vi "TLB Native Dynamic Events ver 0.19a.vi"() -> ()   [LabVIEW 2018]
uses:
  Labview Training Phase 2/Enum Controls/States for Action Engine.ctl
  TLB Type Definitions/State Type Definitions, for 0.26g versions and later 2.ctl
  TLB Type Definitions/Intruction Type Definitions.ctl
  TLB Type Definitions/Encoder cluster.ctl
  TLB Type Definitions/PING CLUSTER.ctl
  <vilib>/Studica/Studica Toolkit/NavX/NavX.lvlib
  <vilib>/Studica/Studica Toolkit/Background/DIO Channel.ctl
  Underlying VI's/NavX VI/navX type def.ctl
  <vilib>/Studica/Studica Toolkit/Background/I2C Channel.ctl
  TLB Type Definitions/Vision cluster.ctl
  <vilib>/NI_Real-Time Target Support.lvlib
  TLB Type Definitions/Stepper cluster.ctl
  Experimental VI's/Archived VI's/MOTOR CONTROL NO PID Type Def.ctl
  Underlying VI's/I2C Master VI/I2C MASTER Type Def.ctl
  Underlying VI's/I2C Master VI/I2C_MASTER_WRITE_NEW Type Def.ctl
  <vilib>/userdefined/High Color/IMAQdx.ctl
  Underlying VI's/I2C Master VI/Arduino_Interfacing.ctl
  TLB Type Definitions/Yaw Cluster.ctl
  TLB Type Definitions/Time cluster.ctl
  TLB Type Definitions/Y Stepper cluster.ctl
  Underlying VI's/Modified webcam FGV/Webcam AE.ctl
  Underlying VI's/Elasped Timer/Elapsed timer control.ctl
  Underlying VI's/Motor Control VI with PID/MOTOR CONTROL WITH PID AE DATA MODE TYPE DEF.ctl
  Underlying VI's/Motor Control VI with PID/MOTOR CONTROL WITH PID AE DIRECTION TYPE DEF.ctl
  TLB Type Definitions/IR Sensor Type Def.ctl
  <vilib>/myRIO/Common/Instrument Driver Framework/myRIO v1.0/AI/typedefs/AI Channels Enum.ctl
  <vilib>/myRIO/Common/Instrument Driver Framework/myRIO v1.0/AI/typedefs/AI Channels List.ctl
  TLB Type Definitions/Motor Speed Cluster.ctl
  Underlying VI's/IMAQ Create Reference AE/IMAQ Reference AE.ctl
  TLB Type Definitions/Line Sensor Cluster.ctl
  Underlying VI's/Line Sensor AE/Line Sensor AE Type Def.ctl
  <vilib>/Utility/RT CPU Load.ctl
  <vilib>/Studica/Studica Toolkit/NavX/TypeDefs/Flags/Z900_navX_Flags_CalibrationStatusTypeDef.ctl
  <vilib>/Studica/Studica Toolkit/NavX/TypeDefs/Flags/Z900_navX_Flags_OpStatusTypeDef.ctl
panel:
  out "Distance reached?":bool
  out "Correcte stepper":u8
  out "Image Processing Error":errorcluster
  out "Object Detection":T1
  out "Status":T4 {"OP Status" items=["INITIALIZING", "SELFTEST_IN_PROGRESS", "ERROR", "IMU_AUTOCAL_IN_PROGRESS", "NORMAL"]; "Calibration Status" items=["IMU_CAL_STATE_MASK"=3, "IMU_CAL_STATE_INPROGRESS"=0, "IMU_CAL_STATE_ACCUMULATE"=1, "IMU_CAL_STATE_COMPLETE"=2]}
  out "General Errors":errorcluster
  in  "Red LED":bool
  out "Arm IR Sensor":dbl
  out "Table obstruct":bool
  out "x-y":dbl
  out "Left IR Sensor":dbl
  out "Obstacle detected":bool
  out "Speed & distance":T5
  out "Time up flag":bool
  out "Task selection":u8
  in  "Object recognition mode":enum16{"Ball", "Soap", "Gel", "Pipe", "None"}(ring)
  out "NavX Readings":T6
  out "Arduino Data":T7
  out "CPU loads":T8[](array[typedef]) {"ISR (%)" format="%#.2f"; "Idle (%)" format="%#.2f"; "Background (%)" format="%#.2f"; "Normal (%)" format="%#.2f"; "Above Normal (%)" format="%#.2f"; "High (%)" format="%#.2g"; "Timed Structures (%)" format="%#.2g"; "Time Critical (%)" format="%#.2g"; "Total (%)" format="%#.2g"}
  out "TASK ENABLE":bool
  out "Rising Edge":bool
  in  "Green LED":bool
  out "State Logic":T9=enum."Startup"
  out "elements":T10[](array[typedef])
  in  "STOP TASK":bool
  in  "OK Button":bool
  in  "STOP":bool
  out "Queue Errors":errorcluster
  out "Action Queue Items":i32
  out "State Logic Queue Items":i32
  out "Action Queues items":string[](array[string])=["Hardware reset", "Software reset", ""]
  out "Action State":string
  # "System Health Status Update"
  # "VISION"
  # "TLB FRAMEWORK STATUS"
  # "Test Programme written by Calvin Loke    Dated: 28 Aug 2019\nTest Programme revised by Dr Alex See   Dated 30 Aug 2019\n\nRevision date: 20/03/2020\nProgramme version:   TLB Native Dynamic Events ver 0.19a"
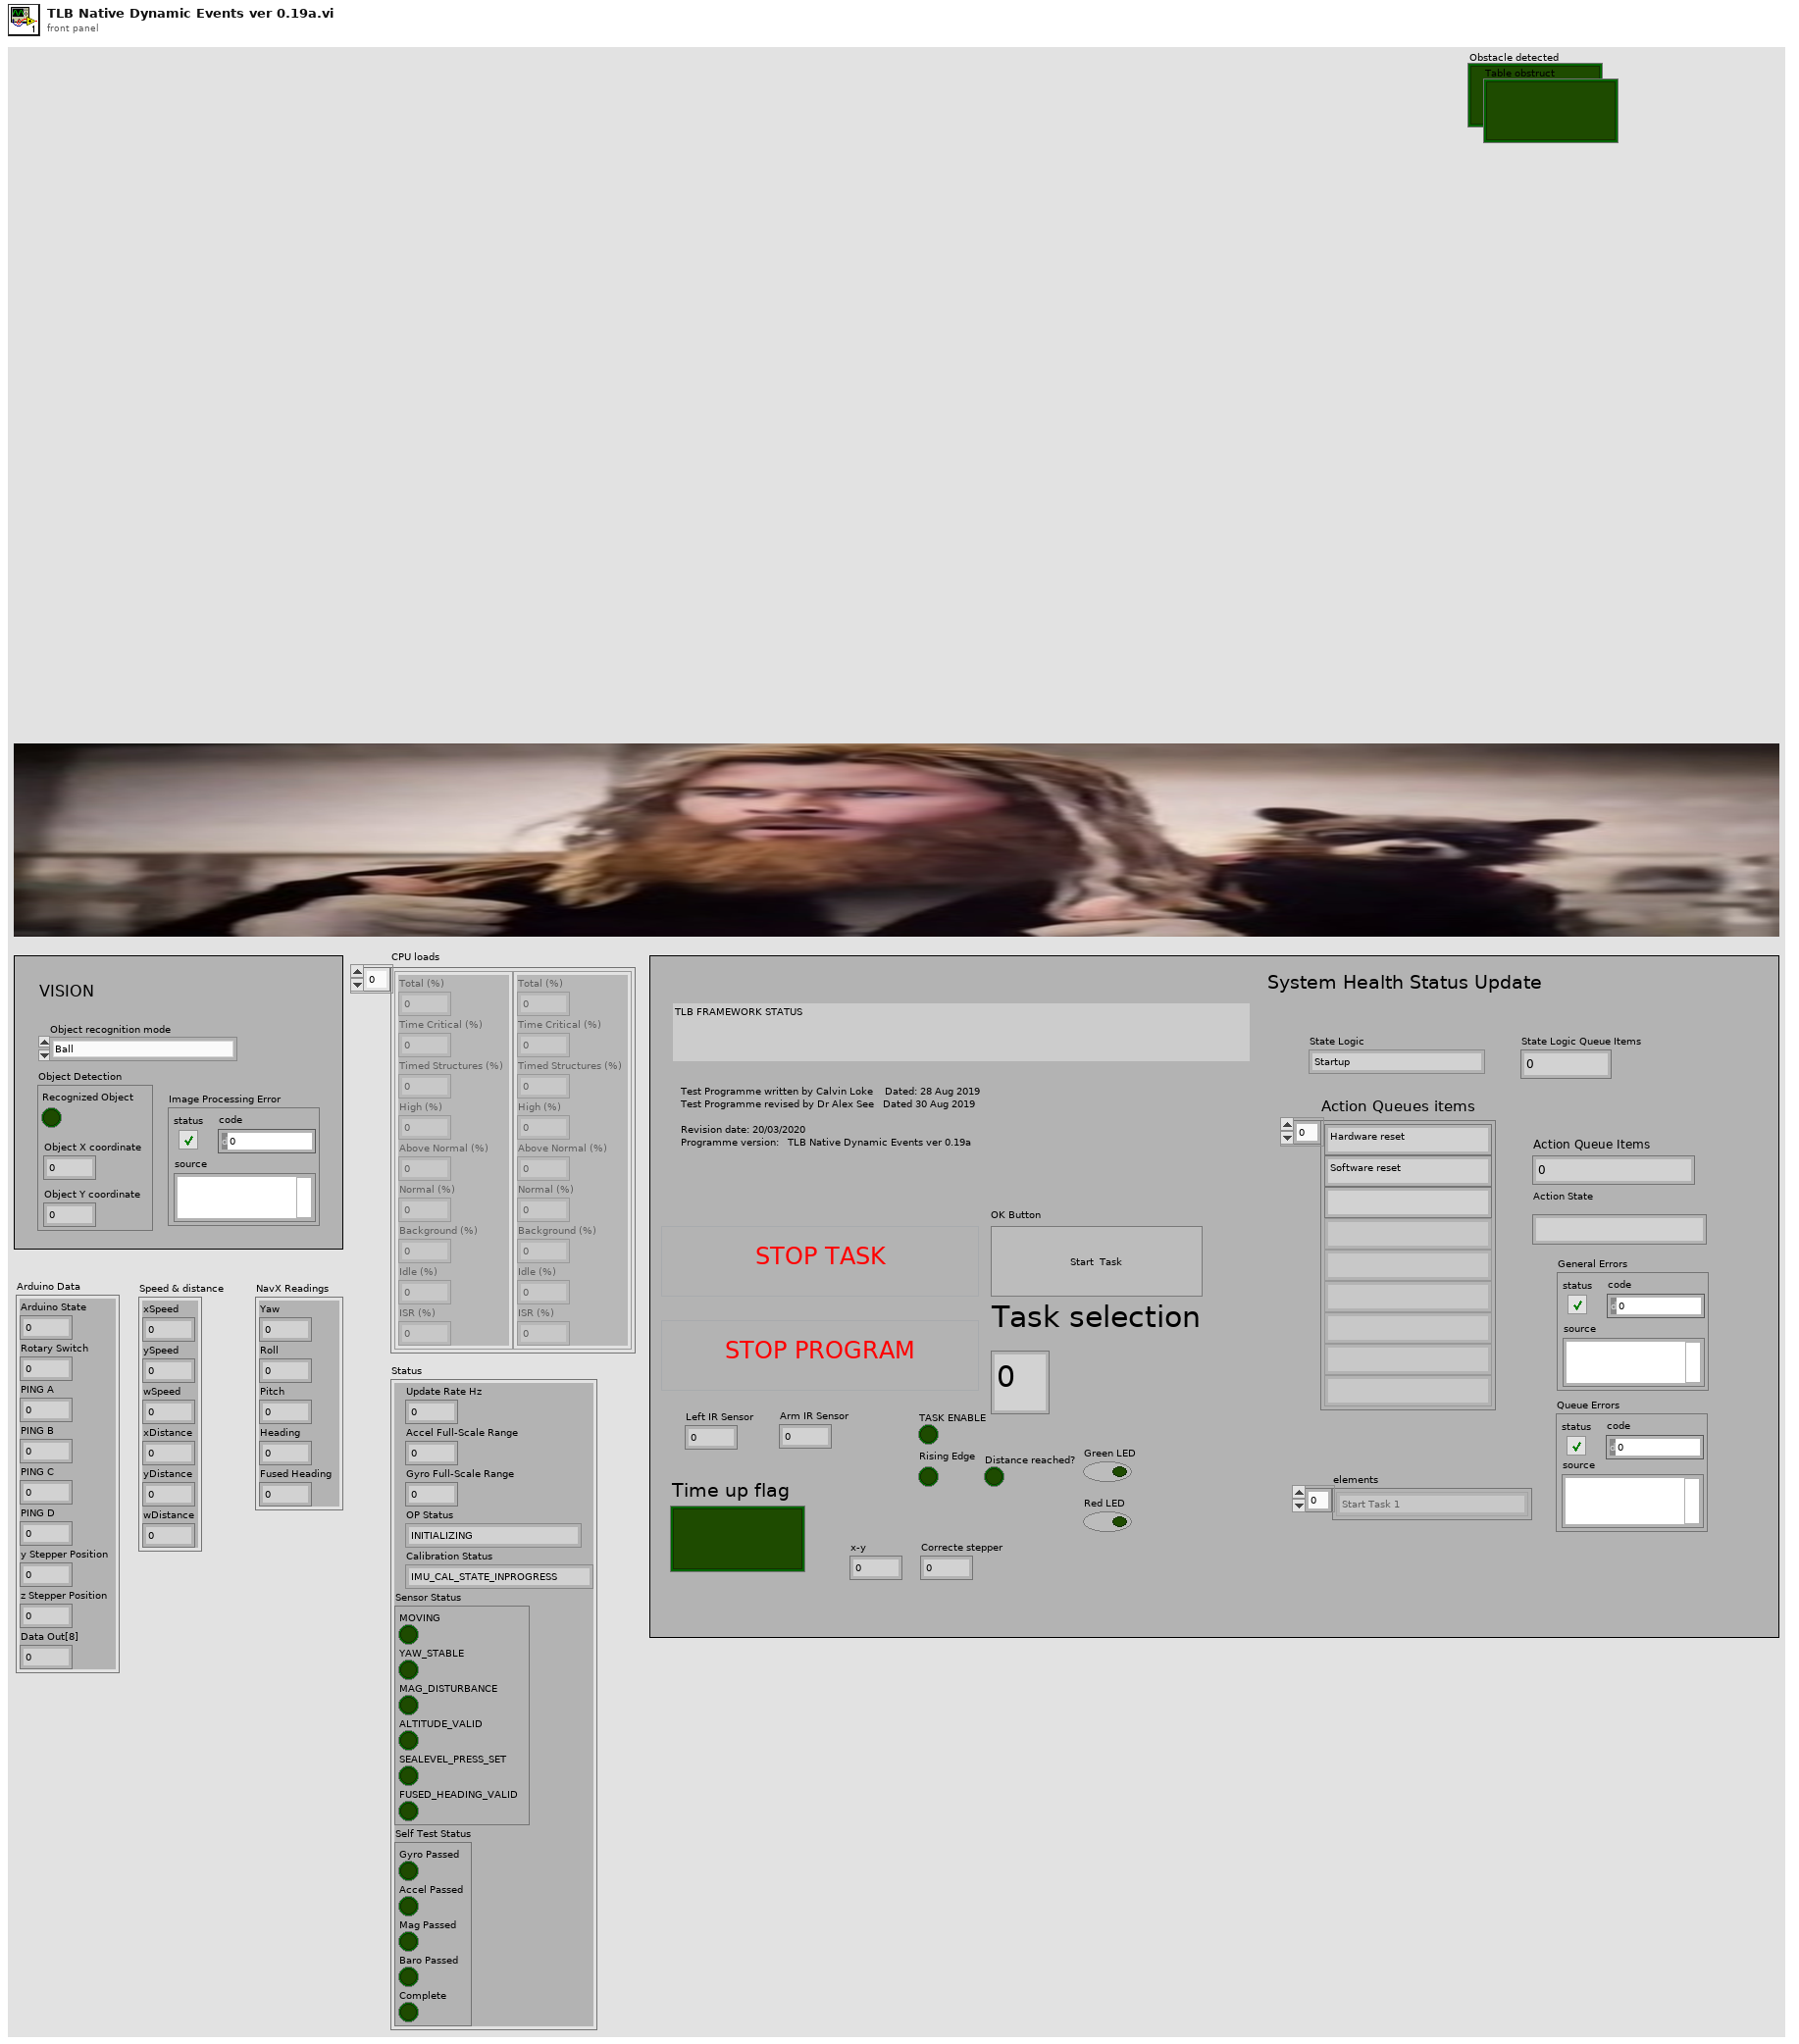
[diagram p1: front panel]
types:
  T1 = typedef "Vision cluster.ctl" = cluster{"Recognized Object":bool, "Object X coordinate":dbl, "Object Y coordinate":dbl}
  T2 = typedef "NavX.lvlib/Z900_navX_Flags_OpStatusTypeDef.ctl" = u8
  T3 = typedef "NavX.lvlib/Z900_navX_Flags_CalibrationStatusTypeDef.ctl" = u8
  T4 = cluster{"Update Rate Hz":u8, "Accel Full-Scale Range":u8, "Gyro Full-Scale Range":u16, "OP Status":T2, "Calibration Status":T3, "Sensor Status":cluster{"MOVING":bool, "YAW_STABLE":bool, "MAG_DISTURBANCE":bool, "ALTITUDE_VALID":bool, "SEALEVEL_PRESS_SET":bool, "FUSED_HEADING_VALID":bool}, "Self Test Status":cluster{"Gyro Passed":bool, "Accel Passed":bool, "Mag Passed":bool, "Baro Passed":bool, "Complete":bool}}
  T5 = cluster{"xSpeed":dbl, "ySpeed":dbl, "wSpeed":dbl, "xDistance":dbl, "yDistance":dbl, "wDistance":dbl}
  T6 = cluster{"Yaw":dbl, "Roll":dbl, "Pitch":dbl, "Heading":dbl, "Fused Heading":dbl}
  T7 = cluster{"Arduino State":u8, "Rotary Switch":u8, "PING A":u8, "PING B":u8, "PING C":u8, "PING D":u8, "y Stepper Position":u8, "z Stepper Position":u8, "Data Out[8]":u8}
  T8 = typedef "NI_Real-Time Target Support.lvlib/RT CPU Load.ctl" = cluster{"Total (%)":dbl, "Time Critical (%)":dbl, "Timed Structures (%)":dbl, "High (%)":dbl, "Above Normal (%)":dbl, "Normal (%)":dbl, "Background (%)":dbl, "Idle (%)":dbl, "ISR (%)":dbl}
  T9 = typedef "State Type Definitions, for 0.26g versions and later 2.ctl" = enum16{"None", "Startup", "Move to Angle", "True Stop", "Idle", "Shutdown", "Task 1A", "Task 1B", "Task 2:Raise Arm", "Task 2:Sensor Mode", "Task 2:Reverse Mode", "Task 3", "Task 4_A", "Task 4_B", "Task 4_C", "Task 4_D", "Task 5A", "Task 5B", "Task 5C", "Task 5D", "Task 5E: POSITION ARM", "Task 5F: ARM GRAB HEIGHT", "Task 5G: CLOSE CLAW", "Task 5H: RAISE ARM", "Task 6_A", "Task 6_B", "Task 7", "Task 8A: RAISE ARM", "Task 8B: MOVE TO BOX", "Task 8C: CAM BURST", "Task 8D: PROCESS IMAGE", "Task 8E: ROBOT ADJUST", "Task 8F: CAM BURST 2", "Task 8G: PROCESS IMAGE 2", "Task 8H: ARM ADJUST", "Task 8I: ARM GRAB HEIGHT", "Task 8J: CLOSE CLAW", "Task 8K: RAISE MY SWORD", "Task 9A: Raise Arm", "Task 9B: Rotate to Angle", "Task 9C: Detect Box", "Task 9D: MOVE FORWARD", "Task 9E: MOVE LEFT", "Task 9F: SCAN BOX", "Task 9G: MOVE RIGHT", "Task 9H: SCAN BOX 2", "Task 9I: ROTATE 90 CW", "Task 9J: FORWARD", "Task 9K: MOVE RIGHT", "Task 9L: SCAN BOX 3", "Task 9M: MOVE RIGHT", "Task 9N: SCAN BOX 4", "PENIS", "PENIS 2", "PENIS 3", "Task 9R: PROCESS COLOUR", "Task A1: Task 9 Open cam", "Task A2: Task 9 Move Arm", "Task A3: Task 9 Set Timer", "Task A4: Tasl 9 Capture images", "Task A5: Task 9 Close camera", "Task A6: Process Colour", "Task A7: Dispose Camera Buffer"}
  T10 = typedef "Intruction Type Definitions.ctl" = enum16{"None", "Start Task 1", "Start Task 2", "Start Task 3", "Start Task 4", "Start Task 5", "Start Task 6", "Start Task 7", "Start Task 8 - BALL", "Start Task 8 - Gel", "Start Task 8 - Pipe", "Start Task 8 - Soap", "Start Task 9", "Start Task A", "Start Task B", "Exit"}
  T11 = typedef "Line Sensor Cluster.ctl" = cluster{"Line Detected?":bool, "S1":dbl, "S2":dbl, "S3":dbl, "S4":dbl}
  T12 = typedef "Motor Speed Cluster.ctl" = cluster{"ySpeed":dbl, "xSpeed":dbl, "wSpeed":dbl}
  T13 = typedef "IR Sensor Type Def.ctl" = cluster{"Left IR Sensor":dbl, "Arm IR Sensor":dbl, "Bottom IR Sensor":dbl}
  T14 = typedef "Y Stepper cluster.ctl" = cluster{"yStepper desired":u8}
  T15 = typedef "Time cluster.ctl" = cluster{"Time up flag":bool, "SET TIME TO CHECK":dbl}
  T16 = typedef "Yaw Cluster.ctl" = cluster{"Yaw":dbl, "Compass":dbl}
  T17 = typedef "Stepper cluster.ctl" = cluster{"y Stepper Position":u8, "z Stepper Position":u8}
  T18 = typedef "DIO Channel.ctl" = enum16{"Not Connected", "A/DIO1", "A/DIO2", "A/DIO3", "A/DIO4", "A/DIO5", "A/DIO6", "A/DIO7", "A/DIO13", "B/DIO1", "B/DIO2", "B/DIO3", "B/DIO4", "B/DIO5", "B/DIO6", "B/DIO7", "B/DIO13", "C/DIO0", "C/DIO1", "C/DIO2", "C/DIO3", "C/DIO4", "C/DIO5", "C/DIO6", "C/DIO7"}
  T19 = typedef "PING CLUSTER.ctl" = cluster{"PING_A":u8, "PING_B":u8, "PING_C":u8, "PING_D":u8}
  T20 = typedef "Encoder cluster.ctl" = cluster{"xDistance":dbl, "yDistance":dbl, "wDistance":dbl}
  T21 = cluster{"DIO Channel":T18, "FPGA VI Reference Out":refnum<k20>}
  T22 = typedef "navX type def.ctl" = enum16{"Get i2C reference", "Read Values", "Zero Yaw"}
  T23 = typedef "Arduino_Interfacing.ctl" = enum16{"Initialize", "Write to Arduino", "Read From Arduino"}
  T24 = typedef "I2C Channel.ctl" = enum16{"Not Connected", "A", "B"}
  T25 = typedef "States for Action Engine.ctl" = enum16{"Initialize", "Write", "Read"}
  T26 = cluster{"I2C Ref Out":cluster{"I2C Channel":T24, "FPGA VI Reference Out":refnum<k20>}, "Connected":bool, "Slave Address (7-bit)":u8, "Registry":u8[]}
  T27 = typedef "State Type Definitions.ctl" = enum16{"None", "Startup", "Move to Angle", "True Stop", "Idle", "Shutdown", "Task 1", "Task 2:Raise Arm", "Task 2:Sensor Mode", "Task 2:Reverse Mode", "Task 3", "Task 4_A", "Task 4_B", "Task 4_C", "Task 4_D", "Task 5A: ARM CAM HEIGHT", "Task 5B: MOVE TO BOX", "Task 5C: CAM BURST", "Task 5D: PROCESS IMAGE", "Task 5E: POSITION ARM", "Task 5F: ARM GRAB HEIGHT", "Task 5G: CLOSE CLAW", "Task 5H: RAISE ARM", "Task 6_A", "Task 6_B", "Task 7", "Task 8A: RAISE ARM", "Task 8B: MOVE TO BOX", "Task 8C: CAM BURST", "Task 8D: PROCESS IMAGE", "Task 8E: ROBOT ADJUST", "Task 8F: CAM BURST 2", "Task 8G: PROCESS IMAGE 2", "Task 8H: ARM ADJUST", "Task 8I: ARM GRAB HEIGHT", "Task 8J: CLOSE CLAW", "Task 8K: RAISE MY SWORD", "Task 9A: Raise Arm", "Task 9B: Rotate to Angle", "Task 9C: Rotation alignmnet", "Task 9D: Move Forward", "Task 9E: MOVE LEFT", "Task A: RAISE ARM TO HEIGHT", "Task A: MOVE FORWARD"}
  T28 = typedef "MOTOR CONTROL WITH PID AE DIRECTION TYPE DEF.ctl" = enum16{"y-axis movement", "x-axis movement", "rotation", "stop", "reset encoders"}
  T29 = typedef "MOTOR CONTROL WITH PID AE DATA MODE TYPE DEF.ctl" = enum16{"Init AE", "Write to AE", "Read from AE"}
  T30 = typedef "Line Sensor AE Type Def.ctl" = enum16{"INIT AE", "READ FROM LINE SENSORS"}
  T31 = typedef "IMAQ Reference AE.ctl" = enum16{"Initialize AE", "Get IMAQ Reference", "Dispose Processing Buffer"}
  T32 = typedef "Elapsed timer control.ctl" = enum16{"Start", "Pause", "Initialize"}
  T33 = typedef "I2C_MASTER_WRITE_NEW Type Def.ctl" = enum16{"Ultrasonic sensors", "Stepper origin", "zStepper 13.3k", "zStepper 13k", "zStepper 12k", "zStepper 11k", "zStepper 10k", "zStepper 9k", "zStepper 8k", "zStepper 7k", "zStepper 6k", "zStepper 5k", "zStepper 4k", "zStepper 3k", "zStepper 2k", "zStepper 1k", "zStepper 900", "zStepper 800", "zStepper 700", "zStepper 600", "zStepper 500", "zStepper 400", "zStepper 300", "zStepper 200", "zStepper 100", "zStepper 0", "yStepper control", "Open Claw", "Close Claw", "Soft Reset"}
  T34 = typedef "Webcam AE.ctl" = enum16{"Initialize Camera", "Open Camera", "Continuous Acquisition", "Close Camera", "Retrieve Image", "Dispose Camera Image Buffer"}
  T35 = typedef "IMAQdx.ctl" = refnum<k21>
  T36 = typedef "MOTOR CONTROL NO PID Type Def.ctl" = enum16{"Init", "Front Back", "Left Right", "Rotate", "Stop", "Latch"}
  T37 = typedef "AI Channels List.ctl" = T38[]
  T38 = typedef "AI Channels Enum.ctl" = enum16{"Not Connected", "AudioIn/Left", "AudioIn/Right", "C/AI0", "C/AI1", "A/AI0", "A/AI1", "A/AI2", "A/AI3", "A/AI4", "A/AI5", "A/AI6", "A/AI7", "B/AI0", "B/AI1", "B/AI2", "B/AI3", "B/AI4", "B/AI5", "B/AI6", "B/AI7", "AI/AI0", "AI/AI1", "AI/AI2", "AI/AI3", "A/AI0 (DIFF)", "A/AI1 (DIFF)", "A/AI2 (DIFF)", "A/AI3 (DIFF)", "B/AI0 (DIFF)", "B/AI1 (DIFF)", "B/AI2 (DIFF)", "B/AI3 (DIFF)"}
  T39 = cluster{"S1":dbl, "S2":dbl, "S3":dbl, "S4":dbl, "Array[4]":dbl, "Array[5]":dbl, "Array[6]":dbl, "Array[7]":dbl, "Array[8]":dbl}
  T40 = typedef "I2C MASTER Type Def.ctl" = enum16{"Last State", "Mode 0", "Mode 1", "Mode 2", "Mode 3", "Mode 4", "Mode 5", "Mode 6", "Mode 7", "Mode 8", "Mode 9", "Mode 10"}
  T41 = typedef "IMAQ Image.ctl" = refnum<image>
  T42 = cluster{"Number of Matches":i32, "Object detected?":bool}
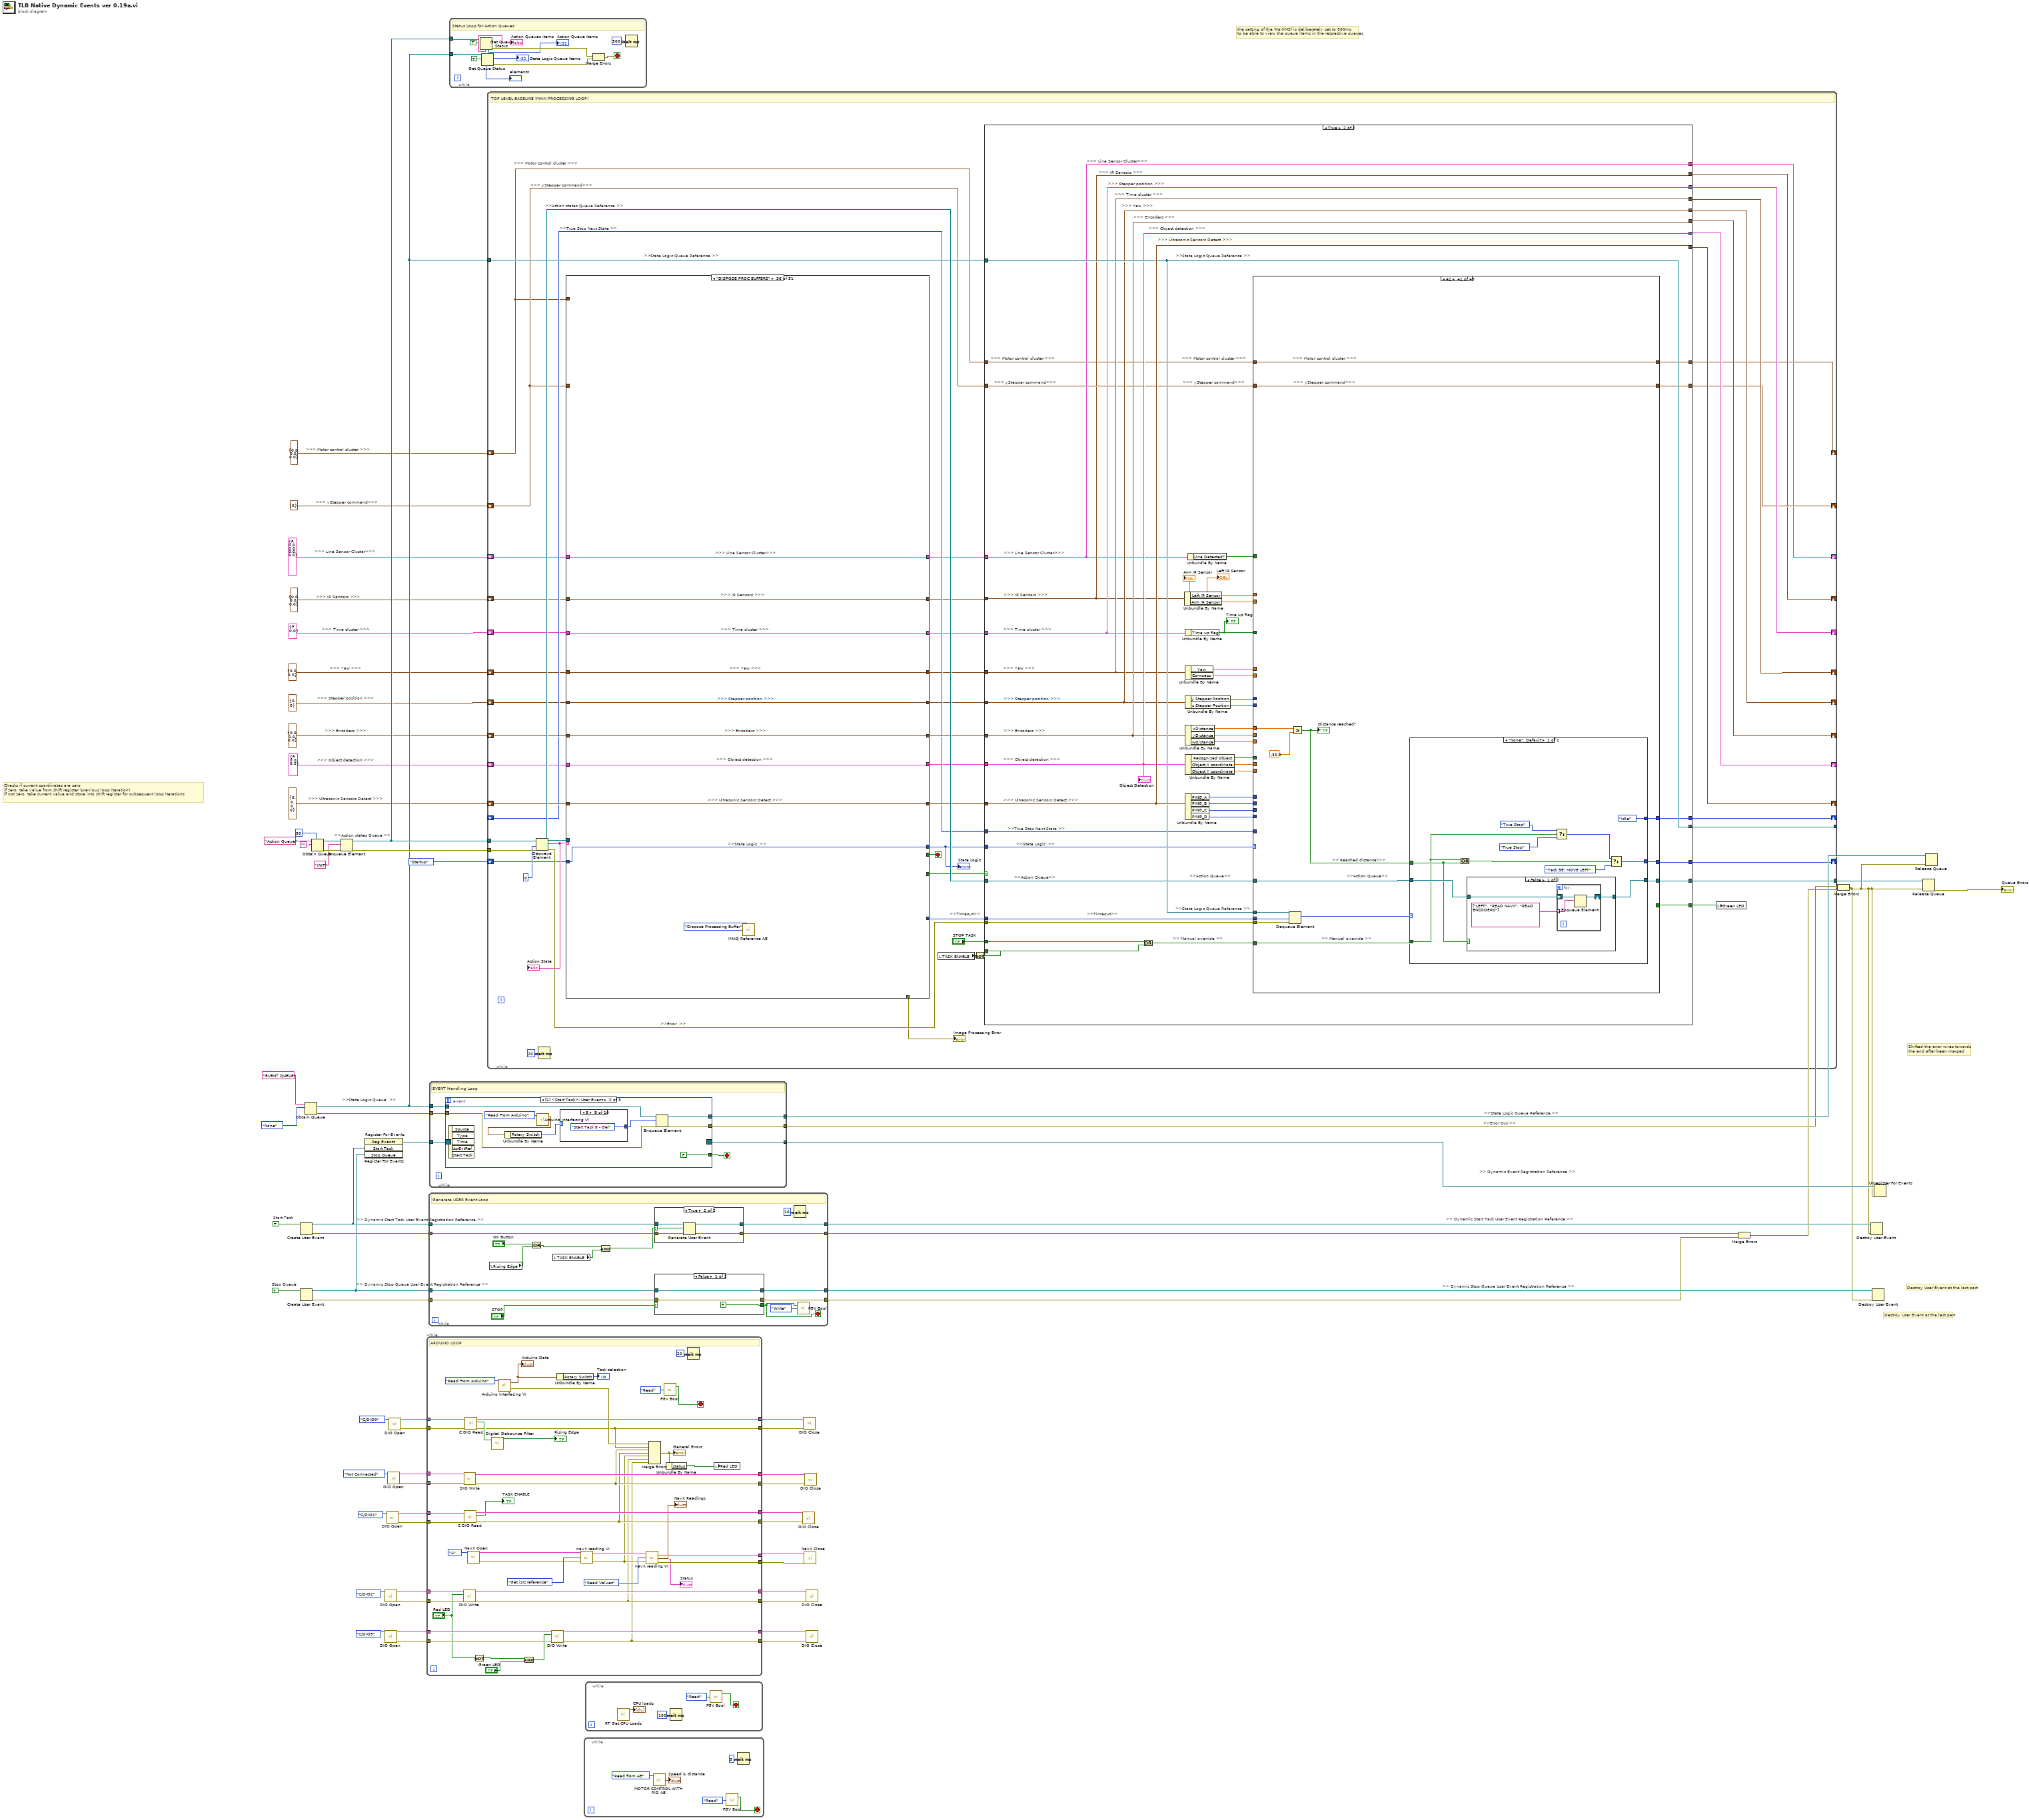
[diagram p0: block diagram]
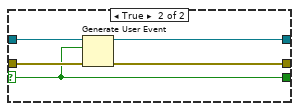
[diagram p2: hidden frame]
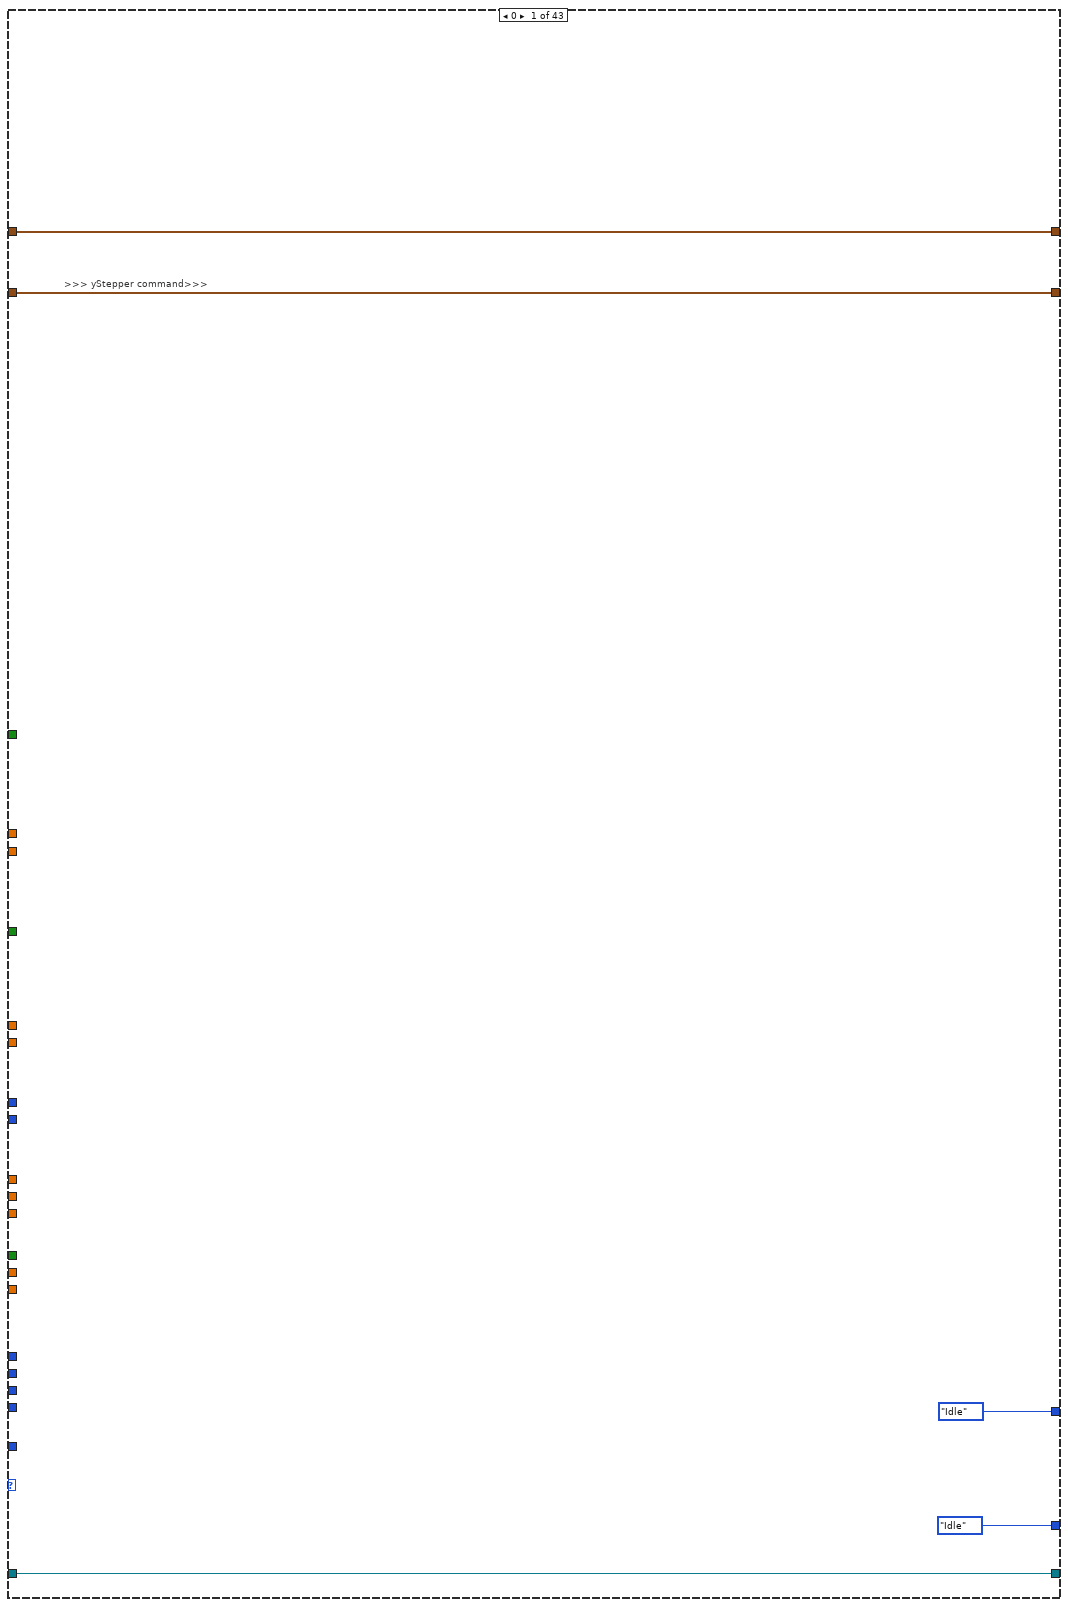
[diagram p5: hidden frame]
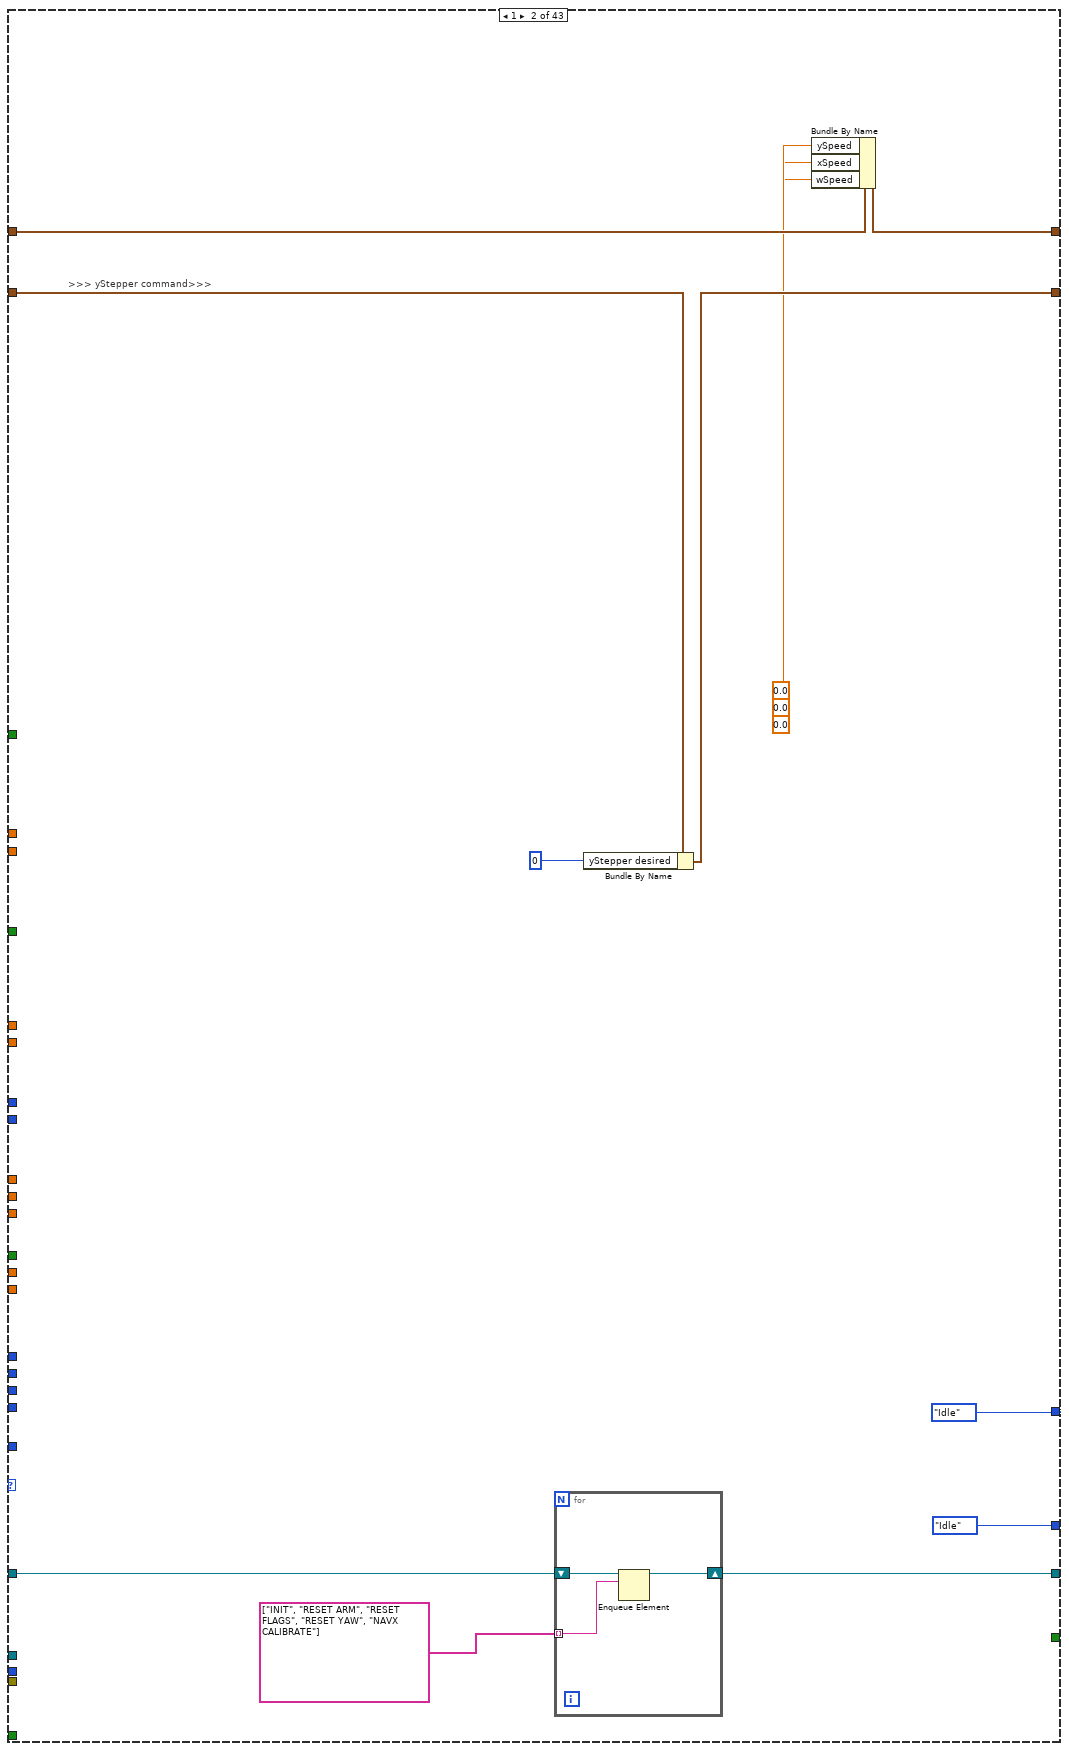
[diagram p6: hidden frame]
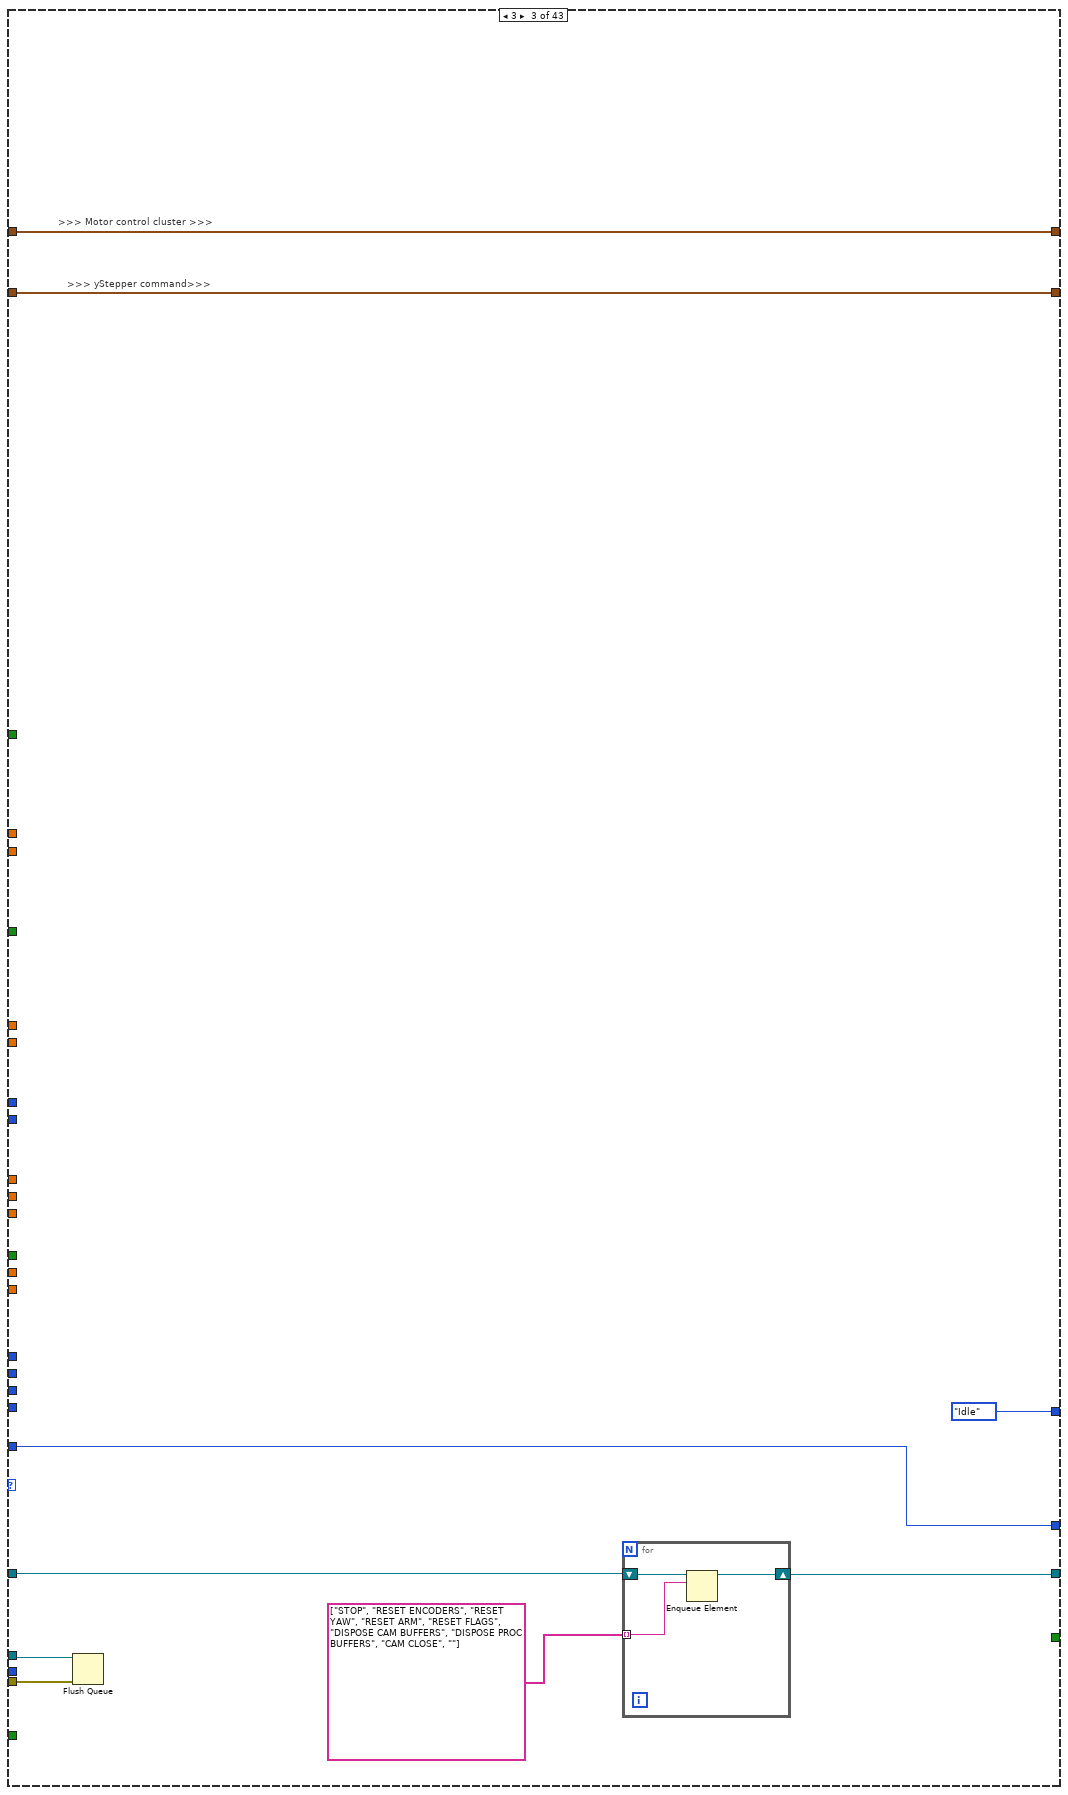
[diagram p7: hidden frame]
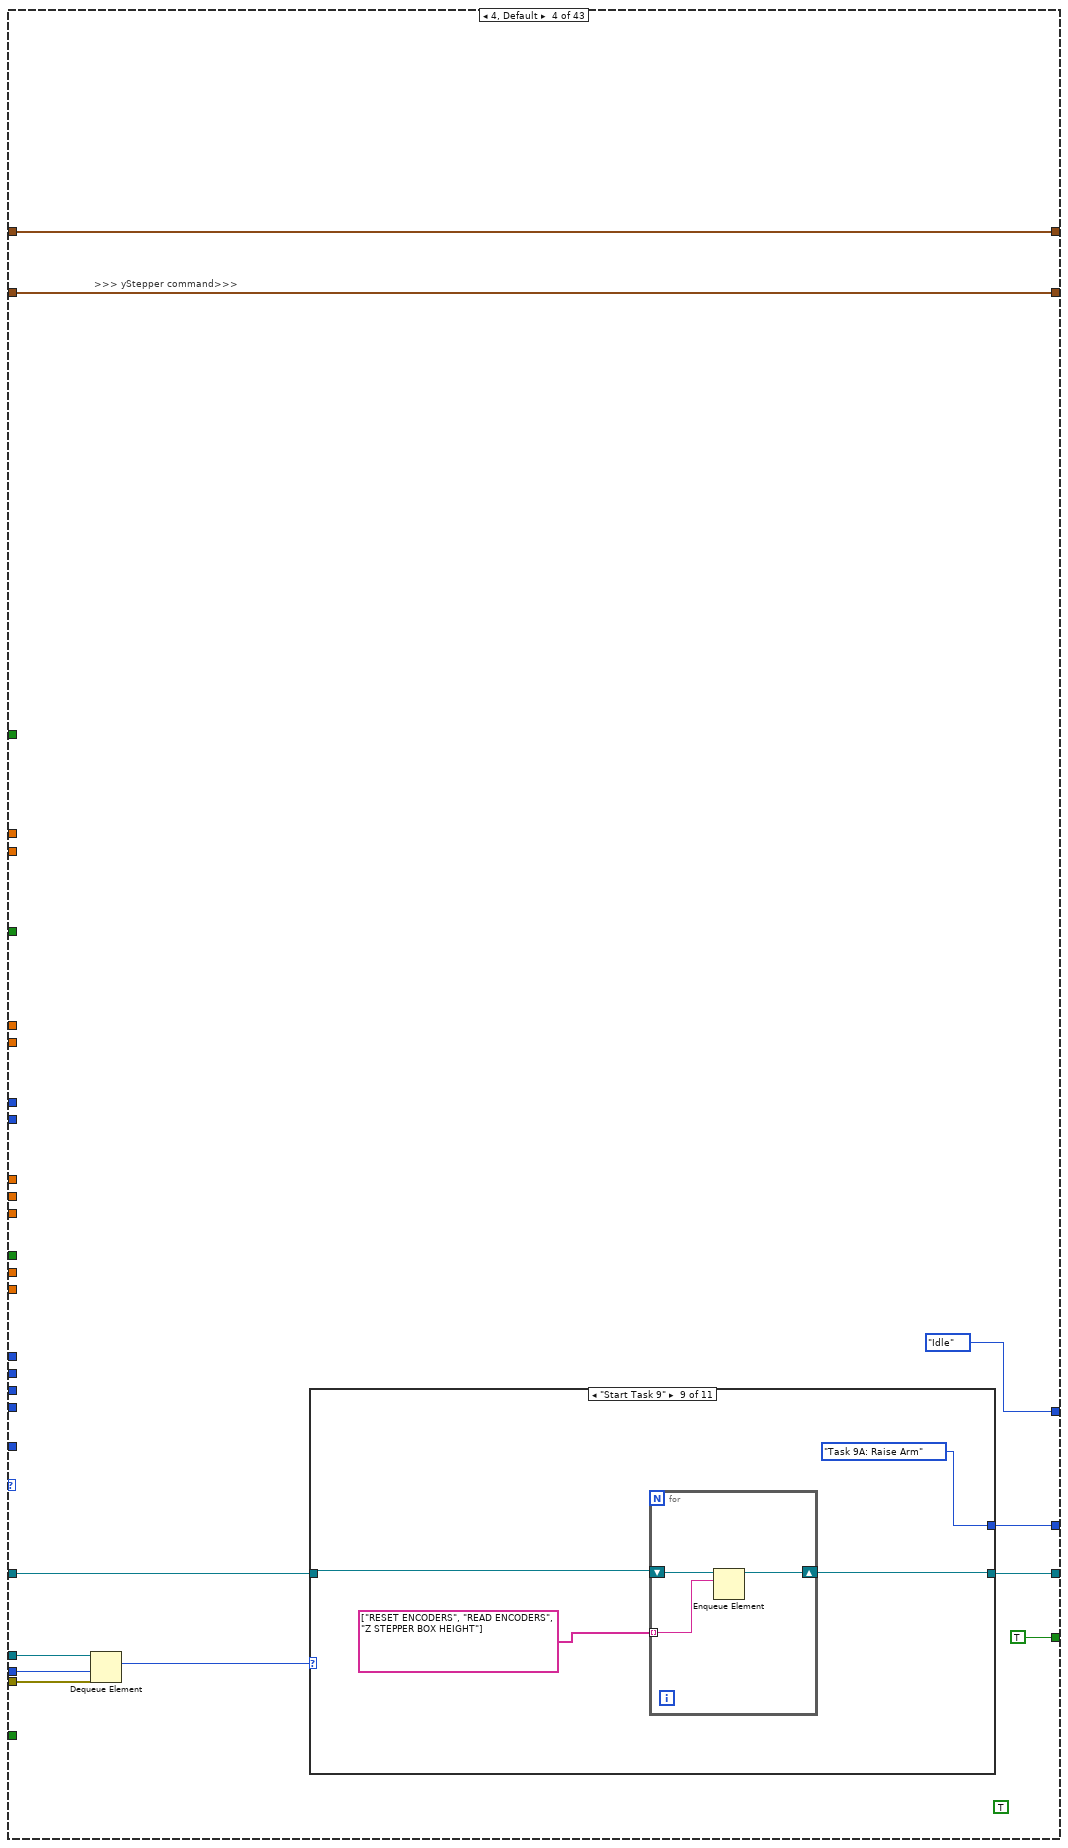
[diagram p8: hidden frame]
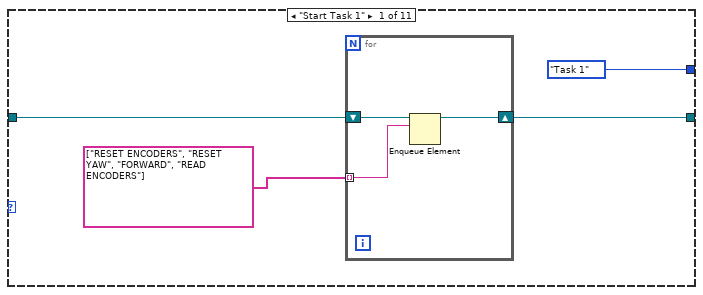
[diagram p9: hidden frame]
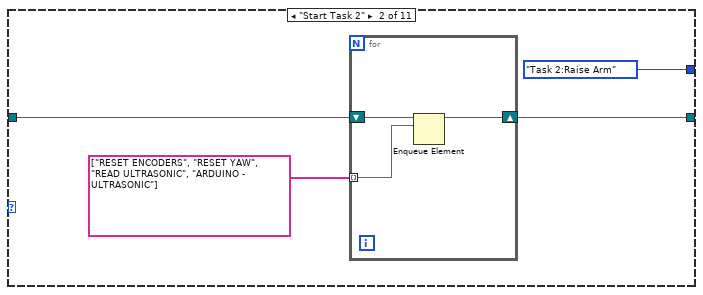
[diagram p10: hidden frame]
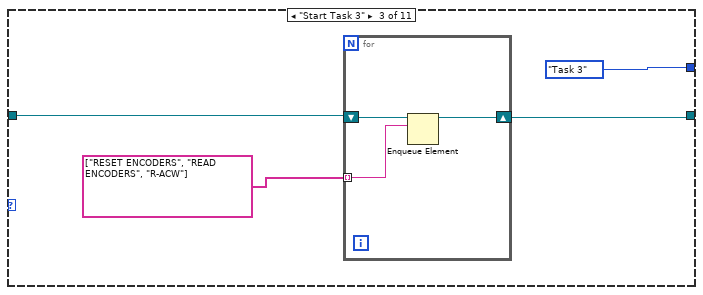
[diagram p11: hidden frame]
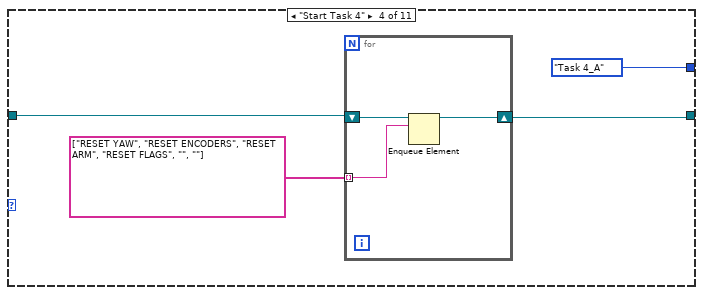
[diagram p12: hidden frame]
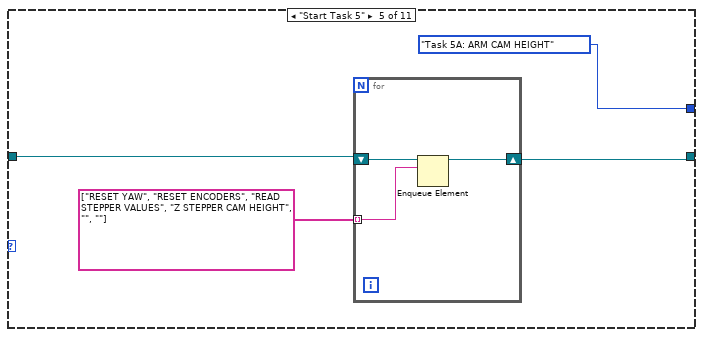
[diagram p13: hidden frame]
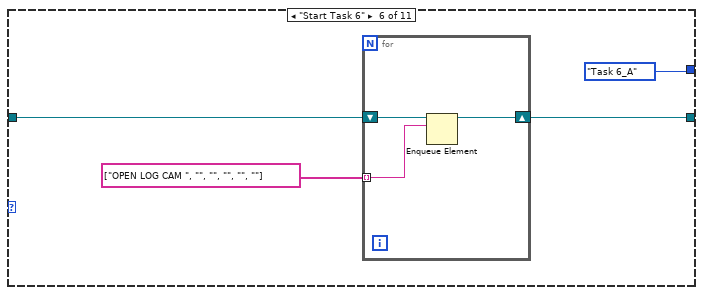
[diagram p14: hidden frame]
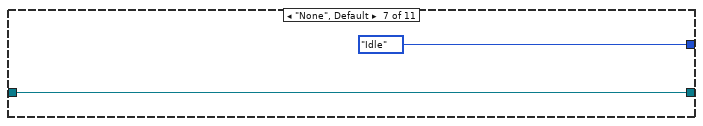
[diagram p15: hidden frame]
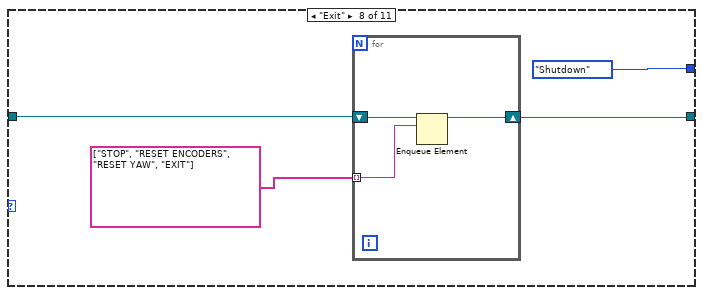
[diagram p16: hidden frame]
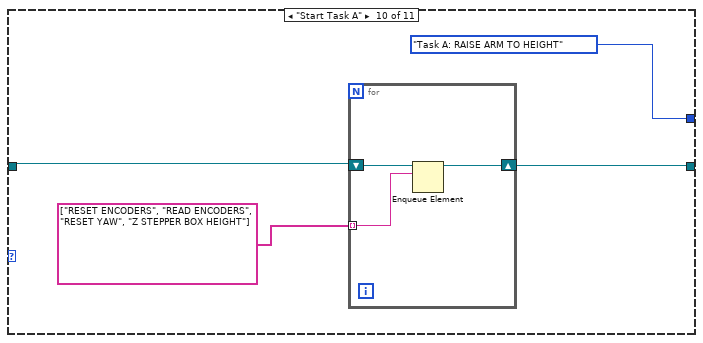
[diagram p17: hidden frame]
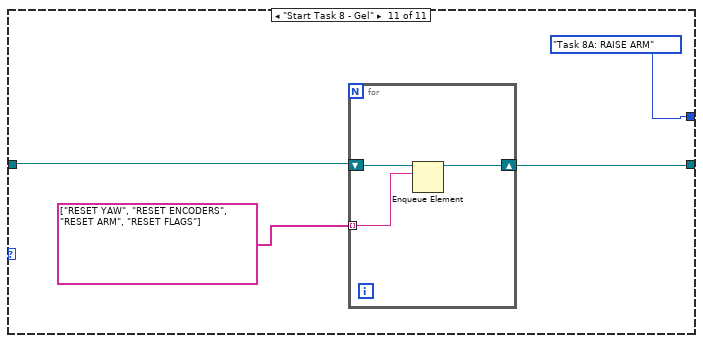
[diagram p18: hidden frame]
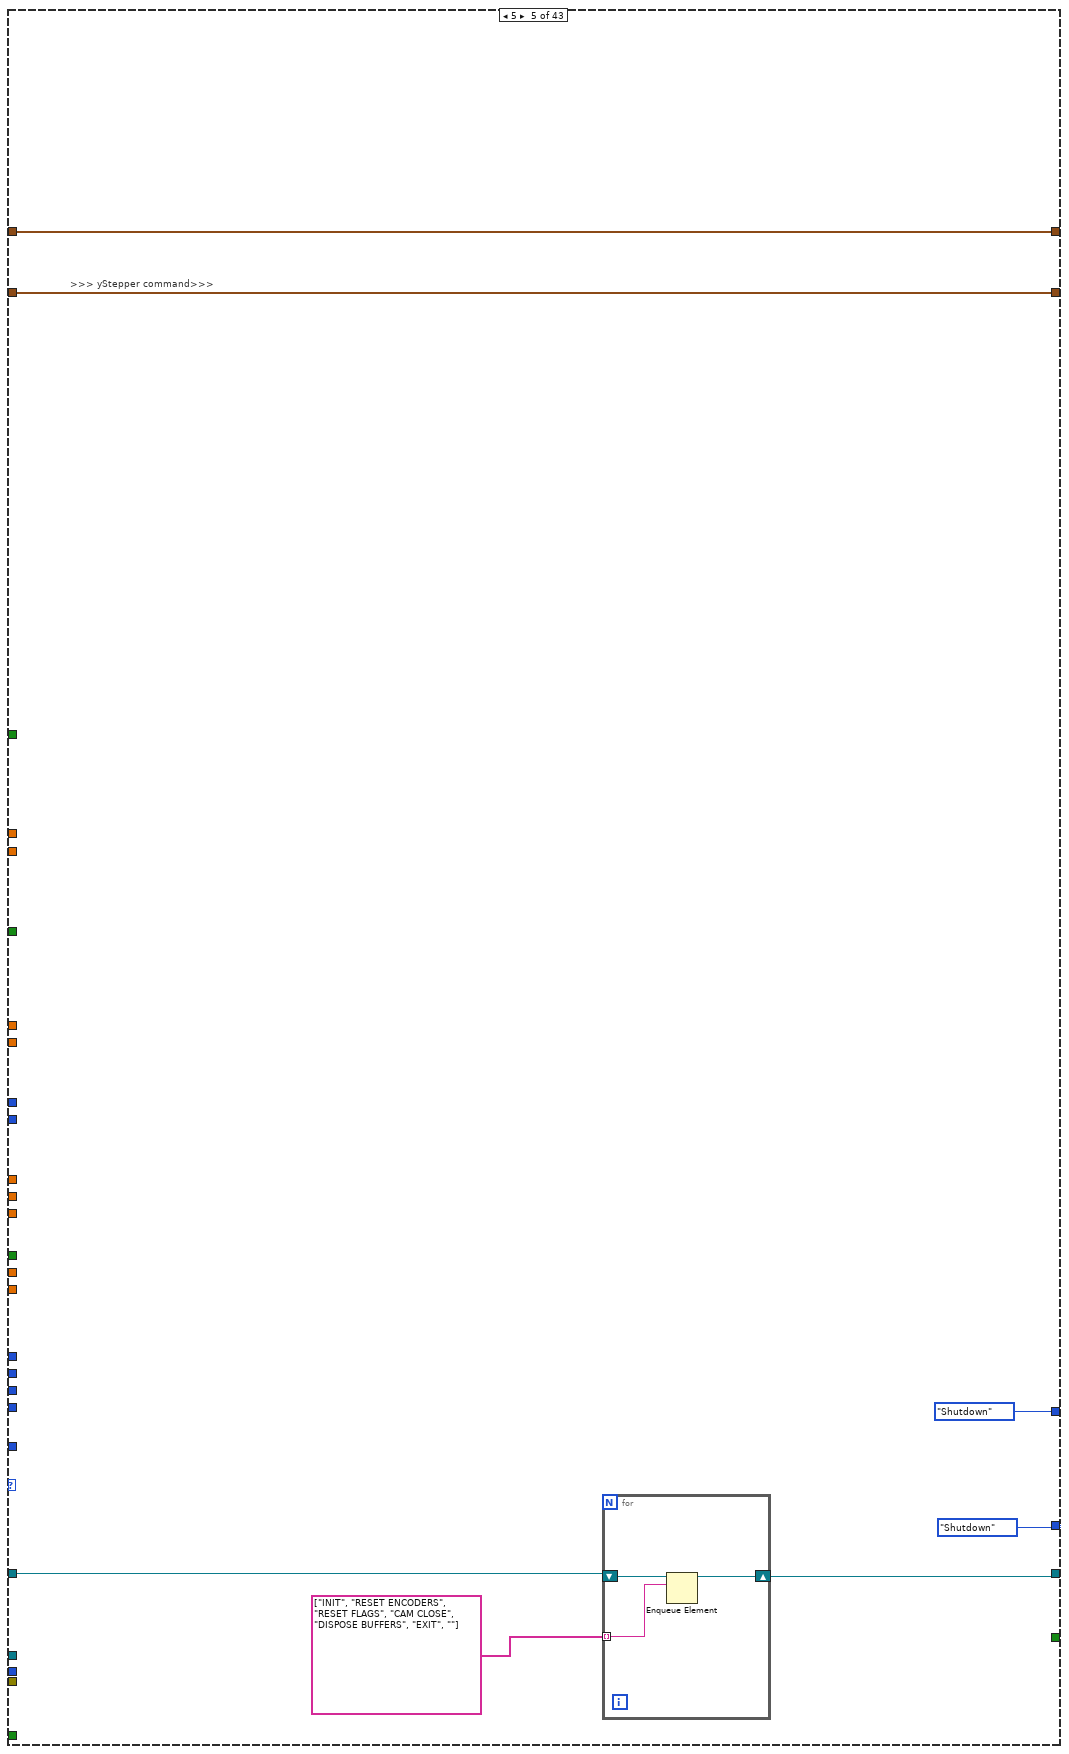
[diagram p19: hidden frame]
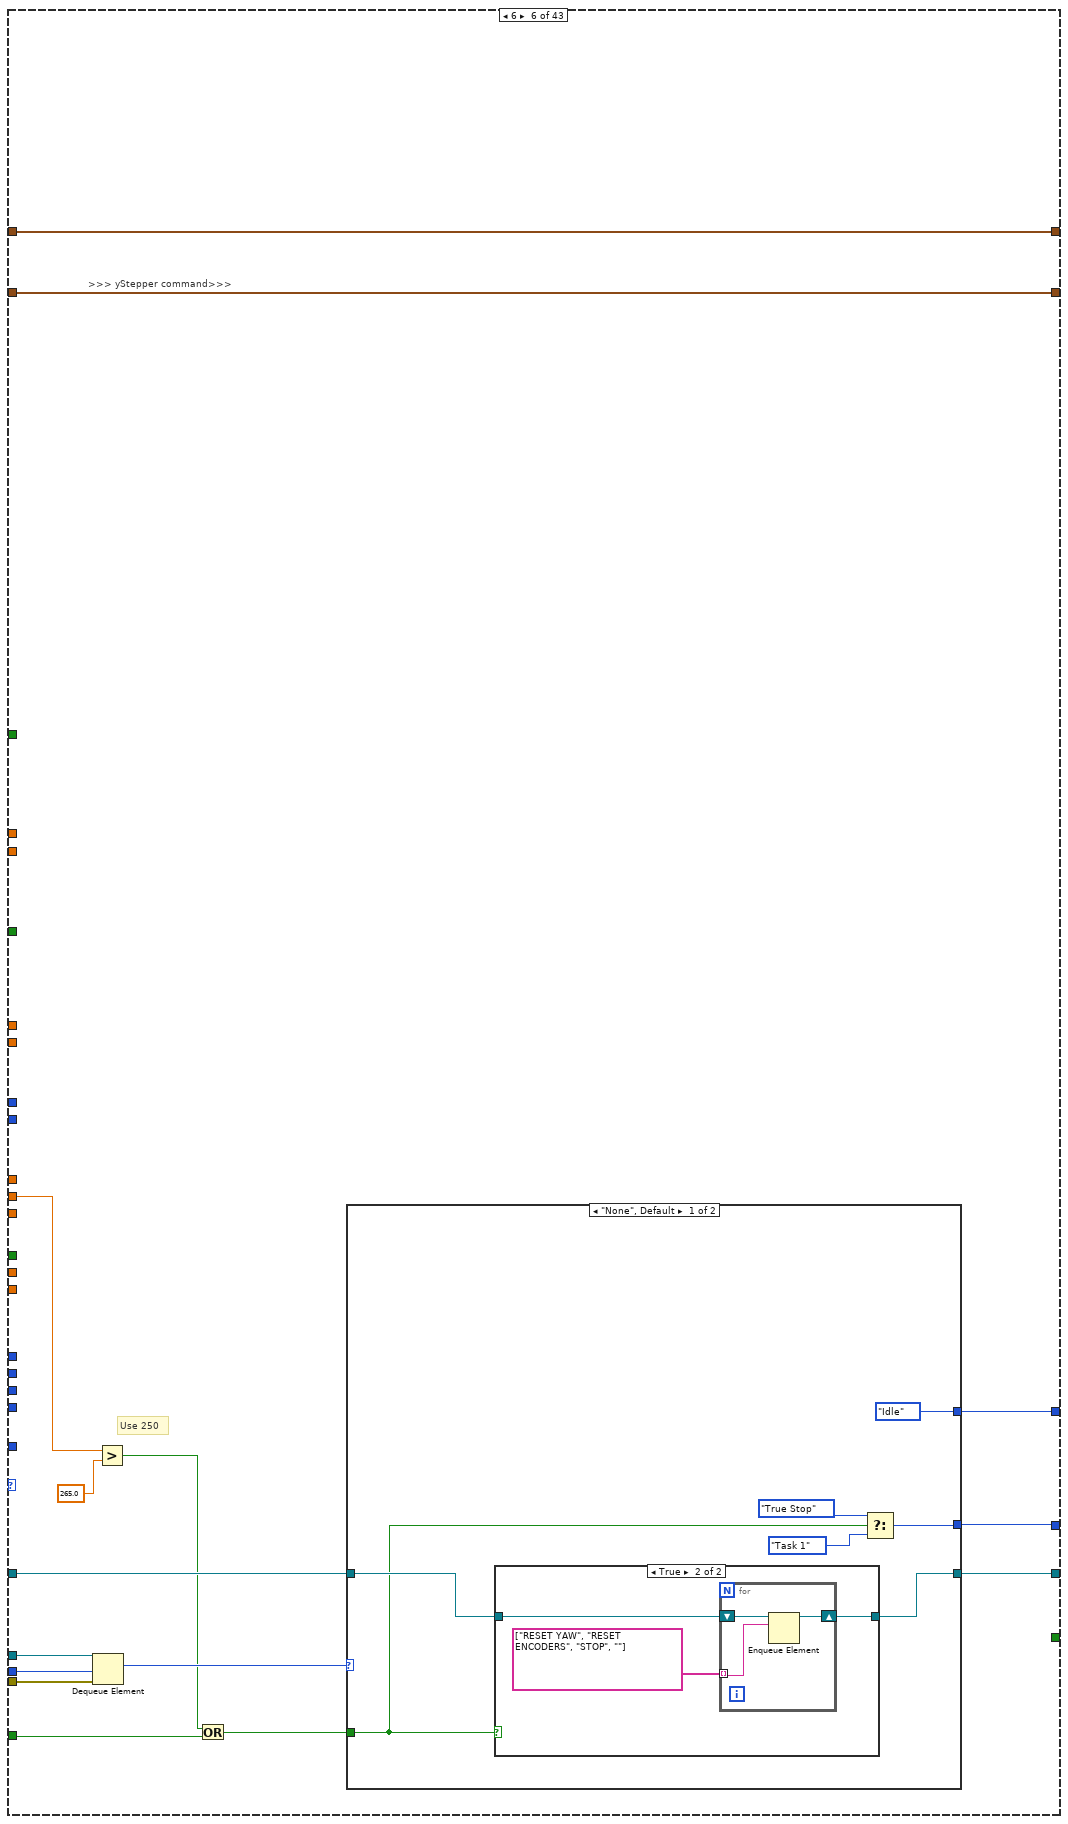
[diagram p20: hidden frame]
diagram:
  w68 = TRUE  # Stop Queue
  w67 = TRUE  # Start Task
  # ">>> Line Sensor Cluster>>>"
  # ">>> Motor control cluster >>>"
  # ">>> IR Sensors >>>"
  # "Checks if current coordinates are zero\nif zero, take value from shift register (previous loop iteration)\nif not zero, take current value and store into shift register for subsequent loop iterations"
  # ">>> yStepper command>>>"
  # ">>> Time cluster >>>"
  # ">>> Yaw >>>"
  # ">>> Stepper position >>>"
  # ">>> Encoders >>>"
  # ">>> Object detection >>>"
  # ">>> Ultrasonic Sensors Detect >>>"
  # "the setting of the Wait(MS) is deliberately set to 500ms\nto be able to view the queue items in the respective queues"
  # ">>Error Out >>"
  # ">> Dynamic Stop Queue User Event Registration Reference >>"
  # ">> Dynamic Start Task User Event Registration Reference >>"
  # ">> Dynamic Stop Queue User Event Registration Reference >>"
  # ">> Dynamic Start Task User Event Registration Reference >>"
  # ">> Dynamic Event Registration Reference >>"
  # ">>Action states Queue >>"
  # ">>State Logic Queue  >>"
  # ">>State Logic Queue Reference >>"
  # "Destroy User Event at the last part"
  # "Destroy User Event at the last part"
  # "Shifted the error wires towards\nthe end after been merged"
  n1 = Create User Event(user event datatype=w67) -> (user event=w59:refnum<user-event>, error out=w64:errorcluster)  [unwired: 1 in]
  n2 = Create User Event(user event datatype=w68) -> (user event=w60:refnum<user-event>, error out=w63:errorcluster)  [unwired: 1 in]
  n3 = Obtain Queue(name (unnamed)="EVENT QUEUE", element data type=Intruction_Type_Definitions."None" ("Enum")) -> (queue out=w45:refnum<queue>, error out=w51:errorcluster)  [unwired: 3 in, 1 out]
  n4 = Obtain Queue(max queue size (-1, unlimited)=50, name (unnamed)="Action Queue", element data type="") -> (queue out=w54:refnum<queue>, error out=w50:errorcluster)  [unwired: 2 in, 1 out]
  n5 = Enqueue Element(queue=w54, element="INIT", error in (no error)=w50) -> (queue out=w46:refnum<queue>, error out=w49:errorcluster)  [unwired: 1 in, 1 out]
  n6 = register-events "Register For Events"(w59, w60) -> (reference out=w58:refnum<event-registration>)  [unwired: 2 in, 1 out]
  n7 = call <vilib>:"DIO Open.vi"("DIO Channel"=DIO_Channel."C/DIO2") -> ("error out"=w18:errorcluster, "DIO Info Out"=w19:T21)  [unwired: 9 in]
  n8 = call <vilib>:"DIO Open.vi"("DIO Channel"=DIO_Channel."C/DIO3") -> ("error out"=w13:errorcluster, "DIO Info Out"=w14:T21)  [unwired: 9 in]
  n9 = call <vilib>:"DIO Open.vi"("DIO Channel"=DIO_Channel."C/DIO1") -> ("error out"=w23:errorcluster, "DIO Info Out"=w24:T21)  [unwired: 9 in]
  n10 = call <vilib>:"DIO Open.vi"("DIO Channel"=DIO_Channel."Not Connected") -> ("error out"=w28:errorcluster, "DIO Info Out"=w30:T21)  [unwired: 9 in]
  n11 = call <vilib>:"DIO Open.vi"("DIO Channel"=DIO_Channel."C/DIO0") -> ("error out"=w33:errorcluster, "DIO Info Out"=w36:T21)  [unwired: 9 in]
  n12 = while {
    tunnel: w36 -> [w112]
    tunnel: [w111] -> w34
    tunnel: w33 -> [w110]
    tunnel: [w81] -> w32
    tunnel: w30 -> [w107]
    tunnel: [w106] -> w29
    tunnel: w28 -> [w105]
    tunnel: [w80] -> w27
    tunnel: [w104] -> w25
    tunnel: w24 -> [w103]
    tunnel: w23 -> [w102]
    tunnel: [w79] -> w22
    tunnel: w19 -> [w96]
    tunnel: w18 -> [w95]
    tunnel: [w94] -> w17
    tunnel: [w77] -> w16
    tunnel: w14 -> [w93]
    tunnel: w13 -> [w92]
    tunnel: [w91] -> w12
    tunnel: [w76] -> w11
    tunnel: [w88] -> w8
    tunnel: [w87] -> w9
    stop <- w114 stop-if-true
    # "ARDUINO LOOP"
    n13 = call <vilib>:"DIO Write.vi"("error in (no error)"=w95, "Input"="Red LED", "DIO Info In"=w96) -> ("error out"=w77:errorcluster, "DIO Info Out"=w94:T21)  [unwired: 7 in]
    n14 = call <vilib>:"DIO Write.vi"("error in (no error)"=w105, "DIO Info In"=w107) -> ("error out"=w80:errorcluster, "DIO Info Out"=w106:T21)  [unwired: 8 in]
    n15 = call <vilib>:"C DIO Read.vi"("error in (no error)"=w102, "DIO Info In in"=w103) -> ("error out"=w79:errorcluster, "IN"=→"TASK ENABLE":bool, "DIO Info In out"=w104:T21)  [unwired: 7 in]
    n16 = call <vilib>:"C DIO Read.vi"("error in (no error)"=w110, "DIO Info In in"=w112) -> ("error out"=w81:errorcluster, "IN"=w109:bool, "DIO Info In out"=w111:T21)  [unwired: 7 in]
    n17 = call <vilib>:"NavX Open.vi"("I2C Channel"=I2C_Channel."A") -> ("error out"=w98:errorcluster, "NavX Info"=w100:T26)  [unwired: 9 in]
    n18 = Not(x="Red LED") -> (.not. x?=w70:bool)
    n19 = call "Digital Debounce Filter.vi"("Boolean input"=w109) -> ("Rising Edge"=→"Rising Edge":bool)  [unwired: 1 in, 2 out]
    n20 = call "Arduino Interfacing VI.vi"("AE Mode"=Arduino_Interfacing."Read From Arduino") -> ("error out"=w82:errorcluster, "Arduino Data"=w84:T7)  [unwired: 3 in]
    "Arduino Data" <- w84
    n21 = And(x=w70, y="Green LED") -> (x .and. y?=w73:bool)
    n22 = call <vilib>:"DIO Write.vi"("error in (no error)"=w92, "Input"=w73, "DIO Info In"=w93) -> ("error out"=w76:errorcluster, "DIO Info Out"=w91:T21)  [unwired: 7 in]
    n23 = Unbundle By Name(w84) -> ("Rotary Switch"=→"Task selection":u8)
    n24 = call "navX reading VI.vi"("NavX Info In"=w100, "Mode"=navX_type_def."Get i2C reference", "error in (no error)"=w98) -> ("NavX Info Out"=w89:T26, "Error Out"=w78:errorcluster)  [unwired: 2 out]
    n25 = call "navX reading VI.vi"("NavX Info In"=w89, "Mode"=navX_type_def."Read Values", "error in (no error)"=w78) -> ("NavX Info Out"=w88:T26, "NavX Readings"=→"NavX Readings":T6, "Status"=→"Status":T4, "Error Out"=w87:errorcluster)
    n26 = Merge Errors(w82, w81, w80, w79, w78, w77, w76) -> (w74:errorcluster)
    "General Errors" <- w74
    n27 = call "FGV Bool.vi"("Init/Read/Write State"=States_for_Action_Engine."Read") -> ("Output node"=w114:bool)  [unwired: 2 in, 1 out]
    n28 = Unbundle By Name(w74) -> ("status"=w71:bool)
    n29 = Wait (ms)(milliseconds to wait=u32 20) -> ()  [unwired: 1 out]
    n30 = local write "Red LED"(w71) -> ()
  }
  n31 = while {
    tunnel: w59 -> [w132]
    tunnel: w60 -> [w131]
    tunnel: [w130] -> w66
    tunnel: [w129] -> w65
    tunnel: w64 -> [w128]
    tunnel: [w127] -> w62
    tunnel: w63 -> [w126]
    tunnel: [w125] -> w61
    stop <- w123 stop-if-true
    # "Generate USER Event Loop"
    n32 = local read "Rising Edge"() -> (w120:bool)
    n33 = Or(x="OK Button", y=w120) -> (x .or. y?=w119:bool)
    n34 = local read "TASK ENABLE"() -> (w118:bool)
    n35 = And(x=w119, y=w118) -> (x .and. y?=w117:bool)
    n36 = case shown="True" w117 {
      selector: w117 -> [_ w143]
      tunnel: w132 -> [w142 w147]
      tunnel: [w142 w146] -> w129
      tunnel: w128 -> [w141 w145]
      tunnel: [w141 w144] -> w127
      frame False {
      }
      frame True {
        n37 = Generate User Event(user event=w147, event data cluster=w143, error in=w145) -> (user event out=w146:refnum<user-event>, error out=w144:errorcluster)  [unwired: 1 in]
      }
    }
    n38 = case shown="False" "STOP" {
      selector: "STOP" -> [_ w136]
      tunnel: w131 -> [w135 w140]
      tunnel: [w135 w139] -> w130
      tunnel: w126 -> [w134 w138]
      tunnel: [w134 w137] -> w125
      tunnel: [FALSE w136] -> w123
      frame False {
      }
      frame True {
        n39 = Generate User Event(user event=w140, event data cluster=w136, error in=w138) -> (user event out=w139:refnum<user-event>, error out=w137:errorcluster)  [unwired: 1 in]
      }
    }
    n40 = Wait (ms)(milliseconds to wait=u32 10) -> ()  [unwired: 1 out]
    n41 = call "FGV Bool.vi"("Init/Read/Write State"=States_for_Action_Engine."Write", "Input Node"=w123) -> ()  [unwired: 1 in, 2 out]
  }
  n42 = while {
    tunnel: w58 -> [w154]
    tunnel: [w153] -> w57
    tunnel: w45 -> [w151]
    tunnel: [w150] -> w56
    tunnel: w51 -> [w149]
    tunnel: [w148] -> w48
    stop <- w152 stop-if-true
    # "EVENT Handling Loop"
    n43 = event shown="[1] <Start Task>: User Event" {
      selector: w154 -> [_ _ _]
      dyn-events: [_ _ _] -> w153
      timeout: _ -> [_ _ _]
      tunnel: [FALSE FALSE w185] -> w152
      tunnel: w151 -> [w159 w168 w183]
      tunnel: [w158 w167 w184] -> w150
      tunnel: w149 -> [w157 w166 w182]
      tunnel: [w156 w165 w181] -> w148
      event Timeout {
        n44 = event-data() -> ()  [unwired: 1 in, 3 out]
        n45 = Enqueue Element(queue=w159, element=Intruction_Type_Definitions."None" ("Enum"), error in (no error)=w157) -> (queue out=w158:refnum<queue>, error out=w156:errorcluster)  [unwired: 1 in, 1 out]
      }
      event User Event {
        n46 = event-data() -> ()  [unwired: 1 in, 5 out]
        n47 = call "Arduino Interfacing VI.vi"("AE Mode"=Arduino_Interfacing."Read From Arduino") -> ("Arduino Data"=w162:T7)  [unwired: 3 in, 1 out]
        n48 = Unbundle By Name(w162) -> ("Rotary Switch"=w161:u8)
        n49 = case shown="8" w161 {
          tunnel: [Intruction_Type_Definitions."None" ("Enum") Intruction_Type_Definitions."Start Task 1" ("Enum") Intruction_Type_Definitions."Start Task 2" ("Enum") Intruction_Type_Definitions."Start Task 3" ("Enum") Intruction_Type_Definitions."Start Task 4" ("Enum") Intruction_Type_Definitions."Start Task 5" ("Enum") Intruction_Type_Definitions."Start Task 6" ("Enum") Intruction_Type_Definitions."Start Task 8 - Gel" ("Enum") Intruction_Type_Definitions."Start Task 9" ("Enum") Intruction_Type_Definitions."Start Task A" ("Enum")] -> w164
          frame 0, Default {
          }
          frame 1 {
          }
          frame 2 {
          }
          frame 3 {
          }
          frame 4 {
          }
          frame 5 {
          }
          frame 6 {
          }
          frame 8 {
          }
          frame 9 {
          }
          frame 10 {
          }
        }
        n50 = Enqueue Element(queue=w168, element=w164, error in (no error)=w166) -> (queue out=w167:refnum<queue>, error out=w165:errorcluster)  [unwired: 1 in, 1 out]
      }
      event User Event {
        n51 = event-data() -> ("Stop Queue"=w185:bool)  [unwired: 1 in, 4 out]
        n52 = Enqueue Element At Opposite End(queue=w183, element=Intruction_Type_Definitions."Exit" ("Enum"), error in (no error)=w182) -> (queue out=w184:refnum<queue>, error out=w181:errorcluster)  [unwired: 1 in, 1 out]
      }
    }
  }
  n53 = while {
    tunnel: w46 -> [w195]
    tunnel: w45 -> [w192]
    stop <- w189 stop-if-true
    # "Status Loop for Action Queues"
    n54 = Get Queue Status(queue=w195, return elements? (F)=TRUE) -> (error out=w191:errorcluster, # elements in queue=→"Action Queue Items":i32, elements=→"Action Queues items":string[])  [unwired: 1 in, 5 out]
    n55 = Get Queue Status(queue=w192, return elements? (F)=TRUE) -> (# pending remove=→"State Logic Queue Items":i32, error out=w190:errorcluster, elements=→"elements":T10[])  [unwired: 1 in, 5 out]
    n56 = Merge Errors(w191, w190) -> (w189:errorcluster)
    n57 = Wait (ms)(milliseconds to wait=u32 500) -> ()  [unwired: 1 out]
  }
  n58 = while {
    tunnel: w45 -> [w236]
    tunnel: w46 -> [w248]
    tunnel: w49 -> [w246]
    tunnel: [w245] -> _
    tunnel: [w244] -> w39
    shift-right: [w237] -> _
    shift-left: T19 {"PING_A"=0, "PING_B"=0, "PING_C"=0, "PING_D"=0} -> [w239]
    shift-right: [w230] -> _
    shift-left: State_Type_Definitions,_for_0.26g_versions_and_later_2."Startup" ("Enum") -> [w233]
    shift-right: [w226] -> _
    shift-left: T20 {"xDistance"=0.0, "yDistance"=0.0, "wDistance"=0.0} -> [w228]
    shift-right: [w223] -> _
    shift-left: _ -> [w222]
    shift-right: [w219] -> _
    shift-left: T1 {"Recognized Object"=FALSE, "Object X coordinate"=0.0, "Object Y coordinate"=0.0} -> [w221]
    shift-right: [w216] -> _
    shift-left: T17 {"y Stepper Position"=0, "z Stepper Position"=0} -> [w218]
    shift-right: [w213] -> _
    shift-left: T16 {"Yaw"=0.0, "Compass"=0.0} -> [w215]
    shift-right: [w210] -> _
    shift-left: T15 {"Time up flag"=FALSE, "SET TIME TO CHECK"=0.0} -> [w212]
    shift-right: [w208] -> _
    shift-left: T14 {"yStepper desired"=0} -> [w209]
    shift-right: [w204] -> _
    shift-left: T13 {"Left IR Sensor"=0.0, "Arm IR Sensor"=0.0, "Bottom IR Sensor"=0.0} -> [w206]
    shift-right: [w202] -> _
    shift-left: T12 {"ySpeed"=0.0, "xSpeed"=0.0, "wSpeed"=0.0} -> [w203]
    shift-right: [w199] -> _
    shift-left: T11 {"Line Detected?"=FALSE, "S1"=0.0, "S2"=0.0, "S3"=0.0, "S4"=0.0} -> [w201]
    stop <- w235 stop-if-true
    # ">>> Motor control cluster >>>"
    # ">>> yStepper command>>>"
    # ">>True Stop Next State >>"
    # ">>Error  >>"
    # ">>Timeout>>"
    # ">>Action states Queue Reference >>"
    # ">>State Logic Queue Reference >>"
    # "TOP LEVEL BASELINE (MAIN PROCESSING LOOP)"
    n59 = Dequeue Element(queue=w248, timeout in ms (-1)=0, error in (no error)=w246) -> (queue out=w240:refnum<queue>, element=w247:string, error out=w241:errorcluster)  [unwired: 1 out]
    "Action State" <- w247
    n60 = Wait (ms)(milliseconds to wait=u32 20) -> ()  [unwired: 1 out]
    n61 = case shown="\"DISPOSE PROC BUFFERS\"" w247 {
      tunnel: [_ _ _ _ _ _ _ _ _ _ _ _ _ _ _ _ _ _ _ _ 0 w2400 _ _ _ _ _ _ _ _ _ _ _ _ _ _ _ _ _ _ _ _ _ _ _ _ _ _ _ _ _] -> w243
      tunnel: w240 -> [_ _ _ _ _ _ _ _ _ _ _ _ _ _ _ _ _ _ _ _ _ _ _ _ _ _ _ _ _ _ _ _ _ _ _ _ _ _ _ _ _ _ _ _ _ _ _ _ _ _ _]
      tunnel: w239 -> [w2117 w2127 w2140 w2152 w2170 w2182 w2194 w2207 w2221 w2234 w2246 w2254 w2270 w2285 w2298 w2309 w2331 w2339 w2367 w2378 w2390 w2401 w2411 w2422 w2453 w2465 w2474 w2484 w2495 w2508 w2522 w2532 w2542 w2561 w2570 w2584 w2592 w2603 w2614 w2625 w2633 w2649 w2657 w2674 w2681 w2694 w2707 w2720 w2733 w2746 w2758]
      tunnel: [w2117 w2127 w2140 w2152 w2170 w2182 w2194 w2207 w2221 w2234 w2246 w2254 w2270 w2286 w2298 w2309 w2331 w2339 w2368 w2378 w2390 w2401 w2411 w2422 w2452 w2465 w2474 w2484 w2495 w2508 w2522 w2532 w2542 w2561 w2570 w2584 w2592 w2603 w2614 w2625 w2633 w2649 w2657 w2674 w2681 w2694 w2707 w2720 w2733 w2746 w2758] -> w238
      tunnel: [TRUE TRUE _ _ _ _ _ _ _ _ _ _ _ _ _ _ _ _ _ _ _ _ _ _ _ _ _ _ _ _ _ _ _ _ _ _ _ _ _ _ _ _ _ _ _ _ _ _ _ _ _] -> w235
      tunnel: w233 -> [w2115 w2125 w2139 w2151 w2169 w2181 w2193 w2206 w2220 w2233 w2245 w2253 w2269 w2284 w2297 w2307 w2324 w2338 w2366 w2377 w2387 w2398 w2410 w2421 w2451 w2464 w2473 w2483 w2487 w2507 w2521 w2531 w2541 w2560 w2569 w2578 w2591 w2602 w2613 w2624 w2632 w2640 w2656 w2673 w2680 w2693 w2706 w2719 w2732 w2745 w2757]
      tunnel: [_ _ _ _ _ _ _ _ _ _ _ _ _ _ _ _ _ _ _ _ _ TRUE _ _ _ _ _ _ _ _ _ _ _ _ _ _ _ _ _ _ _ _ _ _ _ _ _ _ _ _ _] -> w232
      tunnel: [w2115 w2125 w2139 w2151 w2169 w2181 w2193 w2206 w2220 w2233 w2245 w2253 w2269 w2284 w2297 w2307 w2324 w2338 w2366 w2377 w2387 w2398 w2410 w2421 w2451 w2464 w2473 w2483 w2487 w2507 w2521 w2531 w2541 w2560 w2569 w2578 w2591 w2602 w2613 w2624 w2632 w2640 w2656 w2673 w2680 w2693 w2706 w2719 w2732 w2745 w2757] -> w231
      tunnel: w228 -> [w2114 w2124 w2138 w2154 w2168 w2180 w2192 w2205 w2219 w2232 w2244 w2255 w2268 w2283 w2299 w2311 w2326 w2340 w2365 w2379 w2386 w2397 w2412 w2423 w2441 w2463 w2476 w2485 w2492 w2509 w2523 w2533 w2543 w2562 w2572 w2582 w2594 w2605 w2616 w2627 w2635 w2644 w2659 w2676 w2683 w2696 w2709 w2722 w2735 w2748 w2760]
      tunnel: [w2114 w2124 w2138 w2154 w2168 w2180 w2192 w2205 w2219 w2232 w2244 w2255 w2267 w2283 w2299 w2311 w2326 w2340 w2364 w2379 w2386 w2397 w2412 w2423 w2440 w2463 w2476 w2485 w2492 w2509 w2523 w2533 w2543 w2562 w2572 w2582 w2594 w2605 w2616 w2627 w2635 w2644 w2659 w2676 w2683 w2696 w2709 w2722 w2735 w2748 w2760] -> w227
      tunnel: w221 -> [w2113 w2123 w2137 w2153 w2167 w2179 w2191 w2204 w2218 w2231 w2242 w2252 w2266 w2282 w2292 w2310 w2325 w2337 w2356 w2376 w2385 w2396 w2409 w2420 w2446 w2461 w2475 w2482 w2493 w2506 w2520 w2527 w2540 w2555 w2571 w2583 w2593 w2604 w2615 w2626 w2634 w2643 w2658 w2675 w2682 w2695 w2708 w2721 w2734 w2747 w2759]
      tunnel: [w2113 w2123 w2137 w2153 w2167 w2179 w2191 w2204 w2218 w2231 w2242 w2252 w2266 w2282 w2292 w2310 w2325 w2337 w2355 w2376 w2385 w2396 w2409 w2420 w2445 w2461 w2475 w2482 w2493 w2506 w2520 w2527 w2540 w2554 w2571 w2583 w2593 w2604 w2615 w2626 w2634 w2643 w2658 w2675 w2682 w2695 w2708 w2721 w2734 w2747 w2759] -> w220
      tunnel: w218 -> [w2112 w2122 w2136 w2155 w2166 w2178 w2190 w2203 w2217 w2230 w2241 w2251 w2265 w2281 w2300 w2312 w2327 w2336 w2361 w2375 w2384 w2395 w2408 w2419 w2436 w2460 w2472 w2481 w2491 w2505 w2519 w2530 w2539 w2563 w2573 w2581 w2590 w2601 w2612 w2623 w2636 w2645 w2660 w2672 w2684 w2697 w2710 w2723 w2736 w2749 w2761]
      tunnel: [w2112 w2122 w2136 w2155 w2166 w2178 w2190 w2203 w2217 w2230 w2241 w2251 w2265 w2281 w2300 w2312 w2327 w2336 w2360 w2375 w2384 w2395 w2408 w2419 w2435 w2460 w2472 w2481 w2491 w2505 w2519 w2530 w2539 w2563 w2573 w2581 w2590 w2601 w2612 w2623 w2636 w2645 w2660 w2671 w2684 w2697 w2710 w2723 w2736 w2749 w2761] -> w217
      tunnel: w215 -> [w2111 w2121 w2134 w2156 w2164 w2176 w2189 w2201 w2215 w2228 w2240 w2250 w2264 w2274 w2295 w2313 w2328 w2335 w2351 w2374 w2383 w2394 w2407 w2418 w2432 w2459 w2469 w2480 w2490 w2504 w2518 w2529 w2538 w2564 w2574 w2580 w2589 w2598 w2609 w2620 w2637 w2646 w2661 w2666 w2685 w2698 w2711 w2724 w2737 w2750 w2762]
      tunnel: [w2111 w2121 w2134 w2156 w2164 w2176 w2189 w2201 w2215 w2228 w2240 w2250 w2264 w2274 w2294 w2313 w2328 w2335 w2350 w2374 w2383 w2394 w2407 w2418 w2431 w2459 w2469 w2480 w2490 w2504 w2518 w2529 w2538 w2564 w2574 w2580 w2589 w2598 w2609 w2620 w2637 w2646 w2661 w2666 w2685 w2698 w2711 w2724 w2737 w2750 w2762] -> w214
      tunnel: w212 -> [w2109 w2120 w2135 w2157 w2165 w2177 w2188 w2202 w2216 w2229 w2239 w2249 w2263 w2273 w2291 w2314 w2329 w2334 w2347 w2371 w2382 w2393 w2406 w2417 w2429 w2457 w2468 w2479 w2489 w2503 w2517 w2528 w2537 w2565 w2575 w2579 w2588 w2597 w2608 w2619 w2638 w2647 w2662 w2665 w2679 w2692 w2705 w2718 w2731 w2744 w2756]
      tunnel: [w2109 w2120 w2135 w2157 w2165 w2177 w2188 w2202 w2216 w2229 w2239 w2249 w2263 w2273 w2291 w2314 w2329 w2334 w2347 w2371 w2382 w2393 w2406 w2417 w2428 w2457 w2468 w2479 w2489 w2503 w2517 w2528 w2537 w2565 w2575 w2579 w2588 w2597 w2608 w2619 w2638 w2647 w2662 w2665 w2679 w2690 w2703 w2716 w2729 w2742 w2755] -> w211
      tunnel: w209 -> [_ _ _ _ _ _ _ _ _ _ _ _ _ _ _ _ _ _ _ _ _ _ _ _ _ _ _ _ _ _ _ _ _ _ _ _ _ _ _ _ _ _ w2653 _ _ _ _ _ _ _ _]
      tunnel: [w2108 w2119 w2129 w2147 w2159 w2172 w2184 w2196 w2211 w2223 w2236 w2248 w2257 w2272 w2288 w2305 w2330 w2333 w2344 w2370 w2381 w2392 w2405 w2414 w2425 w2456 w2467 w2478 w2494 w2497 w2511 w2525 w2535 w2548 w2567 w2585 w2587 w2596 w2607 w2618 w2629 w2648 w2651 w2664 w2678 w2687 w2700 w2713 w2726 w2739 w2752] -> w205
      tunnel: w206 -> [w2108 w2119 w2129 w2147 w2159 w2172 w2184 w2196 w2211 w2223 w2236 w2248 w2257 w2272 w2288 w2306 w2330 w2333 w2344 w2370 w2381 w2392 w2405 w2414 w2425 w2456 w2467 w2478 w2494 w2497 w2511 w2525 w2535 w2548 w2567 w2585 w2587 w2596 w2607 w2618 w2629 w2648 w2651 w2664 w2678 w2687 w2700 w2713 w2726 w2739 w2752]
      tunnel: w203 -> [_ _ _ _ _ _ _ _ w2210 _ _ _ _ _ _ _ _ _ _ _ _ _ _ _ _ _ _ _ _ _ _ _ _ _ _ _ _ _ _ _ _ _ _ _ _ _ _ _ _ _ _]
      tunnel: w201 -> [w2107 w2118 w2128 w2141 w2158 w2171 w2183 w2195 w2208 w2222 w2235 w2247 w2256 w2271 w2287 w2301 w2323 w2332 w2342 w2369 w2380 w2391 w2404 w2413 w2424 w2455 w2466 w2477 w2486 w2496 w2510 w2524 w2534 w2545 w2566 w2576 w2586 w2595 w2606 w2617 w2628 w2639 w2650 w2663 w2677 w2686 w2699 w2712 w2725 w2738 w2751]
      tunnel: [w2107 w2118 w2128 w2141 w2158 w2171 w2183 w2195 w2208 w2222 w2235 w2247 w2256 w2271 w2287 w2301 w2322 w2332 w2342 w2369 w2380 w2391 w2404 w2413 w2424 w2455 w2466 w2477 w2486 w2496 w2510 w2524 w2534 w2545 w2566 w2576 w2586 w2595 w2606 w2617 w2628 w2639 w2650 w2663 w2677 w2686 w2699 w2712 w2725 w2738 w2751] -> w200
      tunnel: [_ _ _ _ _ _ _ _ _ _ _ _ _ _ _ _ _ _ _ _ _ _ _ _ _ _ _ _ _ _ _ _ _ w2544 _ _ _ _ _ _ _ _ _ _ _ _ _ _ _ _ _] -> w198
      frame "Exit" {
        # ">>State Logic  >>"
        # ">>> Time cluster >>>"
        # ">>> Yaw >>>"
        # ">>> Stepper position >>>"
        # ">>> Encoders >>>"
        # ">>> Object detection >>>"
        # ">>> Ultrasonic Sensors Detect >>>"
        n62 = call "Imaq Dispose"("All Images? (No)"=TRUE) -> ()  [unwired: 5 in, 1 out]
      }
      frame "----Movement States----" {
        # ">>State Logic  >>"
        # ">>> Time cluster >>>"
        # ">>> Yaw >>>"
        # ">>> Stepper position >>>"
        # ">>> Encoders >>>"
        # ">>> Object detection >>>"
        # ">>> Ultrasonic Sensors Detect >>>"
      }
      frame "FORWARD" {
        # ">>State Logic  >>"
        # ">>> Time cluster >>>"
        # ">>> Yaw >>>"
        # ">>> Stepper position >>>"
        # ">>> Encoders >>>"
        # ">>> Object detection >>>"
        # ">>> Ultrasonic Sensors Detect >>>"
        n63 = Unbundle By Name(w2134) -> ("Yaw"=w2130:dbl)
        n64 = call "MOTOR CONTROL WITH PID AE.vi"("Yaw"=w2130, "Speed"=50.0, "Direction"=MOTOR_CONTROL_WITH_PID_AE_DIRECTION_TYPE_DEF."y-axis movement", "AE Mode"=MOTOR_CONTROL_WITH_PID_AE_DATA_MODE_TYPE_DEF."Write to AE") -> ()  [unwired: 1 out]
      }
      frame "FORWARD - IR ASSIST" {
        # ">>State Logic  >>"
        # ">>> Time cluster >>>"
        # ">>> Yaw >>>"
        # ">>> Stepper position >>>"
        # ">>> Encoders >>>"
        # ">>> Object detection >>>"
        # ">>> Ultrasonic Sensors Detect >>>"
        n65 = Unbundle By Name(w2147) -> ("Left IR Sensor"=w2146:dbl)
        n66 = Subtract(x=w2146, y=20.0) -> (x-y=w2144:dbl)
        n67 = Multiply(x=w2144, y=0.25) -> (x*y=w2142:dbl)
        n68 = call "MOTOR CONTROL WITH PID AE.vi"("Yaw"=w2142, "Speed"=30.0, "Direction"=MOTOR_CONTROL_WITH_PID_AE_DIRECTION_TYPE_DEF."y-axis movement", "AE Mode"=MOTOR_CONTROL_WITH_PID_AE_DATA_MODE_TYPE_DEF."Write to AE") -> ()  [unwired: 1 out]
      }
      frame "LEFT" {
        # ">>State Logic  >>"
        # ">>> Time cluster >>>"
        # ">>> Yaw >>>"
        # ">>> Stepper position >>>"
        # ">>> Encoders >>>"
        # ">>> Object detection >>>"
        # ">>> Ultrasonic Sensors Detect >>>"
        n69 = Unbundle By Name(w2164) -> ("Yaw"=w2161:dbl)
        n70 = call "MOTOR CONTROL WITH PID AE.vi"("Yaw"=w2161, "Speed"=-25.0, "Direction"=MOTOR_CONTROL_WITH_PID_AE_DIRECTION_TYPE_DEF."x-axis movement", "AE Mode"=MOTOR_CONTROL_WITH_PID_AE_DATA_MODE_TYPE_DEF."Write to AE") -> ()  [unwired: 1 out]
      }
      frame "R-ACW" {
        # ">>> IR Sensors >>>"
        # ">>> Time cluster >>>"
        # ">>> Yaw >>>"
        # ">>> Stepper position >>>"
        # ">>> Encoders >>>"
        # ">>> Object detection >>>"
        # ">>> Ultrasonic Sensors Detect >>>"
        n71 = call "MOTOR CONTROL WITH PID AE.vi"("Speed"=-10.0, "Direction"=MOTOR_CONTROL_WITH_PID_AE_DIRECTION_TYPE_DEF."rotation", "AE Mode"=MOTOR_CONTROL_WITH_PID_AE_DATA_MODE_TYPE_DEF."Write to AE") -> ()  [unwired: 1 in, 1 out]
      }
      frame "R-CW" {
        (unwired) -0.2 ("Speed")
        # ">>> Time cluster >>>"
        # ">>> Yaw >>>"
        # ">>> Stepper position >>>"
        # ">>> Encoders >>>"
        # ">>> Object detection >>>"
        # ">>> Ultrasonic Sensors Detect >>>"
        n72 = call "MOTOR CONTROL WITH PID AE.vi"("Speed"=10.0, "Direction"=MOTOR_CONTROL_WITH_PID_AE_DIRECTION_TYPE_DEF."rotation", "AE Mode"=MOTOR_CONTROL_WITH_PID_AE_DATA_MODE_TYPE_DEF."Write to AE") -> ()  [unwired: 1 in, 1 out]
      }
      frame "RIGHT" {
        # ">>> Time cluster >>>"
        # ">>> Yaw >>>"
        # ">>> Stepper position >>>"
        # ">>> Encoders >>>"
        # ">>> Object detection >>>"
        # ">>> Ultrasonic Sensors Detect >>>"
        n73 = Unbundle By Name(w2201) -> ("Yaw"=w2197:dbl)
        n74 = call "MOTOR CONTROL WITH PID AE.vi"("Yaw"=w2197, "Speed"=50.0, "Direction"=MOTOR_CONTROL_WITH_PID_AE_DIRECTION_TYPE_DEF."x-axis movement", "AE Mode"=MOTOR_CONTROL_WITH_PID_AE_DATA_MODE_TYPE_DEF."Write to AE") -> ()  [unwired: 1 out]
      }
      frame "X AXIS - SLOW" {
        # ">>> IR Sensors >>>"
        # ">>> Time cluster >>>"
        # ">>> Yaw >>>"
        # ">>> Stepper position >>>"
        # ">>> Encoders >>>"
        # ">>> Object detection >>>"
        # ">>> Ultrasonic Sensors Detect >>>"
        n75 = Unbundle By Name(w2210) -> ("xSpeed"=w2209:dbl)
        n76 = Unbundle By Name(w2215) -> ("Yaw"=w2212:dbl)
        n77 = call "MOTOR CONTROL WITH PID AE.vi"("Yaw"=w2212, "Speed"=w2209, "Direction"=MOTOR_CONTROL_WITH_PID_AE_DIRECTION_TYPE_DEF."x-axis movement", "AE Mode"=MOTOR_CONTROL_WITH_PID_AE_DATA_MODE_TYPE_DEF."Write to AE") -> ()  [unwired: 1 out]
      }
      frame "REVERSE" {
        # ">>> Time cluster >>>"
        # ">>> Yaw >>>"
        # ">>> Stepper position >>>"
        # ">>> Encoders >>>"
        # ">>> Object detection >>>"
        # ">>> Ultrasonic Sensors Detect >>>"
        n78 = Unbundle By Name(w2228) -> ("Yaw"=w2224:dbl)
        n79 = call "MOTOR CONTROL WITH PID AE.vi"("Yaw"=w2224, "Speed"=-50.0, "Direction"=MOTOR_CONTROL_WITH_PID_AE_DIRECTION_TYPE_DEF."y-axis movement", "AE Mode"=MOTOR_CONTROL_WITH_PID_AE_DATA_MODE_TYPE_DEF."Write to AE") -> ()  [unwired: 1 out]
      }
      frame "STOP" {
        n80 = Wait (ms)(milliseconds to wait=u32 100) -> ()  [unwired: 1 out]
        n81 = call "MOTOR CONTROL WITH PID AE.vi"("Direction"=MOTOR_CONTROL_WITH_PID_AE_DIRECTION_TYPE_DEF."stop", "AE Mode"=MOTOR_CONTROL_WITH_PID_AE_DATA_MODE_TYPE_DEF."Write to AE") -> ()  [unwired: 2 in, 1 out]
      }
      frame "----SENSOR READING---- " {
      }
      frame "READ ENCODERS" {
        # ">>> Time cluster >>>"
        # ">>> Yaw >>>"
        # ">>> Stepper position >>>"
        # ">>> Object detection >>>"
        # ">>> Current encoder distance >>>"
        # ">>> Ultrasonic Sensors Detect >>>"
        n82 = call "MOTOR CONTROL WITH PID AE.vi"("AE Mode"=MOTOR_CONTROL_WITH_PID_AE_DATA_MODE_TYPE_DEF."Read from AE") -> ("Speed & distance"=w2261:T5)  [unwired: 3 in]
        n83 = Unbundle By Name(w2261) -> ("xDistance"=w2260:dbl, "yDistance"=w2259:dbl, "wDistance"=w2258:dbl)
        n84 = Bundle By Name(cluster=w2268, "xDistance"=w2260, "yDistance"=w2259, "wDistance"=w2258) -> (w2267:T20)
      }
      frame "READ ULTRASONIC" {
        (unwired) navX_type_def."Read Values" ("Mode")
        (unwired) MOTOR_CONTROL_NO_PID_Type_Def."Latch" ("Direction")
        # ">>State Logic  >>"
        # ">>> Time cluster >>>"
        # ">>> Ultrasonic Sensors Detect >>>"
        # ">>> Object detection >>>"
        # ">>> Encoders >>>"
        # ">>> Stepper position >>>"
        # ">>> Yaw >>>"
        n85 = call "Arduino Interfacing VI.vi"("AE Mode"=Arduino_Interfacing."Read From Arduino") -> ("Arduino Data"=w2279:T7)  [unwired: 3 in, 1 out]
        n86 = Unbundle By Name(w2279) -> ("PING A"=w2278:u8, "PING B"=w2277:u8, "PING C"=w2276:u8, "PING D"=w2275:u8)
        n87 = Bundle By Name(cluster=w2285, "PING_A"=w2278, "PING_B"=w2277, "PING_C"=w2276, "PING_D"=w2275) -> (w2286:T19)
      }
      frame "READ NAVX" {
        # ">>> Time cluster >>>"
        # ">>> Yaw >>>"
        # ">>> Ultrasonic Sensors Detect >>>"
        # ">>> Object detection >>>"
        # ">>> Encoders >>>"
        # ">>> Stepper position >>>"
        n88 = call "navX reading VI.vi"("Mode"=navX_type_def."Read Values") -> ("NavX Readings"=w2290:T6)  [unwired: 2 in, 3 out]
        n89 = Unbundle By Name(w2290) -> ("Heading"=w2289:dbl)
        n90 = Unbundle By Name(w2290) -> ("Yaw"=w2293:dbl)
        n91 = Bundle By Name(cluster=w2295, "Yaw"=w2293, "Compass"=w2289) -> (w2294:T16)
      }
      frame "READ IR" {
        w2303 = T37 [enum."B/AI1"] items=["Not Connected", "AudioIn/Left", "AudioIn/Right", "C/AI0", "C/AI1", "A/AI0", "A/AI1", "A/AI2", "A/AI3", "A/AI4", "A/AI5", "A/AI6", "A/AI7", "B/AI0", "B/AI1", "B/AI2", "B/AI3", "B/AI4", "B/AI5", "B/AI6", "B/AI7", "AI/AI0", "AI/AI1", "AI/AI2", "AI/AI3", "A/AI0 (DIFF)", "A/AI1 (DIFF)", "A/AI2 (DIFF)", "A/AI3 (DIFF)", "B/AI0 (DIFF)", "B/AI1 (DIFF)", "B/AI2 (DIFF)", "B/AI3 (DIFF)"] ("AI Channel")
        w2308 = T37 [enum."B/AI0"] items=["Not Connected", "AudioIn/Left", "AudioIn/Right", "C/AI0", "C/AI1", "A/AI0", "A/AI1", "A/AI2", "A/AI3", "A/AI4", "A/AI5", "A/AI6", "A/AI7", "B/AI0", "B/AI1", "B/AI2", "B/AI3", "B/AI4", "B/AI5", "B/AI6", "B/AI7", "AI/AI0", "AI/AI1", "AI/AI2", "AI/AI3", "A/AI0 (DIFF)", "A/AI1 (DIFF)", "A/AI2 (DIFF)", "A/AI3 (DIFF)", "B/AI0 (DIFF)", "B/AI1 (DIFF)", "B/AI2 (DIFF)", "B/AI3 (DIFF)"] ("AI Channel")
        # ">>State Logic  >>"
        # ">>> Time cluster >>>"
        # ">>> Ultrasonic Sensors Detect >>>"
        # ">>> Object detection >>>"
        # ">>> Encoders >>>"
        # ">>> Stepper position >>>"
        # ">>> Yaw >>>"
        n92 = call <vilib>:"Sharp IR.vi"("AI Channel"=w2308) -> ("Sharp IR Distance"=w2304:dbl)  [unwired: 8 in, 2 out]
        n93 = call <vilib>:"Sharp IR.vi"("AI Channel"=w2303) -> ("Sharp IR Distance"=w2302:dbl)  [unwired: 8 in, 2 out]
        n94 = Bundle By Name(cluster=w2306, "Left IR Sensor"=w2304, "Arm IR Sensor"=w2302) -> (w2305:T13)
      }
      frame "READ LINE SENSOR" {
        # ">>> IR Sensors >>>"
        # ">>> Line Sensor Cluster>>>"
        # ">>State Logic  >>"
        # ">>> Time cluster >>>"
        # ">>> Object detection >>>"
        # ">>> Yaw >>>"
        # ">>> Ultrasonic Sensors Detect >>>"
        # ">>> Encoders >>>"
        # ">>> Stepper position >>>"
        n95 = call "Line Sensor AE.vi"("AE State"=Line_Sensor_AE_Type_Def."READ FROM LINE SENSORS") -> ("Line Detected?"=w2320:bool, "Line Sensor Raw Values"=w2319:T39)
        n96 = Unbundle By Name(w2319) -> ("S1"=w2318:dbl, "S2"=w2317:dbl, "S3"=w2316:dbl, "S4"=w2315:dbl)
        n97 = Bundle By Name(cluster=w2323, "Line Detected?"=w2320, "S1"=w2318, "S2"=w2317, "S3"=w2316, "S4"=w2315) -> (w2322:T11)
      }
      frame "----SYSTEM MODES----" {
        (unwired) I2C_MASTER_Type_Def."Last State" ("Arduino Mode")
        # ">>> Object detection >>>"
        # ">>> Yaw >>>"
        # ">>> Ultrasonic Sensors Detect >>>"
        # ">>> Encoders >>>"
        # ">>> Stepper position >>>"
      }
      frame "INIT" {
        w2362 = u8 0
        w2363 = 0.0
        # ">>> IR Sensors >>>"
        # ">>> IR Sensors >>>"
        # ">>> Line Sensor Cluster>>>"
        # ">>> Time cluster >>>"
        # ">>> Object detection >>>"
        # ">>> Yaw >>>"
        # ">>> Ultrasonic Sensors Detect >>>"
        # ">>> Encoders >>>"
        # ">>> Stepper position >>>"
        # ">>State Logic  >>"
        n98 = call "Arduino Interfacing VI.vi"("AE Mode"=Arduino_Interfacing."Initialize") -> ()  [unwired: 3 in, 2 out]
        n99 = call "FGV Bool.vi"("Init/Read/Write State"=States_for_Action_Engine."Initialize") -> ()  [unwired: 2 in, 2 out]
        n100 = call "Elasped Timer.vi"("Action"=Elapsed_timer_control."Initialize") -> ()  [unwired: 7 in, 4 out]
        n101 = call "MOTOR CONTROL WITH PID AE.vi"("AE Mode"=MOTOR_CONTROL_WITH_PID_AE_DATA_MODE_TYPE_DEF."Init AE") -> ()  [unwired: 3 in, 1 out]
        n102 = call "IMAQ Reference AE.vi"("IMAQ AE States"=IMAQ_Reference_AE."Initialize AE") -> ()  [unwired: 1 in, 2 out]
        n103 = call "Line Sensor AE.vi"("AE State"=Line_Sensor_AE_Type_Def."INIT AE") -> ()  [unwired: 2 out]
        n104 = Bundle By Name(cluster=w2356, "Recognized Object"=FALSE, "Object X coordinate"=0.0, "Object Y coordinate"=0.0) -> (w2355:T1)
        n105 = Bundle By Name(cluster=w2361, "y Stepper Position"=u8 0, "z Stepper Position"=u8 0) -> (w2360:T17)
        n106 = Bundle By Name(cluster=w2365, "xDistance"=w2363, "yDistance"=w2363, "wDistance"=w2363) -> (w2364:T20)
        n107 = Bundle By Name(cluster=w2367, "PING_A"=w2362, "PING_B"=w2362, "PING_C"=w2362, "PING_D"=w2362) -> (w2368:T19)
        n108 = Bundle By Name(cluster=w2351, "Yaw"=0.0) -> (w2350:T16)
      }
      frame "ARDUINO - ULTRASONIC" {
        # ">>> Time cluster >>>"
        # ">>> Line Sensor Cluster>>>"
        # ">>> Object detection >>>"
        # ">>> Yaw >>>"
        # ">>> Ultrasonic Sensors Detect >>>"
        # ">>> Encoders >>>"
        # ">>> Stepper position >>>"
        # ">>State Logic  >>"
        n109 = call "Arduino Interfacing VI.vi"("Data to Write"=I2C_MASTER_WRITE_NEW_Type_Def."Ultrasonic sensors", "AE Mode"=Arduino_Interfacing."Write to Arduino") -> ()  [unwired: 2 in, 2 out]
      }
      frame "NAVX CALIBRATE" {
        # ">>> Object detection >>>"
        # ">>> Yaw >>>"
        # ">>> Ultrasonic Sensors Detect >>>"
        # ">>> Encoders >>>"
        # ">>> Stepper position >>>"
        # ">>State Logic  >>"
        # "Adds a 15 second delay to the startup process \nfor the NavX to calibrate"
        n110 = Wait (ms)(milliseconds to wait=u32 1000) -> ()  [unwired: 1 out]
      }
      frame "NO ACTION", Default {
        (unwired) u8 0 ("y Stepper value")
        (unwired) TRUE ("Latch")
        (unwired) navX_type_def."Read Values" ("Mode")
        (unwired) MOTOR_CONTROL_NO_PID_Type_Def."Latch" ("Direction")
        # ">>> Object detection >>>"
        # ">>> Yaw >>>"
        # ">>> Ultrasonic Sensors Detect >>>"
        # ">>> Encoders >>>"
        # ">>> Stepper position >>>"
        # ">>State Logic  >>"
        n111 = case shown="4" w2398 {
          tunnel: [0 100] -> w2400
          frame 1, Default {
          }
          frame 4 {
          }
        }
      }
      frame "----RESET CASES----" {
        (unwired) I2C_MASTER_Type_Def."Last State" ("Arduino Mode")
        # ">>> Object detection >>>"
        # ">>> Yaw >>>"
        # ">>> Ultrasonic Sensors Detect >>>"
        # ">>> Encoders >>>"
        # ">>> Stepper position >>>"
        # ">>State Logic  >>"
      }
      frame "RESET ENCODERS" {
        # ">>> Object detection >>>"
        # ">>> Yaw >>>"
        # ">>> Ultrasonic Sensors Detect >>>"
        # ">>> Encoders >>>"
        # ">>> Stepper position >>>"
        # ">>State Logic  >>"
        n112 = call "MOTOR CONTROL WITH PID AE.vi"("Direction"=MOTOR_CONTROL_WITH_PID_AE_DIRECTION_TYPE_DEF."reset encoders", "AE Mode"=MOTOR_CONTROL_WITH_PID_AE_DATA_MODE_TYPE_DEF."Write to AE") -> ()  [unwired: 2 in, 1 out]
      }
      frame "RESET FLAGS" {
        (unwired) I2C_MASTER_Type_Def."Last State" ("Arduino Mode")
        # "Resets any software variables\nand/or non-critical states"
        n113 = Wait (ms)(milliseconds to wait=u32 20) -> ()  [unwired: 1 out]
        n114 = Bundle By Name(cluster=w2429, "Time up flag"=FALSE, "SET TIME TO CHECK"=0.0) -> (w2428:T15)
        n115 = Bundle By Name(cluster=w2446, "Recognized Object"=FALSE, "Object X coordinate"=0.0, "Object Y coordinate"=0.0) -> (w2445:T1)
        n116 = Bundle By Name(cluster=w2436, "y Stepper Position"=u8 0, "z Stepper Position"=u8 0) -> (w2435:T17)
        n117 = Bundle By Name(cluster=w2441, "xDistance"=0.0, "yDistance"=0.0, "wDistance"=0.0) -> (w2440:T20)
        n118 = Bundle By Name(cluster=w2453, "PING_A"=u8 0, "PING_B"=u8 0, "PING_C"=u8 0, "PING_D"=u8 0) -> (w2452:T19)
        n119 = Bundle By Name(cluster=w2432, "Yaw"=0.0) -> (w2431:T16)
      }
      frame "RESET YAW" {
        n120 = Wait (ms)(milliseconds to wait=u32 100) -> ()  [unwired: 1 out]
        n121 = call "navX reading VI.vi"("Mode"=navX_type_def."Zero Yaw") -> ()  [unwired: 2 in, 4 out]
      }
      frame "RESET ARM" {
        n122 = call "Arduino Interfacing VI.vi"("Data to Write"=I2C_MASTER_WRITE_NEW_Type_Def."Soft Reset", "AE Mode"=Arduino_Interfacing."Write to Arduino") -> ()  [unwired: 2 in, 2 out]
      }
      frame "--------CAM STATES-------" {
      }
      frame "OPEN IMAQ REF" {
        # ">>> Line Sensor Cluster>>>"
        # ">>State Logic  >>"
        # ">>> Time cluster >>>"
        # ">>> Object detection >>>"
        # ">>> Yaw >>>"
        # ">>> Ultrasonic Sensors Detect >>>"
        # ">>> Encoders >>>"
        # ">>> Stepper position >>>"
        # ">>> IR Sensors >>>"
        n123 = call "IMAQ Reference AE.vi"("IMAQ AE States"=IMAQ_Reference_AE."Initialize AE") -> ()  [unwired: 1 in, 2 out]
      }
      frame "OPEN LOG CAM" {
        n124 = call "Webcam AE.vi"("Session In"=T35 "cam0", "Camera states"=Webcam_AE."Initialize Camera") -> ("error out"=w2500:errorcluster, "Session Out"=w2499:T35)  [unwired: 1 in, 1 out]
        n125 = call "Webcam AE.vi"("error in (no error)"=w2500, "Session In"=w2499, "Camera states"=Webcam_AE."Open Camera") -> ()  [unwired: 3 out]
      }
      frame "OPEN LIFE CAM" {
        n126 = call "Webcam AE.vi"("Session In"=T35 "cam1", "Camera states"=Webcam_AE."Initialize Camera") -> ("error out"=w2514:errorcluster, "Session Out"=w2513:T35)  [unwired: 1 in, 1 out]
        n127 = call "Webcam AE.vi"("error in (no error)"=w2514, "Session In"=w2513, "Camera states"=Webcam_AE."Open Camera") -> ()  [unwired: 3 out]
      }
      frame "CAM ACQ" {
        # ">>State Logic  >>"
        # ">>> Time cluster >>>"
        # ">>> Yaw >>>"
        # ">>> Stepper position >>>"
        # ">>> Encoders >>>"
        # ">>> Object detection >>>"
        # ">>> Ultrasonic Sensors Detect >>>"
        n128 = call "Webcam AE.vi"("Camera states"=Webcam_AE."Continuous Acquisition") -> ()  [unwired: 2 in, 3 out]
      }
      frame "CAM CLOSE" {
        # ">>State Logic  >>"
        # ">>> Time cluster >>>"
        # ">>> Yaw >>>"
        # ">>> Stepper position >>>"
        # ">>> Encoders >>>"
        # ">>> Object detection >>>"
        # ">>> Ultrasonic Sensors Detect >>>"
        n129 = call "Webcam AE.vi"("Camera states"=Webcam_AE."Close Camera") -> ()  [unwired: 2 in, 3 out]
      }
      frame "PROCESS IMAGE" {
        # ">>State Logic  >>"
        # ">>> Time cluster >>>"
        # ">>> Yaw >>>"
        # ">>> Stepper position >>>"
        # ">>> Encoders >>>"
        # ">>> Object detection >>>"
        # ">>> Ultrasonic Sensors Detect >>>"
        n130 = call "Webcam AE.vi"("Camera states"=Webcam_AE."Retrieve Image") -> ("error out"=w2556:errorcluster, "Image Out"=w2558:T41)  [unwired: 2 in, 1 out]
        n131 = call "IMAQ Reference AE.vi"("IMAQ AE States"=IMAQ_Reference_AE."Get IMAQ Reference") -> ("Image Out"=w2546:T41)  [unwired: 1 in, 1 out]
        n132 = call "Object Detection SubVI.vi"("Error In"=w2556, "Mode"="Object recognition mode", "Image Dest"=w2546, "Image in"=w2558) -> ("Error out"=w2544:errorcluster, "Object Center Coordinates"=w2553:cluster{"x":sgl, "y":sgl}, "Object detection cluster"=w2549:T42)  [unwired: 1 out]
        n133 = Unbundle By Name(w2549) -> ("Object detected?"=w2550:bool)
        n134 = Unbundle By Name(w2553) -> ("x"=w2552:sgl, "y"=w2551:sgl)
        n135 = Bundle By Name(cluster=w2555, "Recognized Object"=w2550, "Object X coordinate"=w2552, "Object Y coordinate"=w2551) -> (w2554:T1)
      }
      frame "DISPOSE CAM BUFFERS" {
        # ">>> Line Sensor Cluster>>>"
        # ">>> IR Sensors >>>"
        # ">>State Logic  >>"
        # ">>> Time cluster >>>"
        # ">>> Yaw >>>"
        # ">>> Stepper position >>>"
        # ">>> Encoders >>>"
        # ">>> Object detection >>>"
        # ">>> Ultrasonic Sensors Detect >>>"
        n136 = call "Webcam AE.vi"("Camera states"=Webcam_AE."Dispose Camera Image Buffer") -> ()  [unwired: 2 in, 3 out]
      }
      frame "DISPOSE PROC BUFFERS" {
        # ">>> Line Sensor Cluster>>>"
        # ">>State Logic  >>"
        # ">>> IR Sensors >>>"
        # ">>> Time cluster >>>"
        # ">>> Object detection >>>"
        # ">>> Yaw >>>"
        # ">>> Ultrasonic Sensors Detect >>>"
        # ">>> Encoders >>>"
        # ">>> Stepper position >>>"
        n137 = call "IMAQ Reference AE.vi"("IMAQ AE States"=IMAQ_Reference_AE."Dispose Processing Buffer") -> ()  [unwired: 1 in, 2 out]
      }
      frame "-----ARM ACTIONS-----" {
      }
      frame "CLOSE CLAW" {
        n138 = call "Arduino Interfacing VI.vi"("Data to Write"=I2C_MASTER_WRITE_NEW_Type_Def."Close Claw", "AE Mode"=Arduino_Interfacing."Write to Arduino") -> ()  [unwired: 2 in, 2 out]
      }
      frame "OPEN CLAW" {
        n139 = call "Arduino Interfacing VI.vi"("Data to Write"=I2C_MASTER_WRITE_NEW_Type_Def."Open Claw", "AE Mode"=Arduino_Interfacing."Write to Arduino") -> ()  [unwired: 2 in, 2 out]
      }
      frame "Z STEPPER CAM HEIGHT" {
        n140 = call "Arduino Interfacing VI.vi"("Data to Write"=I2C_MASTER_WRITE_NEW_Type_Def."zStepper 6k", "AE Mode"=Arduino_Interfacing."Write to Arduino") -> ()  [unwired: 2 in, 2 out]
      }
      frame "Z STEPPER GRAB HEIGHT" {
        # ">>State Logic  >>"
        # ">>> Time cluster >>>"
        # ">>> Yaw >>>"
        # ">>> Stepper position >>>"
        # ">>> Encoders >>>"
        # ">>> Object detection >>>"
        # ">>> Ultrasonic Sensors Detect >>>"
        n141 = call "Arduino Interfacing VI.vi"("Data to Write"=I2C_MASTER_WRITE_NEW_Type_Def."zStepper 100", "AE Mode"=Arduino_Interfacing."Write to Arduino") -> ()  [unwired: 2 in, 2 out]
      }
      frame "Z STEPPER BOX HEIGHT" {
        # ">>> IR Sensors >>>"
        # ">>> Time cluster >>>"
        # ">>> Yaw >>>"
        # ">>> Stepper position >>>"
        # ">>> Encoders >>>"
        # ">>> Object detection >>>"
        # ">>> Ultrasonic Sensors Detect >>>"
        n142 = call "Arduino Interfacing VI.vi"("Data to Write"=I2C_MASTER_WRITE_NEW_Type_Def."zStepper 4k", "AE Mode"=Arduino_Interfacing."Write to Arduino") -> ()  [unwired: 2 in, 2 out]
      }
      frame "Y STEPPER CONTROL" {
        # ">>State Logic  >>"
        # ">>> yStepper command>>>"
        # ">>> Time cluster >>>"
        # ">>> Yaw >>>"
        # ">>> Stepper position >>>"
        # ">>> Encoders >>>"
        # ">>> Object detection >>>"
        # ">>> Ultrasonic Sensors Detect >>>"
        n143 = Unbundle By Name(w2653) -> ("yStepper desired"=w2652:u8)
        n144 = call "Arduino Interfacing VI.vi"("y Stepper value"=w2652, "Data to Write"=I2C_MASTER_WRITE_NEW_Type_Def."yStepper control", "AE Mode"=Arduino_Interfacing."Write to Arduino") -> ()  [unwired: 1 in, 2 out]
      }
      frame "READ STEPPER VALUES" {
        # ">>State Logic  >>"
        # ">>> Time cluster >>>"
        # ">>> Yaw >>>"
        # ">>> Stepper position >>>"
        # ">>> Encoders >>>"
        # ">>> Object detection >>>"
        # ">>> Ultrasonic Sensors Detect >>>"
        n145 = call "Arduino Interfacing VI.vi"("AE Mode"=Arduino_Interfacing."Read From Arduino") -> ("Arduino Data"=w2669:T7)  [unwired: 3 in, 1 out]
        n146 = Unbundle By Name(w2669) -> ("y Stepper Position"=w2668:u8, "z Stepper Position"=w2667:u8)
        n147 = Bundle By Name(cluster=w2672, "y Stepper Position"=w2668, "z Stepper Position"=w2667) -> (w2671:T17)
      }
      frame " -----TIMING-----" {
        # ">>State Logic  >>"
        # ">>> Time cluster >>>"
        # ">>> Yaw >>>"
        # ">>> Stepper position >>>"
        # ">>> Encoders >>>"
        # ">>> Object detection >>>"
        # ">>> Ultrasonic Sensors Detect >>>"
      }
      frame "SET TIMER 1" {
        # ">>State Logic  >>"
        # ">>> Time cluster >>>"
        # ">>> Yaw >>>"
        # ">>> Stepper position >>>"
        # ">>> Encoders >>>"
        # ">>> Object detection >>>"
        # ">>> Ultrasonic Sensors Detect >>>"
        n148 = call "Elasped Timer.vi"("Time Setting"=1.0, "Action"=Elapsed_timer_control."Initialize") -> ()  [unwired: 6 in, 4 out]
        n149 = Bundle By Name(cluster=w2692, "Time up flag"=FALSE) -> (w2690:T15)
      }
      frame "SET TIMER 2" {
        # ">>State Logic  >>"
        # ">>> Time cluster >>>"
        # ">>> Yaw >>>"
        # ">>> Stepper position >>>"
        # ">>> Encoders >>>"
        # ">>> Object detection >>>"
        # ">>> Ultrasonic Sensors Detect >>>"
        n150 = call "Elasped Timer.vi"("Time Setting"=2.0, "Action"=Elapsed_timer_control."Initialize") -> ()  [unwired: 6 in, 4 out]
        n151 = Bundle By Name(cluster=w2705, "Time up flag"=FALSE) -> (w2703:T15)
      }
      frame "SET TIMER 3" {
        # ">>State Logic  >>"
        # ">>> Time cluster >>>"
        # ">>> Yaw >>>"
        # ">>> Stepper position >>>"
        # ">>> Encoders >>>"
        # ">>> Object detection >>>"
        # ">>> Ultrasonic Sensors Detect >>>"
        n152 = call "Elasped Timer.vi"("Time Setting"=3.0, "Action"=Elapsed_timer_control."Initialize") -> ()  [unwired: 6 in, 4 out]
        n153 = Bundle By Name(cluster=w2718, "Time up flag"=FALSE) -> (w2716:T15)
      }
      frame "SET TIMER 4" {
        # ">>State Logic  >>"
        # ">>> Time cluster >>>"
        # ">>> Yaw >>>"
        # ">>> Stepper position >>>"
        # ">>> Encoders >>>"
        # ">>> Object detection >>>"
        # ">>> Ultrasonic Sensors Detect >>>"
        n154 = call "Elasped Timer.vi"("Time Setting"=4.0, "Action"=Elapsed_timer_control."Initialize") -> ()  [unwired: 6 in, 4 out]
        n155 = Bundle By Name(cluster=w2731, "Time up flag"=FALSE) -> (w2729:T15)
      }
      frame "SET TIMER 5" {
        # ">>State Logic  >>"
        # ">>> Time cluster >>>"
        # ">>> Yaw >>>"
        # ">>> Stepper position >>>"
        # ">>> Encoders >>>"
        # ">>> Object detection >>>"
        # ">>> Ultrasonic Sensors Detect >>>"
        n156 = call "Elasped Timer.vi"("Time Setting"=5.0, "Action"=Elapsed_timer_control."Initialize") -> ()  [unwired: 6 in, 4 out]
        n157 = Bundle By Name(cluster=w2744, "Time up flag"=FALSE) -> (w2742:T15)
      }
      frame "START TIMER" {
        # ">>State Logic  >>"
        # ">>> Time cluster >>>"
        # ">>> Yaw >>>"
        # ">>> Stepper position >>>"
        # ">>> Encoders >>>"
        # ">>> Object detection >>>"
        # ">>> Ultrasonic Sensors Detect >>>"
        n158 = call "Elasped Timer.vi"("Action"=Elapsed_timer_control."Start") -> ("Time Out?!"=w2753:bool)  [unwired: 7 in, 3 out]
        n159 = Bundle By Name(cluster=w2756, "Time up flag"=w2753) -> (w2755:T15)
      }
    }
    "State Logic" <- w231
    "Image Processing Error" <- w198
    n160 = local read "TASK ENABLE"() -> (w225:bool)
    n161 = Not(x=w225) -> (.not. x?=w224:bool)
    n162 = case shown="True" w232 {
      tunnel: w236 -> [w262 w300]
      tunnel: w240 -> [w258 w302]
      tunnel: [w262 w300] -> w245
      tunnel: [w258 w303] -> w244
      tunnel: w241 -> [_ w298]
      tunnel: w243 -> [_ w299]
      tunnel: w238 -> [w261 w305]
      tunnel: [w261 w305] -> w237
      tunnel: "STOP TASK" -> [_ w288]
      tunnel: w231 -> [w260 w304]
      tunnel: [w260 w301] -> w230
      tunnel: w227 -> [w259 w294]
      tunnel: [w259 w294] -> w226
      tunnel: w224 -> [_ w289]
      tunnel: [w257 w286] -> w223
      tunnel: w222 -> [w257 w285]
      tunnel: w220 -> [w256 w282]
      tunnel: [w256 w282] -> w219
      tunnel: w217 -> [w255 w278]
      tunnel: [w255 w278] -> w216
      tunnel: w214 -> [w254 w276]
      tunnel: [w254 w276] -> w213
      tunnel: w211 -> [w253 w274]
      tunnel: [w253 w274] -> w210
      tunnel: w209 -> [w252 w273]
      tunnel: [w252 w272] -> w208
      tunnel: [_ w270] -> w207
      tunnel: w205 -> [w251 w268]
      tunnel: [w251 w268] -> w204
      tunnel: w203 -> [w250 w267]
      tunnel: [w250 w266] -> w202
      tunnel: w200 -> [w249 w263]
      tunnel: [w249 w263] -> w199
      frame False {
        # ">>> Line Sensor Cluster>>>"
        # ">>> Line Sensor Cluster>>>"
        # ">>> Motor control cluster >>>"
        # ">>> yStepper command>>>"
        # ">>> Motor control cluster >>>"
        # ">>> yStepper command>>>"
        # ">>> Motor control cluster >>>"
        # ">>> IR Sensors >>>"
        # ">>> IR Sensors >>>"
        # ">>> yStepper command>>>"
        # ">>> Time cluster >>>"
        # ">>> Yaw >>>"
        # ">>> Stepper position >>>"
        # ">>> Encoders >>>"
        # ">>> Object detection >>>"
        # ">>> Ultrasonic Sensors Detect >>>"
        # ">>> Time cluster >>>"
        # ">>> Yaw >>>"
        # ">>> Stepper position >>>"
        # ">>> Encoders >>>"
        # ">>> Object detection >>>"
        # ">>> Ultrasonic Sensors Detect >>>"
      }
      frame True {
        # ">>> IR Sensors >>>"
        # ">>> Line Sensor Cluster>>>"
        # ">>> Line Sensor Cluster>>>"
        # ">>> Motor control cluster >>>"
        # ">>> yStepper command>>>"
        # ">>> IR Sensors >>>"
        # ">>> Motor control cluster >>>"
        # ">>State Logic Queue Reference >>"
        # ">>Timeout>>"
        # ">>> yStepper command>>>"
        # ">>> Time cluster >>>"
        # ">>> Object detection >>>"
        # ">>> Yaw >>>"
        # ">>> Ultrasonic Sensors Detect >>>"
        # ">>> Encoders >>>"
        # ">>> Stepper position >>>"
        # ">>State Logic  >>"
        # ">>True Stop Next State >>"
        # ">>Action Queue>>"
        # ">> Manual override >>"
        # ">>> Time cluster >>>"
        # ">>> Yaw >>>"
        # ">>> Stepper position >>>"
        # ">>> Encoders >>>"
        # ">>> Object detection >>>"
        # ">>> Ultrasonic Sensors Detect >>>"
        # ">>Action Queue>>"
        # ">>State Logic Queue Reference >>"
        n163 = Or(x=w288, y=w289) -> (x .or. y?=w287:bool)
        n164 = Unbundle By Name(w268) -> ("Left IR Sensor"=w269:dbl, "Arm IR Sensor"=w265:dbl)
        "Left IR Sensor" <- w269
        "Arm IR Sensor" <- w265
        n165 = Unbundle By Name(w274) -> ("Time up flag"=w275:bool)
        "Time up flag" <- w275
        n166 = Unbundle By Name(w276) -> ("Yaw"=w277:dbl, "Compass"=w271:dbl)
        n167 = Unbundle By Name(w278) -> ("y Stepper Position"=w280:u8, "z Stepper Position"=w279:u8)
        n168 = Unbundle By Name(w294) -> ("xDistance"=w291:dbl, "yDistance"=w292:dbl, "wDistance"=w293:dbl)
        n169 = Unbundle By Name(w282) -> ("Recognized Object"=w281:bool, "Object X coordinate"=w284:dbl, "Object Y coordinate"=w283:dbl)
        n170 = Unbundle By Name(w305) -> ("PING_A"=w297:u8, "PING_B"=w296:u8, "PING_C"=w295:u8, "PING_D"=w290:u8)
        n171 = Unbundle By Name(w263) -> ("Line Detected?"=w264:bool)
        n172 = case shown="42" w304 {
          tunnel: [w309 w320 w333 w343 w425 w439 w475 w528 w570 w617 w660 w714 w761 w801 w861 w906 w946 w994 w1036 w1088 w1125 w1176 w1219 w1262 w1291 w1308 w1353 w1393 w1441 w1493 w1531 w1579 w1621 w1673 w1710 w1761 w1796 w1844 w1886 w1931 w1976 w2019 w2073] -> w303
          tunnel: w302 -> [w309 w323 w334 w346 w427 w440 w484 w526 w574 w618 w666 w707 w764 w808 w851 w909 w952 w993 w1039 w1078 w1131 w1166 w1214 w1253 w1291 w1298 w1356 w1399 w1440 w1492 w1537 w1578 w1624 w1663 w1716 w1751 w1800 w1851 w1891 w1936 w1981 w2023 w2071]
          tunnel: [State_Type_Definitions,_for_0.26g_versions_and_later_2."Idle" ("Enum") State_Type_Definitions,_for_0.26g_versions_and_later_2."Idle" ("Enum") w329 w345 State_Type_Definitions,_for_0.26g_versions_and_later_2."Shutdown" ("Enum") w441 w482 w529 w571 w616 w661 w713 w762 w803 w860 w907 w953 w995 w1038 w1087 w1132 w1175 w1220 w1254 State_Type_Definitions,_for_0.26g_versions_and_later_2."Idle" ("Enum") w1307 w1354 w1400 w1442 w1494 w1538 w1580 w1623 w1672 w1717 w1760 w1797 w1845 w1887 w1932 w1977 w2020 w2074] -> w301
          tunnel: w300 -> [_ _ w332 w349 _ w446 w478 w525 w575 w625 w665 w711 w765 w807 w858 w904 w951 w991 w1040 w1085 w1130 w1173 w1217 w1261 _ w1305 w1351 w1398 w1438 w1490 w1536 w1576 w1625 w1670 w1715 w1758 w1804 w1850 w1894 w1939 w1984 w2027 w2070]
          tunnel: w299 -> [_ _ _ w348 _ w445 w477 w524 w576 w624 w664 w710 w758 w806 w857 w903 w950 w990 w1041 w1084 w1129 w1172 w1216 w1259 _ w1304 w1350 w1397 w1437 w1489 w1535 w1575 w1626 w1669 w1714 w1757 w1799 w1849 w1893 w1938 w1983 w2022 w2069]
          tunnel: w298 -> [_ _ w331 w344 _ w444 w476 w523 w577 w623 w663 w709 w757 w805 w859 w905 w949 w989 w1042 w1086 w1128 w1174 w1215 w1260 _ w1306 w1352 w1396 w1436 w1488 w1534 w1574 w1627 w1671 w1713 w1759 w1803 w1848 w1892 w1937 w1982 w2026 w2068]
          tunnel: w287 -> [_ _ _ _ _ w438 w483 w522 w578 w620 w659 w712 w763 w809 w852 w910 w947 w992 w1043 w1079 w1126 w1167 w1218 w1257 _ w1299 w1357 w1394 w1439 w1491 w1532 w1577 w1628 w1664 w1711 w1752 w1802 w1843 w1890 w1935 w1980 w2025 w2067]
          tunnel: w297 -> [_ _ _ _ _ _ _ _ _ _ _ _ _ _ _ _ _ _ _ _ _ _ _ _ _ _ _ _ _ _ _ _ _ _ _ _ _ _ _ _ _ _ _]
          tunnel: w296 -> [_ _ _ _ _ _ _ w521 _ _ _ w703 w746 w799 _ w896 _ _ _ _ _ _ _ _ _ _ w1343 _ _ _ _ _ _ _ _ _ _ _ _ _ _ _ _]
          tunnel: w295 -> [_ _ _ _ _ _ _ w520 _ _ _ w704 w747 w800 _ w897 _ _ _ _ _ _ _ _ _ _ w1344 _ _ _ _ _ _ _ _ _ _ _ _ _ _ _ _]
          tunnel: w293 -> [_ _ _ _ _ _ _ _ _ w622 _ _ _ _ _ _ _ _ _ _ _ _ _ _ _ _ _ _ _ _ _ _ _ _ _ _ _ _ _ _ _ _ _]
          tunnel: w292 -> [_ _ _ _ _ w437 _ _ w569 _ _ _ _ w804 _ _ _ _ _ _ _ _ _ _ _ _ _ _ _ _ _ _ _ _ _ _ _ _ _ _ _ _ _]
          tunnel: w291 -> [_ _ _ _ _ _ _ _ _ _ _ _ w752 _ _ _ _ _ _ _ _ _ _ _ _ _ _ _ _ w1479 _ _ _ _ _ _ _ _ _ _ w1974 _ _]
          tunnel: w290 -> [_ _ _ _ _ _ _ _ _ _ _ _ _ _ _ _ _ _ _ _ _ _ _ _ _ _ _ _ _ _ _ _ _ _ _ _ _ _ _ _ _ _ _]
          tunnel: [State_Type_Definitions,_for_0.26g_versions_and_later_2."Idle" ("Enum") State_Type_Definitions,_for_0.26g_versions_and_later_2."Idle" ("Enum") State_Type_Definitions,_for_0.26g_versions_and_later_2."Idle" ("Enum") State_Type_Definitions,_for_0.26g_versions_and_later_2."Idle" ("Enum") State_Type_Definitions,_for_0.26g_versions_and_later_2."Shutdown" ("Enum") w434 w481 w527 w572 w613 w658 w706 w760 w802 w862 w908 w945 w996 w1037 w1089 w1124 w1177 w1221 w1255 w1293 w1309 w1355 w1392 w1443 w1495 w1530 w1581 w1622 w1674 w1709 w1762 w1798 w1846 w1889 w1934 w1979 w2021 w2072] -> w286
          tunnel: w285 -> [_ _ w329 _ _ _ _ _ _ _ _ _ _ _ _ _ _ _ _ _ _ _ _ _ w1293 _ _ _ _ _ _ _ _ _ _ _ _ _ _ _ _ _ _]
          tunnel: w281 -> [_ _ _ _ _ _ _ _ _ _ _ _ _ _ _ _ _ _ _ _ _ _ _ w1256 _ _ _ _ _ _ _ _ _ _ _ _ _ _ _ _ _ _ _]
          tunnel: w284 -> [_ _ _ _ _ _ _ _ _ _ _ _ _ _ _ _ _ _ _ _ _ _ _ _ _ _ _ _ _ w1485 _ _ _ _ _ _ _ _ _ _ _ _ _]
          tunnel: w283 -> [_ _ _ _ _ _ _ _ _ _ _ _ _ _ _ _ _ _ w1032 _ _ _ _ _ _ _ _ _ _ _ _ _ w1617 _ _ _ _ _ _ _ _ _ _]
          tunnel: w280 -> [_ _ _ _ _ _ _ _ _ _ _ _ _ _ _ _ _ _ w1031 _ _ _ _ _ _ _ _ _ _ _ _ _ w1616 _ _ _ _ _ _ _ _ _ _]
          tunnel: w279 -> [_ _ _ _ _ _ w480 _ _ _ w656 _ _ _ w855 _ _ _ _ w1082 _ w1170 w1213 _ _ w1302 _ _ _ _ _ _ _ w1667 _ w1755 w1801 _ _ _ _ w2024 _]
          tunnel: w277 -> [_ _ _ _ _ _ _ _ _ _ _ _ _ _ _ _ _ _ _ _ _ _ _ _ _ _ _ _ _ _ _ _ _ _ _ _ _ _ _ _ _ _ _]
          tunnel: w275 -> [_ _ _ _ _ _ _ _ _ _ _ _ _ _ _ _ w943 w986 _ _ w1122 _ _ _ _ _ _ w1390 w1433 _ w1528 w1571 _ _ w1707 _ _ _ _ _ _ _ _]
          tunnel: w273 -> [w307 w318 w328 w341 w423 w433 w479 w519 w573 w612 w657 w705 w756 w798 w850 w901 w944 w987 w1034 w1077 w1123 w1165 w1210 w1252 w1294 w1297 w1348 w1391 w1434 w1486 w1529 w1572 w1619 w1662 w1708 w1750 w1795 w1847 w1888 w1933 w1978 w2018 w2066]
          tunnel: [w307 w317 w328 w341 w423 w433 w479 w519 w573 w612 w657 w705 w756 w798 w850 w901 w944 w987 w1033 w1077 w1123 w1165 w1210 w1252 w1294 w1297 w1348 w1391 w1434 w1486 w1529 w1572 w1618 w1662 w1708 w1750 w1795 w1847 w1888 w1933 w1978 w2018 w2066] -> w272
          tunnel: w271 -> [_ _ _ _ _ _ _ _ _ _ _ _ _ _ _ _ _ _ _ _ _ _ _ _ _ _ _ _ _ _ _ _ _ _ _ _ _ w1842 _ _ _ _ _]
          tunnel: [_ _ _ TRUE _ _ _ _ _ _ _ _ _ _ _ _ _ _ _ _ _ _ _ _ _ _ _ _ _ _ _ _ _ _ _ _ _ _ _ _ _ _ _] -> w270
          tunnel: w269 -> [_ _ _ _ _ _ _ _ _ _ _ _ _ _ _ _ _ _ _ _ _ _ _ _ _ _ _ _ _ _ _ _ _ _ _ _ _ _ _ _ _ _ _]
          tunnel: w267 -> [w306 w315 w327 w339 w422 w432 w474 w518 w566 w611 w653 w698 w745 w797 w849 w894 w942 w985 w1028 w1076 w1121 w1164 w1209 w1251 w1295 w1296 w1341 w1389 w1432 w1482 w1527 w1570 w1613 w1661 w1706 w1749 w1794 w1838 w1885 w1930 w1975 w2017 w2065]
          tunnel: [w306 w314 w327 w339 w422 w432 w474 w518 w566 w611 w653 w698 w745 w797 w849 w894 w942 w985 w1028 w1076 w1121 w1164 w1209 w1251 w1295 w1296 w1341 w1389 w1432 w1481 w1527 w1570 w1613 w1661 w1706 w1749 w1794 w1838 w1885 w1930 w1975 w2017 w2065] -> w266
          tunnel: w265 -> [_ _ _ _ _ _ _ _ _ _ _ _ _ _ _ _ _ _ _ _ _ _ _ _ _ _ _ _ _ _ _ _ _ _ _ _ _ _ _ w1928 _ _ w2064]
          tunnel: w264 -> [_ _ _ _ _ _ _ _ _ _ _ _ _ _ _ _ _ _ _ _ _ _ _ _ _ _ _ _ _ _ _ _ _ _ _ _ _ _ w1884 _ _ _ _]
          frame 0 {
            # ">>> yStepper command>>>"
          }
          frame 1 {
            # ">>> yStepper command>>>"
            n173 = for {
              shift-right: [w326] -> w320
              shift-left: w323 -> [w325]
              tunnel: string[] ["INIT", "RESET ARM", "RESET FLAGS", "RESET YAW", "NAVX CALIBRATE"] -> [w324] mode=indexing
              n174 = Enqueue Element(queue=w325, element=w324) -> (queue out=w326:refnum<queue>)  [unwired: 2 in, 2 out]
            }
            n175 = Bundle By Name(cluster=w318, "yStepper desired"=u8 0) -> (w317:T14)
            n176 = Bundle By Name(cluster=w315, "ySpeed"=0.0, "xSpeed"=0.0, "wSpeed"=0.0) -> (w314:T12)
          }
          frame 3 {
            # ">>> Motor control cluster >>>"
            # ">>> yStepper command>>>"
            n177 = Flush Queue(queue=w332, error in (no error)=w331) -> ()  [unwired: 3 out]
            n178 = for {
              shift-right: [w338] -> w333
              shift-left: w334 -> [w337]
              tunnel: string[] ["STOP", "RESET ENCODERS", "RESET YAW", "RESET ARM", "RESET FLAGS", "DISPOSE CAM BUFFERS", "DISPOSE PROC BUFFERS", "CAM CLOSE", ""] -> [w336] mode=indexing
              n179 = Enqueue Element(queue=w337, element=w336) -> (queue out=w338:refnum<queue>)  [unwired: 2 in, 2 out]
            }
          }
          frame 4, Default {
            (unwired) TRUE ("Green LED")
            # ">>> yStepper command>>>"
            n180 = Dequeue Element(queue=w349, timeout in ms (-1)=w348, error in (no error)=w344) -> (element=w347:T10)  [unwired: 3 out]
            n181 = case shown="\"Start Task 9\"" w347 {
              tunnel: [w351 w358 w365 w372 w379 w386 w393 w395 w403 w410 w416] -> w343
              tunnel: w346 -> [w352 w359 w366 w373 w380 w387 w393 w396 w402 w409 w417]
              tunnel: [State_Type_Definitions."Task 1" ("Enum") State_Type_Definitions,_for_0.26g_versions_and_later_2."Task 2:Raise Arm" ("Enum") State_Type_Definitions,_for_0.26g_versions_and_later_2."Task 3" ("Enum") State_Type_Definitions,_for_0.26g_versions_and_later_2."Task 4_A" ("Enum") State_Type_Definitions."Task 5A: ARM CAM HEIGHT" ("Enum") State_Type_Definitions,_for_0.26g_versions_and_later_2."Task 6_A" ("Enum") State_Type_Definitions,_for_0.26g_versions_and_later_2."Idle" ("Enum") State_Type_Definitions,_for_0.26g_versions_and_later_2."Shutdown" ("Enum") State_Type_Definitions,_for_0.26g_versions_and_later_2."Task 9A: Raise Arm" ("Enum") State_Type_Definitions."Task A: RAISE ARM TO HEIGHT" ("Enum") State_Type_Definitions,_for_0.26g_versions_and_later_2."Task 8A: RAISE ARM" ("Enum")] -> w345
              frame "Start Task 1" {
                n182 = for {
                  shift-right: [w356] -> w351
                  shift-left: w352 -> [w355]
                  tunnel: string[] ["RESET ENCODERS", "RESET YAW", "FORWARD", "READ ENCODERS"] -> [w354] mode=indexing
                  n183 = Enqueue Element(queue=w355, element=w354) -> (queue out=w356:refnum<queue>)  [unwired: 2 in, 2 out]
                }
              }
              frame "Start Task 2" {
                n184 = for {
                  shift-right: [w363] -> w358
                  shift-left: w359 -> [w362]
                  tunnel: string[] ["RESET ENCODERS", "RESET YAW", "READ ULTRASONIC", "ARDUINO - ULTRASONIC"] -> [w361] mode=indexing
                  n185 = Enqueue Element(queue=w362, element=w361) -> (queue out=w363:refnum<queue>)  [unwired: 2 in, 2 out]
                }
              }
              frame "Start Task 3" {
                n186 = for {
                  shift-right: [w370] -> w365
                  shift-left: w366 -> [w369]
                  tunnel: string[] ["RESET ENCODERS", "READ ENCODERS", "R-ACW"] -> [w368] mode=indexing
                  n187 = Enqueue Element(queue=w369, element=w368) -> (queue out=w370:refnum<queue>)  [unwired: 2 in, 2 out]
                }
              }
              frame "Start Task 4" {
                n188 = for {
                  shift-right: [w377] -> w372
                  shift-left: w373 -> [w376]
                  tunnel: string[] ["RESET YAW", "RESET ENCODERS", "RESET ARM", "RESET FLAGS", "", ""] -> [w375] mode=indexing
                  n189 = Enqueue Element(queue=w376, element=w375) -> (queue out=w377:refnum<queue>)  [unwired: 2 in, 2 out]
                }
              }
              frame "Start Task 5" {
                n190 = for {
                  shift-right: [w384] -> w379
                  shift-left: w380 -> [w383]
                  tunnel: string[] ["RESET YAW", "RESET ENCODERS", "READ STEPPER VALUES", "Z STEPPER CAM HEIGHT", "", ""] -> [w382] mode=indexing
                  n191 = Enqueue Element(queue=w383, element=w382) -> (queue out=w384:refnum<queue>)  [unwired: 2 in, 2 out]
                }
              }
              frame "Start Task 6" {
                n192 = for {
                  shift-right: [w391] -> w386
                  shift-left: w387 -> [w390]
                  tunnel: string[] ["OPEN LOG CAM ", "", "", "", "", ""] -> [w389] mode=indexing
                  n193 = Enqueue Element(queue=w390, element=w389) -> (queue out=w391:refnum<queue>)  [unwired: 2 in, 2 out]
                }
              }
              frame "None", Default {
              }
              frame "Exit" {
                n194 = for {
                  shift-right: [w400] -> w395
                  shift-left: w396 -> [w399]
                  tunnel: string[] ["STOP", "RESET ENCODERS", "RESET YAW", "EXIT"] -> [w398] mode=indexing
                  n195 = Enqueue Element(queue=w399, element=w398) -> (queue out=w400:refnum<queue>)  [unwired: 2 in, 2 out]
                }
              }
              frame "Start Task 9" {
                n196 = for {
                  shift-right: [w407] -> w403
                  shift-left: w402 -> [w406]
                  tunnel: string[] ["RESET ENCODERS", "READ ENCODERS", "Z STEPPER BOX HEIGHT"] -> [w405] mode=indexing
                  n197 = Enqueue Element(queue=w406, element=w405) -> (queue out=w407:refnum<queue>)  [unwired: 2 in, 2 out]
                }
              }
              frame "Start Task A" {
                n198 = for {
                  shift-right: [w414] -> w410
                  shift-left: w409 -> [w413]
                  tunnel: string[] ["RESET ENCODERS", "READ ENCODERS", "RESET YAW", "Z STEPPER BOX HEIGHT"] -> [w412] mode=indexing
                  n199 = Enqueue Element(queue=w413, element=w412) -> (queue out=w414:refnum<queue>)  [unwired: 2 in, 2 out]
                }
              }
              frame "Start Task 8 - Gel" {
                n200 = for {
                  shift-right: [w421] -> w416
                  shift-left: w417 -> [w420]
                  tunnel: string[] ["RESET YAW", "RESET ENCODERS", "RESET ARM", "RESET FLAGS"] -> [w419] mode=indexing
                  n201 = Enqueue Element(queue=w420, element=w419) -> (queue out=w421:refnum<queue>)  [unwired: 2 in, 2 out]
                }
              }
            }
          }
          frame 5 {
            # ">>> yStepper command>>>"
            n202 = for {
              shift-right: [w431] -> w425
              shift-left: w427 -> [w430]
              tunnel: string[] ["INIT", "RESET ENCODERS", "RESET FLAGS", "CAM CLOSE", "DISPOSE BUFFERS", "EXIT", ""] -> [w429] mode=indexing
              n203 = Enqueue Element(queue=w430, element=w429) -> (queue out=w431:refnum<queue>)  [unwired: 2 in, 2 out]
            }
          }
          frame 6 {
            # ">>> yStepper command>>>"
            # "Use 250"
            n204 = Dequeue Element(queue=w446, timeout in ms (-1)=w445, error in (no error)=w444) -> (element=w443:T10)  [unwired: 3 out]
            n205 = Greater?(x=w437, y=265.0) -> (0:w435:bool)
            n206 = Or(x=w435, y=w438) -> (x .or. y?=w442:bool)
            n207 = case shown="\"None\", Default" w443 {
              tunnel: w442 -> [w449 _]
              tunnel: [w453 State_Type_Definitions,_for_0.26g_versions_and_later_2."True Stop" ("Enum")] -> w441
              tunnel: w440 -> [w450 w468]
              tunnel: [w448 w467] -> w439
              tunnel: [State_Type_Definitions,_for_0.26g_versions_and_later_2."Idle" ("Enum") State_Type_Definitions,_for_0.26g_versions_and_later_2."Shutdown" ("Enum")] -> w434
              frame "None", Default {
                n208 = case shown="True" w449 {
                  tunnel: w450 -> [w456 w462]
                  tunnel: [w455 w460] -> w448
                  frame False {
                    n209 = for {
                      shift-right: [w458] -> w455
                      shift-left: w456 -> [w459]
                      tunnel: string[] ["READ ENCODERS", "READ NAVX", "FORWARD"] ("element") -> [w457] mode=indexing
                      n210 = Enqueue Element(queue=w459, element=w457) -> (queue out=w458:refnum<queue>)  [unwired: 2 in, 2 out]
                    }
                  }
                  frame True {
                    n211 = for {
                      shift-right: [w464] -> w460
                      shift-left: w462 -> [w465]
                      tunnel: string[] ["RESET YAW", "RESET ENCODERS", "STOP", ""] -> [w463] mode=indexing
                      n212 = Enqueue Element(queue=w465, element=w463) -> (queue out=w464:refnum<queue>)  [unwired: 2 in, 2 out]
                    }
                  }
                }
                n213 = Select(t=State_Type_Definitions,_for_0.26g_versions_and_later_2."True Stop" ("Enum"), s=w449, f=State_Type_Definitions."Task 1" ("Enum")) -> (s? t:f=w453:u16)
              }
              frame "Exit" {
                n214 = for {
                  shift-right: [w472] -> w467
                  shift-left: w468 -> [w473]
                  tunnel: string[] ["STOP", "RESET ENCODERS", "RESET YAW", ""] -> [w471] mode=indexing
                  n215 = Enqueue Element(queue=w473, element=w471) -> (queue out=w472:refnum<queue>)  [unwired: 2 in, 2 out]
                }
              }
            }
          }
          frame 8 {
            # ">> Stepper height reeached >>"
            # ">>> yStepper command>>>"
            # ">> Manual override >>"
            n216 = Dequeue Element(queue=w478, timeout in ms (-1)=w477, error in (no error)=w476) -> (element=w487:T10)  [unwired: 3 out]
            n217 = Equal?(x=w480, y=u8 60) -> (x = y?=w485:bool)
            n218 = case shown="\"None\", Default" w487 {
              tunnel: [w498 State_Type_Definitions,_for_0.26g_versions_and_later_2."True Stop" ("Enum")] -> w482
              tunnel: [w496 w513] -> w475
              tunnel: w484 -> [w495 _]
              tunnel: w483 -> [w489 _]
              tunnel: [State_Type_Definitions,_for_0.26g_versions_and_later_2."Idle" ("Enum") State_Type_Definitions,_for_0.26g_versions_and_later_2."Shutdown" ("Enum")] -> w481
              tunnel: w485 -> [w488 _]
              frame "None", Default {
                # ">> WIill proceed to part ii if not manual override >>"
                # ">>If ENABLE or Trigger is set to true>>"
                n219 = Or(x=w488, y=w489) -> (x .or. y?=w490:bool)
                n220 = case shown="True" w488 {
                  tunnel: [w501 w507] -> w496
                  tunnel: w495 -> [w500 w506]
                  frame False {
                    n221 = for {
                      shift-right: [w503] -> w501
                      shift-left: w500 -> [w504]
                      tunnel: string[] ["Z STEPPER CAM HEIGHT", "READ STEPPER VALUES"] ("element") -> [w502] mode=indexing
                      n222 = Enqueue Element(queue=w504, element=w502) -> (queue out=w503:refnum<queue>)  [unwired: 2 in, 2 out]
                    }
                  }
                  frame True {
                    n223 = for {
                      shift-right: [w509] -> w507
                      shift-left: w506 -> [w510]
                      tunnel: string[] ["ARDUINO - ULTRASONIC", "READ ULTRASONIC", "", "", "", ""] -> [w508] mode=indexing
                      n224 = Enqueue Element(queue=w510, element=w508) -> (queue out=w509:refnum<queue>)  [unwired: 2 in, 2 out]
                    }
                  }
                }
                n225 = Select(t=State_Type_Definitions,_for_0.26g_versions_and_later_2."True Stop" ("Enum"), s=w489, f=State_Type_Definitions,_for_0.26g_versions_and_later_2."Task 2:Sensor Mode" ("Enum")) -> (s? t:f=w492:T9)
                n226 = Select(t=w492, s=w490, f=State_Type_Definitions,_for_0.26g_versions_and_later_2."Task 2:Raise Arm" ("Enum")) -> (s? t:f=w498:T9)
              }
              frame "Exit" {
                n227 = for {
                  shift-right: [w516] -> w513
                  shift-left: _ -> [w517]
                  tunnel: string[] ["STOP", "RESET ENCODERS", "RESET YAW", ""] -> [w515] mode=indexing
                  n228 = Enqueue Element(queue=w517, element=w515) -> (queue out=w516:refnum<queue>)  [unwired: 2 in, 2 out]
                }
              }
            }
          }
          frame 9 {
            w533 = u8 20 ("y")
            # ">>> yStepper command>>>"
            # ">>Object detected>>"
            n229 = Dequeue Element(queue=w525, timeout in ms (-1)=w524, error in (no error)=w523) -> (element=w534:T10)  [unwired: 3 out]
            n230 = Less?(x=w521, y=w533) -> (x < y?=w532:bool)
            n231 = Less?(x=w520, y=w533) -> (x < y?=w531:bool)
            n232 = Or(x=w532, y=w531) -> (x .or. y?=w530:bool)
            "Obstacle detected" <- w530
            n233 = case shown="\"None\", Default" w534 {
              tunnel: w530 -> [w537 _]
              tunnel: [w544 State_Type_Definitions,_for_0.26g_versions_and_later_2."True Stop" ("Enum")] -> w529
              tunnel: w522 -> [w536 _]
              tunnel: w526 -> [w543 w560]
              tunnel: [w542 w561] -> w528
              tunnel: [State_Type_Definitions,_for_0.26g_versions_and_later_2."Idle" ("Enum") State_Type_Definitions,_for_0.26g_versions_and_later_2."Shutdown" ("Enum")] -> w527
              frame "None", Default {
                n234 = case shown="True" w537 {
                  tunnel: w543 -> [w547 w554]
                  tunnel: [w548 w553] -> w542
                  frame False {
                    n235 = for {
                      tunnel: string[] ["READ ULTRASONIC", "STOP"] ("element") -> [w549] mode=indexing
                      shift-right: [w551] -> w548
                      shift-left: w547 -> [w550]
                      n236 = Enqueue Element(queue=w550, element=w549) -> (queue out=w551:refnum<queue>)  [unwired: 2 in, 2 out]
                    }
                  }
                  frame True {
                    n237 = for {
                      shift-right: [w556] -> w553
                      shift-left: w554 -> [w557]
                      tunnel: string[] ["RESET ENCODERS", "READ NAVX", "READ ENCODERS"] -> [w555] mode=indexing
                      n238 = Enqueue Element(queue=w557, element=w555) -> (queue out=w556:refnum<queue>)  [unwired: 2 in, 2 out]
                    }
                  }
                }
                n239 = Or(x=w537, y=w536) -> (x .or. y?=w535:bool)
                n240 = Select(t=State_Type_Definitions,_for_0.26g_versions_and_later_2."True Stop" ("Enum"), s=w536, f=State_Type_Definitions,_for_0.26g_versions_and_later_2."Task 2:Reverse Mode" ("Enum")) -> (s? t:f=w538:T9)
                n241 = Select(t=w538, s=w535, f=State_Type_Definitions,_for_0.26g_versions_and_later_2."Task 2:Sensor Mode" ("Enum")) -> (s? t:f=w544:T9)
              }
              frame "Exit" {
                n242 = for {
                  shift-right: [w564] -> w561
                  shift-left: w560 -> [w565]
                  tunnel: string[] ["STOP", "RESET ENCODERS", "RESET YAW", "ARDUINO MODE 0"] -> [w563] mode=indexing
                  n243 = Enqueue Element(queue=w565, element=w563) -> (queue out=w564:refnum<queue>)  [unwired: 2 in, 2 out]
                }
              }
            }
          }
          frame 10 {
            # ">>> yStepper command>>>"
            n244 = Dequeue Element(queue=w575, timeout in ms (-1)=w576, error in (no error)=w577) -> (element=w579:T10)  [unwired: 3 out]
            n245 = Less?(x=w569, y=-50.0) -> (x < y?=w567:bool)
            n246 = case shown="\"None\", Default" w579 {
              tunnel: [w589 State_Type_Definitions,_for_0.26g_versions_and_later_2."True Stop" ("Enum")] -> w571
              tunnel: w578 -> [w582 _]
              tunnel: w574 -> [w588 w605]
              tunnel: [w587 w606] -> w570
              tunnel: [State_Type_Definitions,_for_0.26g_versions_and_later_2."Idle" ("Enum") State_Type_Definitions,_for_0.26g_versions_and_later_2."Shutdown" ("Enum")] -> w572
              tunnel: w567 -> [w580 _]
              frame "None", Default {
                n247 = case shown="False" w580 {
                  tunnel: w588 -> [w592 w599]
                  tunnel: [w593 w598] -> w587
                  frame False {
                    n248 = for {
                      tunnel: string[] ["READ ENCODERS", "REVERSE", "READ NAVX"] ("element") -> [w594] mode=indexing
                      shift-right: [w596] -> w593
                      shift-left: w592 -> [w595]
                      n249 = Enqueue Element(queue=w595, element=w594) -> (queue out=w596:refnum<queue>)  [unwired: 2 in, 2 out]
                    }
                  }
                  frame True {
                    n250 = for {
                      shift-right: [w601] -> w598
                      shift-left: w599 -> [w602]
                      tunnel: string[] ["STOP", "ARDUINO - ULTRASONIC", "READ ULTRASONIC", "RESET ENCODERS"] -> [w600] mode=indexing
                      n251 = Enqueue Element(queue=w602, element=w600) -> (queue out=w601:refnum<queue>)  [unwired: 2 in, 2 out]
                    }
                  }
                }
                n252 = Or(x=w580, y=w582) -> (x .or. y?=w581:bool)
                n253 = Select(t=State_Type_Definitions,_for_0.26g_versions_and_later_2."True Stop" ("Enum"), s=w582, f=State_Type_Definitions,_for_0.26g_versions_and_later_2."Task 2:Sensor Mode" ("Enum")) -> (s? t:f=w583:T9)
                n254 = Select(t=w583, s=w581, f=State_Type_Definitions,_for_0.26g_versions_and_later_2."Task 2:Reverse Mode" ("Enum")) -> (s? t:f=w589:T9)
              }
              frame "Exit" {
                n255 = for {
                  shift-right: [w609] -> w606
                  shift-left: w605 -> [w610]
                  tunnel: string[] ["STOP", "RESET ENCODERS", "RESET YAW", "ARDUINO MODE 0"] -> [w608] mode=indexing
                  n256 = Enqueue Element(queue=w610, element=w608) -> (queue out=w609:refnum<queue>)  [unwired: 2 in, 2 out]
                }
              }
            }
          }
          frame 11 {
            # ">>> yStepper command>>>"
            n257 = Dequeue Element(queue=w625, timeout in ms (-1)=w624, error in (no error)=w623) -> (element=w614:T10)  [unwired: 3 out]
            n258 = Greater?(x=w622, y=160.0) -> (0:w619:bool)
            n259 = Or(x=w619, y=w620) -> (x .or. y?=w615:bool)
            n260 = case shown="\"None\", Default" w614 {
              tunnel: w615 -> [w628 _]
              tunnel: [w632 State_Type_Definitions,_for_0.26g_versions_and_later_2."True Stop" ("Enum")] -> w616
              tunnel: w618 -> [w629 w648]
              tunnel: [w627 w647] -> w617
              tunnel: [State_Type_Definitions,_for_0.26g_versions_and_later_2."Idle" ("Enum") State_Type_Definitions,_for_0.26g_versions_and_later_2."Shutdown" ("Enum")] -> w613
              frame "None", Default {
                n261 = case shown="False" w628 {
                  tunnel: w629 -> [w635 w641]
                  tunnel: [w634 w639] -> w627
                  frame False {
                    n262 = for {
                      shift-right: [w637] -> w634
                      shift-left: w635 -> [w638]
                      tunnel: string[] ["READ ENCODERS", "R-CW"] ("element") -> [w636] mode=indexing
                      n263 = Enqueue Element(queue=w638, element=w636) -> (queue out=w637:refnum<queue>)  [unwired: 2 in, 2 out]
                    }
                  }
                  frame True {
                    n264 = for {
                      shift-right: [w643] -> w639
                      shift-left: w641 -> [w644]
                      tunnel: string[] ["RESET YAW", "RESET ENCODERS", "STOP", "ARDUINO MODE 0"] -> [w642] mode=indexing
                      n265 = Enqueue Element(queue=w644, element=w642) -> (queue out=w643:refnum<queue>)  [unwired: 2 in, 2 out]
                    }
                  }
                }
                n266 = Select(t=State_Type_Definitions,_for_0.26g_versions_and_later_2."True Stop" ("Enum"), s=w628, f=State_Type_Definitions,_for_0.26g_versions_and_later_2."Task 3" ("Enum")) -> (s? t:f=w632:T9)
              }
              frame "Exit" {
                n267 = for {
                  shift-right: [w651] -> w647
                  shift-left: w648 -> [w652]
                  tunnel: string[] ["STOP", "RESET ENCODERS", "RESET YAW", ""] -> [w650] mode=indexing
                  n268 = Enqueue Element(queue=w652, element=w650) -> (queue out=w651:refnum<queue>)  [unwired: 2 in, 2 out]
                }
              }
            }
          }
          frame 12 {
            # ">> Stepper height reeached >>"
            # ">>> yStepper command>>>"
            # ">> Manual override >>"
            n269 = Dequeue Element(queue=w665, timeout in ms (-1)=w664, error in (no error)=w663) -> (element=w662:T10)  [unwired: 3 out]
            n270 = Equal?(x=w656, y=u8 60) -> (x = y?=w654:bool)
            n271 = case shown="\"Exit\"" w662 {
              tunnel: [w677 State_Type_Definitions,_for_0.26g_versions_and_later_2."True Stop" ("Enum")] -> w661
              tunnel: [w675 w693] -> w660
              tunnel: w666 -> [w674 w690]
              tunnel: w659 -> [w668 _]
              tunnel: [State_Type_Definitions,_for_0.26g_versions_and_later_2."Idle" ("Enum") State_Type_Definitions,_for_0.26g_versions_and_later_2."Shutdown" ("Enum")] -> w658
              tunnel: w654 -> [w667 _]
              frame "None", Default {
                # ">> WIill proceed to part ii if not manual override >>"
                # ">>If ENABLE or Trigger is set to true>>"
                n272 = Or(x=w667, y=w668) -> (x .or. y?=w669:bool)
                n273 = case shown="False" w667 {
                  tunnel: [w680 w686] -> w675
                  tunnel: w674 -> [w679 w685]
                  frame False {
                    n274 = for {
                      shift-right: [w682] -> w680
                      shift-left: w679 -> [w683]
                      tunnel: string[] ["Z STEPPER CAM HEIGHT", "READ STEPPER VALUES"] ("element") -> [w681] mode=indexing
                      n275 = Enqueue Element(queue=w683, element=w681) -> (queue out=w682:refnum<queue>)  [unwired: 2 in, 2 out]
                    }
                  }
                  frame True {
                    n276 = for {
                      shift-right: [w688] -> w686
                      shift-left: w685 -> [w689]
                      tunnel: string[] ["ARDUINO - ULTRASONIC", "READ ULTRASONIC", "FORWARD", "", "", ""] -> [w687] mode=indexing
                      n277 = Enqueue Element(queue=w689, element=w687) -> (queue out=w688:refnum<queue>)  [unwired: 2 in, 2 out]
                    }
                  }
                }
                n278 = Select(t=State_Type_Definitions,_for_0.26g_versions_and_later_2."True Stop" ("Enum"), s=w668, f=State_Type_Definitions,_for_0.26g_versions_and_later_2."Task 4_B" ("Enum")) -> (s? t:f=w671:T9)
                n279 = Select(t=w671, s=w669, f=State_Type_Definitions,_for_0.26g_versions_and_later_2."Task 4_A" ("Enum")) -> (s? t:f=w677:T9)
              }
              frame "Exit" {
                n280 = for {
                  shift-right: [w696] -> w693
                  shift-left: w690 -> [w697]
                  tunnel: string[] ["STOP", "RESET ENCODERS", "RESET YAW", ""] -> [w695] mode=indexing
                  n281 = Enqueue Element(queue=w697, element=w695) -> (queue out=w696:refnum<queue>)  [unwired: 2 in, 2 out]
                }
              }
            }
          }
          frame 13 {
            w702 = u8 20
            # ">> Path blocked >>"
            # ">>> yStepper command>>>"
            # ">> Manual override >>"
            n282 = Dequeue Element(queue=w711, timeout in ms (-1)=w710, error in (no error)=w709) -> (element=w708:T10)  [unwired: 3 out]
            n283 = Less?(x=w704, y=w702) -> (x < y?=w699:bool)
            n284 = Less?(x=w703, y=w702) -> (x < y?=w700:bool)
            n285 = And(x=w700, y=w699) -> (x .and. y?=w701:bool)
            n286 = case shown="\"None\", Default" w708 {
              tunnel: [w725 State_Type_Definitions,_for_0.26g_versions_and_later_2."True Stop" ("Enum")] -> w713
              tunnel: [w723 w740] -> w714
              tunnel: w707 -> [w722 _]
              tunnel: w712 -> [w716 _]
              tunnel: [State_Type_Definitions,_for_0.26g_versions_and_later_2."Idle" ("Enum") State_Type_Definitions,_for_0.26g_versions_and_later_2."Shutdown" ("Enum")] -> w706
              tunnel: w701 -> [w715 _]
              frame "None", Default {
                # ">> Manual override forces program to true stop >>"
                # ">>If ENABLE or Trigger is set to true>>"
                n287 = Or(x=w715, y=w716) -> (x .or. y?=w721:bool)
                n288 = case shown="True" w715 {
                  tunnel: [w728 w733] -> w723
                  tunnel: w722 -> [w727 w732]
                  frame False {
                    n289 = for {
                      shift-right: [w730] -> w728
                      shift-left: w727 -> [w731]
                      tunnel: string[] ["FORWARD", "READ ULTRASONIC", "READ NAVX"] ("element") -> [w729] mode=indexing
                      n290 = Enqueue Element(queue=w731, element=w729) -> (queue out=w730:refnum<queue>)  [unwired: 2 in, 2 out]
                    }
                  }
                  frame True {
                    n291 = for {
                      shift-right: [w736] -> w733
                      shift-left: w732 -> [w737]
                      tunnel: string[] ["STOP", "RESET YAW", "RESET ENCODERS", "RESET FLAGS"] -> [w735] mode=indexing
                      n292 = Enqueue Element(queue=w737, element=w735) -> (queue out=w736:refnum<queue>)  [unwired: 2 in, 2 out]
                    }
                  }
                }
                n293 = Select(t=State_Type_Definitions,_for_0.26g_versions_and_later_2."True Stop" ("Enum"), s=w716, f=State_Type_Definitions,_for_0.26g_versions_and_later_2."Task 4_C" ("Enum")) -> (s? t:f=w718:T9)
                n294 = Select(t=w718, s=w721, f=State_Type_Definitions,_for_0.26g_versions_and_later_2."Task 4_B" ("Enum")) -> (s? t:f=w725:T9)
              }
              frame "Exit" {
                n295 = for {
                  shift-right: [w743] -> w740
                  shift-left: _ -> [w744]
                  tunnel: string[] ["STOP", "RESET ENCODERS", "RESET YAW", ""] -> [w742] mode=indexing
                  n296 = Enqueue Element(queue=w744, element=w742) -> (queue out=w743:refnum<queue>)  [unwired: 2 in, 2 out]
                }
              }
            }
          }
          frame 14 {
            w755 = u8 20
            # ">> xDistance travelled>>"
            # ">> Path NOT blocked >>"
            # ">>> yStepper command>>>"
            # ">> Manual override >>"
            n297 = Dequeue Element(queue=w765, timeout in ms (-1)=w758, error in (no error)=w757) -> (element=w759:T10)  [unwired: 3 out]
            n298 = Greater?(x=w747, y=w755) -> (0:w753:bool)
            n299 = Greater?(x=w752, y=80.0) -> (0:w750:bool)
            n300 = Greater?(x=w746, y=w755) -> (0:w754:bool)
            n301 = And(x=w754, y=w753) -> (x .and. y?=w749:bool)
            n302 = And(x=w750, y=w749) -> (x .and. y?=w748:bool)
            n303 = case shown="\"Exit\"" w759 {
              tunnel: [w776 State_Type_Definitions,_for_0.26g_versions_and_later_2."True Stop" ("Enum")] -> w762
              tunnel: [w774 w792] -> w761
              tunnel: w764 -> [w773 w789]
              tunnel: w763 -> [w767 _]
              tunnel: [State_Type_Definitions,_for_0.26g_versions_and_later_2."Idle" ("t") State_Type_Definitions,_for_0.26g_versions_and_later_2."Shutdown" ("Enum")] -> w760
              tunnel: w748 -> [w766 _]
              frame "None", Default {
                # ">> Manual override forces program to true stop >>"
                # ">>If ENABLE or Trigger is set to true>>"
                n304 = Or(x=w766, y=w767) -> (x .or. y?=w772:bool)
                n305 = case shown="False" w766 {
                  tunnel: [w779 w784] -> w774
                  tunnel: w773 -> [w777 w783]
                  frame False {
                    n306 = for {
                      shift-right: [w781] -> w779
                      shift-left: w777 -> [w782]
                      tunnel: string[] ["RIGHT", "READ NAVX", "READ ENCODERS", "READ ULTRASONIC"] ("element") -> [w780] mode=indexing
                      n307 = Enqueue Element(queue=w782, element=w780) -> (queue out=w781:refnum<queue>)  [unwired: 2 in, 2 out]
                    }
                  }
                  frame True {
                    n308 = for {
                      shift-right: [w787] -> w784
                      shift-left: w783 -> [w788]
                      tunnel: string[] ["STOP", "RESET YAW", "RESET ENCODERS", "ARDUINO - ULTRASONIC"] -> [w786] mode=indexing
                      n309 = Enqueue Element(queue=w788, element=w786) -> (queue out=w787:refnum<queue>)  [unwired: 2 in, 2 out]
                    }
                  }
                }
                n310 = Select(t=State_Type_Definitions,_for_0.26g_versions_and_later_2."True Stop" ("Enum"), s=w767, f=State_Type_Definitions,_for_0.26g_versions_and_later_2."Task 4_D" ("Enum")) -> (s? t:f=w768:T9)
                n311 = Select(t=w768, s=w772, f=State_Type_Definitions,_for_0.26g_versions_and_later_2."Task 4_C" ("Enum")) -> (s? t:f=w776:T9)
              }
              frame "Exit" {
                n312 = for {
                  shift-right: [w795] -> w792
                  shift-left: w789 -> [w796]
                  tunnel: string[] ["STOP", "RESET ENCODERS", "RESET YAW", ""] -> [w794] mode=indexing
                  n313 = Enqueue Element(queue=w796, element=w794) -> (queue out=w795:refnum<queue>)  [unwired: 2 in, 2 out]
                }
              }
            }
          }
          frame 15 {
            w816 = u8 20
            # ">> yDistance travelled>>"
            # ">> Path blocked >>"
            # ">>> yStepper command>>>"
            # ">> Manual override >>"
            n314 = Dequeue Element(queue=w807, timeout in ms (-1)=w806, error in (no error)=w805) -> (element=w817:T10)  [unwired: 3 out]
            n315 = Less?(x=w800, y=w816) -> (x < y?=w814:bool)
            n316 = Greater?(x=w804, y=200.0) -> (0:w812:bool)
            n317 = Less?(x=w799, y=w816) -> (x < y?=w815:bool)
            n318 = And(x=w815, y=w814) -> (x .and. y?=w811:bool)
            n319 = Or(x=w812, y=w811) -> (x .or. y?=w810:bool)
            n320 = case shown="\"None\", Default" w817 {
              tunnel: [w828 State_Type_Definitions,_for_0.26g_versions_and_later_2."True Stop" ("Enum")] -> w803
              tunnel: [w826 w844] -> w801
              tunnel: w808 -> [w825 w841]
              tunnel: w809 -> [w819 _]
              tunnel: [State_Type_Definitions,_for_0.26g_versions_and_later_2."Idle" ("t") State_Type_Definitions,_for_0.26g_versions_and_later_2."Shutdown" ("Enum")] -> w802
              tunnel: w810 -> [w818 _]
              frame "None", Default {
                # ">> Manual override forces program to true stop >>"
                # ">>If ENABLE or Trigger is set to true>>"
                n321 = Or(x=w818, y=w819) -> (x .or. y?=w824:bool)
                n322 = case shown="True" w818 {
                  tunnel: [w831 w836] -> w826
                  tunnel: w825 -> [w829 w835]
                  frame False {
                    n323 = for {
                      shift-right: [w833] -> w831
                      shift-left: w829 -> [w834]
                      tunnel: string[] ["FORWARD", "READ NAVX", "READ ENCODERS", "READ ULTRASONIC"] ("element") -> [w832] mode=indexing
                      n324 = Enqueue Element(queue=w834, element=w832) -> (queue out=w833:refnum<queue>)  [unwired: 2 in, 2 out]
                    }
                  }
                  frame True {
                    n325 = for {
                      shift-right: [w839] -> w836
                      shift-left: w835 -> [w840]
                      tunnel: string[] ["STOP", "RESET YAW", "RESET ENCODERS", "RESET FLAGS"] -> [w838] mode=indexing
                      n326 = Enqueue Element(queue=w840, element=w838) -> (queue out=w839:refnum<queue>)  [unwired: 2 in, 2 out]
                    }
                  }
                }
                n327 = Select(t=State_Type_Definitions,_for_0.26g_versions_and_later_2."True Stop" ("Enum"), s=w819, f=State_Type_Definitions,_for_0.26g_versions_and_later_2."True Stop" ("Enum")) -> (s? t:f=w820:T9)
                n328 = Select(t=w820, s=w824, f=State_Type_Definitions,_for_0.26g_versions_and_later_2."Task 4_D" ("Enum")) -> (s? t:f=w828:T9)
              }
              frame "Exit" {
                n329 = for {
                  shift-right: [w847] -> w844
                  shift-left: w841 -> [w848]
                  tunnel: string[] ["STOP", "RESET ENCODERS", "RESET YAW", ""] -> [w846] mode=indexing
                  n330 = Enqueue Element(queue=w848, element=w846) -> (queue out=w847:refnum<queue>)  [unwired: 2 in, 2 out]
                }
              }
            }
          }
          frame 15 {
            # ">>> yStepper command>>>"
            # ">> Manual override >>"
            n331 = Dequeue Element(queue=w858, timeout in ms (-1)=w857, error in (no error)=w859) -> (element=w856:T10)  [unwired: 3 out]
            n332 = Equal?(x=w855, y=u8 60) -> (x = y?=w853:bool)
            n333 = case shown="\"None\", Default" w856 {
              tunnel: [w869 State_Type_Definitions,_for_0.26g_versions_and_later_2."True Stop" ("Enum")] -> w860
              tunnel: [w872 w889] -> w861
              tunnel: [State_Type_Definitions,_for_0.26g_versions_and_later_2."Idle" ("Enum") State_Type_Definitions,_for_0.26g_versions_and_later_2."Shutdown" ("Enum")] -> w862
              tunnel: w853 -> [w868 _]
              tunnel: w852 -> [w867 _]
              tunnel: w851 -> [w863 w886]
              frame "None", Default {
                # "Stays in Task 5_A until stepper reaches desired \nheight"
                # "T: Go back to idle, F: Continue with task\""
                # ">> Manual override >>"
                n334 = case shown="True" w868 {
                  tunnel: [w876 w882] -> w872
                  tunnel: w863 -> [w874 w880]
                  frame False {
                    n335 = for {
                      tunnel: string[] ["Z STEPPER CAM HEIGHT", "READ STEPPER VALUES"] ("element") -> [w877] mode=indexing
                      shift-right: [w879] -> w876
                      shift-left: w874 -> [w878]
                      n336 = Enqueue Element(queue=w878, element=w877) -> (queue out=w879:refnum<queue>)  [unwired: 2 in, 2 out]
                    }
                  }
                  frame True {
                    n337 = for {
                      shift-right: [w884] -> w882
                      shift-left: w880 -> [w885]
                      tunnel: string[] ["ARDUINO - ULTRASONIC", "READ ULTRASONIC", ""] -> [w883] mode=indexing
                      n338 = Enqueue Element(queue=w885, element=w883) -> (queue out=w884:refnum<queue>)  [unwired: 2 in, 2 out]
                    }
                  }
                }
                n339 = Or(x=w868, y=w867) -> (x .or. y?=w870:bool)
                n340 = Select(t=State_Type_Definitions,_for_0.26g_versions_and_later_2."True Stop" ("Enum"), s=w867, f=State_Type_Definitions."Task 5B: MOVE TO BOX" ("Enum")) -> (s? t:f=w864:u16)
                n341 = Select(t=w864, s=w870, f=State_Type_Definitions."Task 5A: ARM CAM HEIGHT" ("Enum")) -> (s? t:f=w869:u16)
              }
              frame "Exit" {
                n342 = for {
                  shift-right: [w892] -> w889
                  shift-left: w886 -> [w893]
                  tunnel: string[] ["STOP", "RESET ENCODERS", "RESET YAW", "ARDUINO MODE 0"] -> [w891] mode=indexing
                  n343 = Enqueue Element(queue=w893, element=w891) -> (queue out=w892:refnum<queue>)  [unwired: 2 in, 2 out]
                }
              }
            }
          }
          frame 16 {
            w900 = u8 20 ("y")
            # ">>> yStepper command>>>"
            n344 = Less?(x=w897, y=w900) -> (x < y?=w898:bool)
            n345 = Dequeue Element(queue=w904, timeout in ms (-1)=w903, error in (no error)=w905) -> (element=w902:T10)  [unwired: 3 out]
            n346 = Less?(x=w896, y=w900) -> (x < y?=w899:bool)
            n347 = And(x=w899, y=w898) -> (x .and. y?=w895:bool)
            n348 = case shown="\"None\", Default" w902 {
              tunnel: [w917 State_Type_Definitions,_for_0.26g_versions_and_later_2."True Stop" ("Enum")] -> w907
              tunnel: [w920 w937] -> w906
              tunnel: [State_Type_Definitions,_for_0.26g_versions_and_later_2."Idle" ("Enum") State_Type_Definitions,_for_0.26g_versions_and_later_2."Shutdown" ("Enum")] -> w908
              tunnel: w910 -> [w916 _]
              tunnel: w909 -> [w912 w934]
              tunnel: w895 -> [w911 _]
              frame "None", Default {
                # "Stays in Task 5_B to capture image over 5 seconds"
                # "T: Go back to idle, F: Continue with task\""
                # ">> Manual override >>"
                n349 = case shown="True" w911 {
                  tunnel: [w924 w930] -> w920
                  tunnel: w912 -> [w922 w928]
                  frame False {
                    n350 = for {
                      tunnel: string[] ["FORWARD", "READ ULTRASONIC", "READ NAVX"] ("element") -> [w925] mode=indexing
                      shift-right: [w927] -> w924
                      shift-left: w922 -> [w926]
                      n351 = Enqueue Element(queue=w926, element=w925) -> (queue out=w927:refnum<queue>)  [unwired: 2 in, 2 out]
                    }
                  }
                  frame True {
                    n352 = for {
                      shift-right: [w932] -> w930
                      shift-left: w928 -> [w933]
                      tunnel: string[] ["STOP", "RESET ENCODERS", "OPEN LOG CAM", "SET TIMER 5"] -> [w931] mode=indexing
                      n353 = Enqueue Element(queue=w933, element=w931) -> (queue out=w932:refnum<queue>)  [unwired: 2 in, 2 out]
                    }
                  }
                }
                n354 = Or(x=w911, y=w916) -> (x .or. y?=w918:bool)
                n355 = Select(t=State_Type_Definitions,_for_0.26g_versions_and_later_2."True Stop" ("Enum"), s=w916, f=State_Type_Definitions."Task 5C: CAM BURST" ("Enum")) -> (s? t:f=w913:u16)
                n356 = Select(t=w913, s=w918, f=State_Type_Definitions."Task 5B: MOVE TO BOX" ("Enum")) -> (s? t:f=w917:u16)
              }
              frame "Exit" {
                n357 = for {
                  shift-right: [w940] -> w937
                  shift-left: w934 -> [w941]
                  tunnel: string[] ["STOP", "RESET ENCODERS", "RESET YAW", "ARDUINO MODE 0"] -> [w939] mode=indexing
                  n358 = Enqueue Element(queue=w941, element=w939) -> (queue out=w940:refnum<queue>)  [unwired: 2 in, 2 out]
                }
              }
            }
          }
          frame 17 {
            # ">>> Motor control cluster >>>"
            # ">>> yStepper command>>>"
            # ">> Manual override >>"
            n359 = Dequeue Element(queue=w951, timeout in ms (-1)=w950, error in (no error)=w949) -> (element=w948:T10)  [unwired: 3 out]
            n360 = case shown="\"None\", Default" w948 {
              tunnel: [w960 State_Type_Definitions,_for_0.26g_versions_and_later_2."True Stop" ("Enum")] -> w953
              tunnel: [w963 w980] -> w946
              tunnel: [State_Type_Definitions,_for_0.26g_versions_and_later_2."Idle" ("Enum") State_Type_Definitions,_for_0.26g_versions_and_later_2."Shutdown" ("Enum")] -> w945
              tunnel: w947 -> [w954 _]
              tunnel: w952 -> [w959 w977]
              tunnel: w943 -> [w958 _]
              frame "None", Default {
                # ">> Is time up? >>"
                # "Determines if object is in range to pick up"
                # ">> Manual override >>"
                n361 = case shown="False" w958 {
                  tunnel: [w967 w973] -> w963
                  tunnel: w959 -> [w965 w971]
                  frame False {
                    n362 = for {
                      tunnel: string[] ["CAM ACQ", "START TIMER"] ("element") -> [w968] mode=indexing
                      shift-right: [w970] -> w967
                      shift-left: w965 -> [w969]
                      n363 = Enqueue Element(queue=w969, element=w968) -> (queue out=w970:refnum<queue>)  [unwired: 2 in, 2 out]
                    }
                  }
                  frame True {
                    n364 = for {
                      shift-right: [w975] -> w973
                      shift-left: w971 -> [w976]
                      tunnel: string[] ["CAM CLOSE", "PROCESS IMAGE", "SET TIMER 5"] -> [w974] mode=indexing
                      n365 = Enqueue Element(queue=w976, element=w974) -> (queue out=w975:refnum<queue>)  [unwired: 2 in, 2 out]
                    }
                  }
                }
                n366 = Or(x=w958, y=w954) -> (x .or. y?=w961:bool)
                n367 = Select(t=State_Type_Definitions,_for_0.26g_versions_and_later_2."True Stop" ("Enum"), s=w954, f=State_Type_Definitions."Task 5D: PROCESS IMAGE" ("Enum")) -> (s? t:f=w956:u16)
                n368 = Select(t=w956, s=w961, f=State_Type_Definitions."Task 5C: CAM BURST" ("Enum")) -> (s? t:f=w960:u16)
              }
              frame "Exit" {
                n369 = for {
                  shift-right: [w983] -> w980
                  shift-left: w977 -> [w984]
                  tunnel: string[] ["STOP", "RESET ENCODERS", "RESET YAW", "ARDUINO MODE 0"] -> [w982] mode=indexing
                  n370 = Enqueue Element(queue=w984, element=w982) -> (queue out=w983:refnum<queue>)  [unwired: 2 in, 2 out]
                }
              }
            }
          }
          frame 18 {
            # ">>> yStepper command>>>"
            n371 = Dequeue Element(queue=w991, timeout in ms (-1)=w990, error in (no error)=w989) -> (element=w988:T10)  [unwired: 3 out]
            n372 = case shown="\"None\", Default" w988 {
              tunnel: [w1003 State_Type_Definitions,_for_0.26g_versions_and_later_2."True Stop" ("Enum")] -> w995
              tunnel: [w1006 w1023] -> w994
              tunnel: [State_Type_Definitions,_for_0.26g_versions_and_later_2."Idle" ("Enum") State_Type_Definitions,_for_0.26g_versions_and_later_2."Shutdown" ("Enum")] -> w996
              tunnel: w992 -> [w1002 _]
              tunnel: w993 -> [w998 w1020]
              tunnel: w986 -> [w997 _]
              frame "None", Default {
                # ">> T: Breaks out of state loop; F: Stays in loop>>"
                # ">> Manual override >>"
                # ">> Checks if time is up>>"
                # "Stays in Task 5D until the object is detected"
                # "T: Go back to idle, F: Continue with task\""
                # ">> Manual override >>"
                n373 = case shown="True" w997 {
                  tunnel: [w1010 w1016] -> w1006
                  tunnel: w998 -> [w1008 w1014]
                  frame False {
                    n374 = for {
                      tunnel: string[] ["START TIMER", "PROCESS IMAGE", ""] ("element") -> [w1011] mode=indexing
                      shift-right: [w1013] -> w1010
                      shift-left: w1008 -> [w1012]
                      n375 = Enqueue Element(queue=w1012, element=w1011) -> (queue out=w1013:refnum<queue>)  [unwired: 2 in, 2 out]
                    }
                  }
                  frame True {
                    n376 = for {
                      shift-right: [w1018] -> w1016
                      shift-left: w1014 -> [w1019]
                      tunnel: string[] ["CAM CLOSE", "", ""] -> [w1017] mode=indexing
                      n377 = Enqueue Element(queue=w1019, element=w1017) -> (queue out=w1018:refnum<queue>)  [unwired: 2 in, 2 out]
                    }
                  }
                }
                n378 = Or(x=w997, y=w1002) -> (x .or. y?=w1004:bool)
                n379 = Select(t=State_Type_Definitions,_for_0.26g_versions_and_later_2."True Stop" ("Enum"), s=w1002, f=State_Type_Definitions,_for_0.26g_versions_and_later_2."Task 5E: POSITION ARM" ("Enum")) -> (s? t:f=w999:T9)
                n380 = Select(t=w999, s=w1004, f=State_Type_Definitions."Task 5D: PROCESS IMAGE" ("Enum")) -> (s? t:f=w1003:u16)
              }
              frame "Exit" {
                n381 = for {
                  shift-right: [w1026] -> w1023
                  shift-left: w1020 -> [w1027]
                  tunnel: string[] ["STOP", "RESET ENCODERS", "RESET YAW", "ARDUINO MODE 0"] -> [w1025] mode=indexing
                  n382 = Enqueue Element(queue=w1027, element=w1025) -> (queue out=w1026:refnum<queue>)  [unwired: 2 in, 2 out]
                }
              }
            }
          }
          frame 20 {
            # ">>> yStepper command>>>"
            n383 = Dequeue Element(queue=w1040, timeout in ms (-1)=w1041, error in (no error)=w1042) -> (element=w1044:T10)  [unwired: 3 out]
            n384 = formula code="if (pos < 100)\ny = 41;\n\nelse if (pos >= 100 && pos <= 140)\ny = 30;\n\nelse if (pos >= 141 && pos <= 170)\ny = 25;\n\nelse if (pos >= 171 &&pos <= 180) \ny = 20;\n\nelse if (pos >= 181&& pos <= 200)\ny = 15;\n\nelse if (pos >= 201 && pos <= 230)\ny = 10;\n\nelse if (pos >= 231 && pos <= 320)\ny = 8;\n\nelse if (pos > 320)\ny = 0;"("pos"=w1032) -> ("y"=w1035:dbl)
            n385 = To Unsigned Byte Integer(number=w1035) -> (unsigned 8bit integer=w1030:u8)
            n386 = Equal?(x=w1031, y=w1030) -> (x = y?=w1029:bool)
            n387 = case shown="\"None\", Default" w1044 {
              tunnel: [w1051 State_Type_Definitions,_for_0.26g_versions_and_later_2."True Stop" ("Enum")] -> w1038
              tunnel: [w1054 w1071] -> w1036
              tunnel: [State_Type_Definitions,_for_0.26g_versions_and_later_2."Idle" ("Enum") State_Type_Definitions,_for_0.26g_versions_and_later_2."Shutdown" ("Enum")] -> w1037
              tunnel: w1043 -> [w1050 _]
              tunnel: w1039 -> [w1046 w1068]
              tunnel: w1029 -> [w1045 _]
              frame "None", Default {
                # ">> T: Breaks out of state loop; F: Stays in loop>>"
                # ">> Manual override >>"
                # ">> Checks if time is up>>"
                # "Stays in Task 5D until the object is detected"
                # "T: Go back to idle, F: Continue with task\""
                # ">> Manual override >>"
                n388 = case shown="False" w1045 {
                  tunnel: [w1058 w1064] -> w1054
                  tunnel: w1046 -> [w1056 w1062]
                  frame False {
                    n389 = for {
                      tunnel: string[] ["READ STEPPER VALUES", "Y STEPPER CONTROL", ""] ("element") -> [w1059] mode=indexing
                      shift-right: [w1061] -> w1058
                      shift-left: w1056 -> [w1060]
                      n390 = Enqueue Element(queue=w1060, element=w1059) -> (queue out=w1061:refnum<queue>)  [unwired: 2 in, 2 out]
                    }
                  }
                  frame True {
                    n391 = for {
                      shift-right: [w1066] -> w1064
                      shift-left: w1062 -> [w1067]
                      tunnel: string[] ["CAM CLOSE", "DISPOSE BUFFERS", ""] -> [w1065] mode=indexing
                      n392 = Enqueue Element(queue=w1067, element=w1065) -> (queue out=w1066:refnum<queue>)  [unwired: 2 in, 2 out]
                    }
                  }
                }
                n393 = Or(x=w1045, y=w1050) -> (x .or. y?=w1052:bool)
                n394 = Select(t=State_Type_Definitions,_for_0.26g_versions_and_later_2."True Stop" ("Enum"), s=w1050, f=State_Type_Definitions,_for_0.26g_versions_and_later_2."Task 5F: ARM GRAB HEIGHT" ("Enum")) -> (s? t:f=w1047:T9)
                n395 = Select(t=w1047, s=w1052, f=State_Type_Definitions,_for_0.26g_versions_and_later_2."Task 5E: POSITION ARM" ("Enum")) -> (s? t:f=w1051:T9)
              }
              frame "Exit" {
                n396 = for {
                  shift-right: [w1074] -> w1071
                  shift-left: w1068 -> [w1075]
                  tunnel: string[] ["STOP", "RESET ENCODERS", "RESET YAW", "ARDUINO MODE 0"] -> [w1073] mode=indexing
                  n397 = Enqueue Element(queue=w1075, element=w1073) -> (queue out=w1074:refnum<queue>)  [unwired: 2 in, 2 out]
                }
              }
            }
            n398 = Bundle By Name(cluster=w1034, "yStepper desired"=w1030) -> (w1033:T14)
          }
          frame 21 {
            # ">>> Motor control cluster >>>"
            # ">>> yStepper command>>>"
            # ">> Manual override >>"
            n399 = Dequeue Element(queue=w1085, timeout in ms (-1)=w1084, error in (no error)=w1086) -> (element=w1083:T10)  [unwired: 3 out]
            n400 = Equal?(x=w1082, y=u8 1) -> (x = y?=w1080:bool)
            n401 = case shown="\"None\", Default" w1083 {
              tunnel: [w1096 State_Type_Definitions,_for_0.26g_versions_and_later_2."True Stop" ("Enum")] -> w1087
              tunnel: [w1099 w1116] -> w1088
              tunnel: [State_Type_Definitions,_for_0.26g_versions_and_later_2."Idle" ("Enum") State_Type_Definitions,_for_0.26g_versions_and_later_2."Shutdown" ("Enum")] -> w1089
              tunnel: w1080 -> [w1095 _]
              tunnel: w1079 -> [w1094 _]
              tunnel: w1078 -> [w1090 w1113]
              frame "None", Default {
                # "Stays in Task 5F until stepper reaches desired \nheight"
                # "T: Go back to idle, F: Continue with task\""
                # ">> Manual override >>"
                n402 = case shown="True" w1095 {
                  tunnel: [w1103 w1109] -> w1099
                  tunnel: w1090 -> [w1101 w1107]
                  frame False {
                    n403 = for {
                      tunnel: string[] ["Z STEPPER GRAB HEIGHT", "READ STEPPER VALUES"] ("element") -> [w1104] mode=indexing
                      shift-right: [w1106] -> w1103
                      shift-left: w1101 -> [w1105]
                      n404 = Enqueue Element(queue=w1105, element=w1104) -> (queue out=w1106:refnum<queue>)  [unwired: 2 in, 2 out]
                    }
                  }
                  frame True {
                    n405 = for {
                      shift-right: [w1111] -> w1109
                      shift-left: w1107 -> [w1112]
                      tunnel: string[] ["SET TIMER 5", "CLOSE CLAW", ""] -> [w1110] mode=indexing
                      n406 = Enqueue Element(queue=w1112, element=w1110) -> (queue out=w1111:refnum<queue>)  [unwired: 2 in, 2 out]
                    }
                  }
                }
                n407 = Or(x=w1095, y=w1094) -> (x .or. y?=w1097:bool)
                n408 = Select(t=State_Type_Definitions,_for_0.26g_versions_and_later_2."True Stop" ("Enum"), s=w1094, f=State_Type_Definitions,_for_0.26g_versions_and_later_2."Task 5G: CLOSE CLAW" ("Enum")) -> (s? t:f=w1091:T9)
                n409 = Select(t=w1091, s=w1097, f=State_Type_Definitions,_for_0.26g_versions_and_later_2."Task 5F: ARM GRAB HEIGHT" ("Enum")) -> (s? t:f=w1096:T9)
              }
              frame "Exit" {
                n410 = for {
                  shift-right: [w1119] -> w1116
                  shift-left: w1113 -> [w1120]
                  tunnel: string[] ["STOP", "RESET ENCODERS", "RESET YAW", "ARDUINO MODE 0"] -> [w1118] mode=indexing
                  n411 = Enqueue Element(queue=w1120, element=w1118) -> (queue out=w1119:refnum<queue>)  [unwired: 2 in, 2 out]
                }
              }
            }
          }
          frame 22 {
            # ">>> yStepper command>>>"
            # ">> Manual override >>"
            n412 = Dequeue Element(queue=w1130, timeout in ms (-1)=w1129, error in (no error)=w1128) -> (element=w1127:T10)  [unwired: 3 out]
            n413 = case shown="\"None\", Default" w1127 {
              tunnel: [w1139 State_Type_Definitions,_for_0.26g_versions_and_later_2."True Stop" ("Enum")] -> w1132
              tunnel: [w1142 w1159] -> w1125
              tunnel: [State_Type_Definitions,_for_0.26g_versions_and_later_2."Idle" ("Enum") State_Type_Definitions,_for_0.26g_versions_and_later_2."Shutdown" ("Enum")] -> w1124
              tunnel: w1126 -> [w1133 _]
              tunnel: w1131 -> [w1138 w1156]
              tunnel: w1122 -> [w1137 _]
              frame "None", Default {
                # ">> Is time up? >>"
                # "Determines if object is in range to pick up"
                # ">> Manual override >>"
                n414 = case shown="True" w1137 {
                  tunnel: [w1146 w1152] -> w1142
                  tunnel: w1138 -> [w1144 w1150]
                  frame False {
                    n415 = for {
                      tunnel: string[] ["CLOSE CLAW", "START TIMER"] ("element") -> [w1147] mode=indexing
                      shift-right: [w1149] -> w1146
                      shift-left: w1144 -> [w1148]
                      n416 = Enqueue Element(queue=w1148, element=w1147) -> (queue out=w1149:refnum<queue>)  [unwired: 2 in, 2 out]
                    }
                  }
                  frame True {
                    n417 = for {
                      shift-right: [w1154] -> w1152
                      shift-left: w1150 -> [w1155]
                      tunnel: string[] ["READ STEPPER VALUES", "", ""] -> [w1153] mode=indexing
                      n418 = Enqueue Element(queue=w1155, element=w1153) -> (queue out=w1154:refnum<queue>)  [unwired: 2 in, 2 out]
                    }
                  }
                }
                n419 = Or(x=w1137, y=w1133) -> (x .or. y?=w1140:bool)
                n420 = Select(t=State_Type_Definitions,_for_0.26g_versions_and_later_2."True Stop" ("Enum"), s=w1133, f=State_Type_Definitions,_for_0.26g_versions_and_later_2."Task 5H: RAISE ARM" ("Enum")) -> (s? t:f=w1135:T9)
                n421 = Select(t=w1135, s=w1140, f=State_Type_Definitions,_for_0.26g_versions_and_later_2."Task 5G: CLOSE CLAW" ("Enum")) -> (s? t:f=w1139:T9)
              }
              frame "Exit" {
                n422 = for {
                  shift-right: [w1162] -> w1159
                  shift-left: w1156 -> [w1163]
                  tunnel: string[] ["STOP", "RESET ENCODERS", "RESET YAW", "ARDUINO MODE 0"] -> [w1161] mode=indexing
                  n423 = Enqueue Element(queue=w1163, element=w1161) -> (queue out=w1162:refnum<queue>)  [unwired: 2 in, 2 out]
                }
              }
            }
          }
          frame 23 {
            # ">>> yStepper command>>>"
            # ">> Manual override >>"
            n424 = Dequeue Element(queue=w1173, timeout in ms (-1)=w1172, error in (no error)=w1174) -> (element=w1171:T10)  [unwired: 3 out]
            n425 = Equal?(x=w1170, y=u8 60) -> (x = y?=w1168:bool)
            n426 = case shown="\"None\", Default" w1171 {
              tunnel: [w1184 State_Type_Definitions,_for_0.26g_versions_and_later_2."True Stop" ("Enum")] -> w1175
              tunnel: [w1187 w1204] -> w1176
              tunnel: [State_Type_Definitions,_for_0.26g_versions_and_later_2."Idle" ("Enum") State_Type_Definitions,_for_0.26g_versions_and_later_2."Shutdown" ("Enum")] -> w1177
              tunnel: w1168 -> [w1183 _]
              tunnel: w1167 -> [w1182 _]
              tunnel: w1166 -> [w1178 w1201]
              frame "None", Default {
                # "Stays in Task 5_A until stepper reaches desired \nheight"
                # "T: Go back to idle, F: Continue with task\""
                # ">> Manual override >>"
                n427 = case shown="False" w1183 {
                  tunnel: [w1191 w1197] -> w1187
                  tunnel: w1178 -> [w1189 w1195]
                  frame False {
                    n428 = for {
                      tunnel: string[] ["Z STEPPER CAM HEIGHT", "READ STEPPER VALUES"] ("element") -> [w1192] mode=indexing
                      shift-right: [w1194] -> w1191
                      shift-left: w1189 -> [w1193]
                      n429 = Enqueue Element(queue=w1193, element=w1192) -> (queue out=w1194:refnum<queue>)  [unwired: 2 in, 2 out]
                    }
                  }
                  frame True {
                    n430 = for {
                      shift-right: [w1199] -> w1197
                      shift-left: w1195 -> [w1200]
                      tunnel: string[] ["ARDUINO - ULTRASONIC", "READ ULTRASONIC", ""] -> [w1198] mode=indexing
                      n431 = Enqueue Element(queue=w1200, element=w1198) -> (queue out=w1199:refnum<queue>)  [unwired: 2 in, 2 out]
                    }
                  }
                }
                n432 = Or(x=w1183, y=w1182) -> (x .or. y?=w1185:bool)
                n433 = Select(t=State_Type_Definitions,_for_0.26g_versions_and_later_2."True Stop" ("Enum"), s=w1182, f=State_Type_Definitions,_for_0.26g_versions_and_later_2."True Stop" ("Enum")) -> (s? t:f=w1179:T9)
                n434 = Select(t=w1179, s=w1185, f=State_Type_Definitions,_for_0.26g_versions_and_later_2."Task 5H: RAISE ARM" ("Enum")) -> (s? t:f=w1184:T9)
              }
              frame "Exit" {
                n435 = for {
                  shift-right: [w1207] -> w1204
                  shift-left: w1201 -> [w1208]
                  tunnel: string[] ["STOP", "RESET ENCODERS", "RESET YAW", "ARDUINO MODE 0"] -> [w1206] mode=indexing
                  n436 = Enqueue Element(queue=w1208, element=w1206) -> (queue out=w1207:refnum<queue>)  [unwired: 2 in, 2 out]
                }
              }
            }
          }
          frame 24 {
            # ">>> yStepper command>>>"
            n437 = Dequeue Element(queue=w1217, timeout in ms (-1)=w1216, error in (no error)=w1215) -> (element=w1222:T10)  [unwired: 3 out]
            n438 = Equal?(x=w1213, y=u8 60) -> (x = y?=w1212:bool)
            n439 = case shown="\"None\", Default" w1222 {
              tunnel: [w1229 State_Type_Definitions,_for_0.26g_versions_and_later_2."True Stop" ("Enum")] -> w1220
              tunnel: [w1228 w1246] -> w1219
              tunnel: [State_Type_Definitions,_for_0.26g_versions_and_later_2."Idle" ("Enum") State_Type_Definitions,_for_0.26g_versions_and_later_2."Shutdown" ("Enum")] -> w1221
              tunnel: w1218 -> [w1224 _]
              tunnel: w1214 -> [w1226 _]
              tunnel: w1212 -> [w1223 _]
              frame "None", Default {
                n440 = case shown="False" w1223 {
                  tunnel: [w1234 w1240] -> w1228
                  tunnel: w1226 -> [w1232 w1238]
                  frame False {
                    n441 = for {
                      tunnel: string[] ["Z STEPPER CAM HEIGHT", "READ STEPPER VALUES"] ("element") -> [w1235] mode=indexing
                      shift-right: [w1237] -> w1234
                      shift-left: w1232 -> [w1236]
                      n442 = Enqueue Element(queue=w1236, element=w1235) -> (queue out=w1237:refnum<queue>)  [unwired: 2 in, 2 out]
                    }
                  }
                  frame True {
                    n443 = for {
                      shift-right: [w1242] -> w1240
                      shift-left: w1238 -> [w1243]
                      tunnel: string[] ["CAM ACQ", "OPEN LOG CAM"] -> [w1241] mode=indexing
                      n444 = Enqueue Element(queue=w1243, element=w1241) -> (queue out=w1242:refnum<queue>)  [unwired: 2 in, 2 out]
                    }
                  }
                }
                n445 = Or(x=w1223, y=w1224) -> (x .or. y?=w1225:bool)
                n446 = Select(t=State_Type_Definitions,_for_0.26g_versions_and_later_2."Task 6_B" ("Enum"), s=w1225, f=State_Type_Definitions,_for_0.26g_versions_and_later_2."Task 6_A" ("Enum")) -> (s? t:f=w1229:T9)
              }
              frame "Exit" {
                n447 = for {
                  shift-right: [w1249] -> w1246
                  shift-left: _ -> [w1250]
                  tunnel: string[] ["STOP", "RESET ENCODERS", "RESET YAW", "ARDUINO MODE 0"] -> [w1248] mode=indexing
                  n448 = Enqueue Element(queue=w1250, element=w1248) -> (queue out=w1249:refnum<queue>)  [unwired: 2 in, 2 out]
                }
              }
            }
          }
          frame 25 {
            # ">>> yStepper command>>>"
            n449 = Dequeue Element(queue=w1261, timeout in ms (-1)=w1259, error in (no error)=w1260) -> (element=w1258:T10)  [unwired: 3 out]
            n450 = case shown="\"None\", Default" w1258 {
              tunnel: [w1268 State_Type_Definitions,_for_0.26g_versions_and_later_2."True Stop" ("Enum")] -> w1254
              tunnel: [w1267 w1286] -> w1262
              tunnel: [State_Type_Definitions,_for_0.26g_versions_and_later_2."Idle" ("Enum") State_Type_Definitions,_for_0.26g_versions_and_later_2."Shutdown" ("Enum")] -> w1255
              tunnel: w1257 -> [w1263 _]
              tunnel: w1256 -> [w1265 _]
              tunnel: w1253 -> [w1264 w1283]
              frame "None", Default {
                # ">> Manual override >>"
                n451 = case shown="True" w1265 {
                  tunnel: [w1273 w1279] -> w1267
                  tunnel: w1264 -> [w1272 w1277]
                  frame False {
                    n452 = for {
                      shift-right: [w1276] -> w1273
                      shift-left: w1272 -> [w1275]
                      tunnel: string[] ["CAM ACQ", "PROCESS IMAGE", "OPEN CLAW"] -> [w1274] mode=indexing
                      n453 = Enqueue Element(queue=w1275, element=w1274) -> (queue out=w1276:refnum<queue>)  [unwired: 2 in, 2 out]
                    }
                  }
                  frame True {
                    n454 = for {
                      shift-right: [w1281] -> w1279
                      shift-left: w1277 -> [w1282]
                      tunnel: string[] ["CAM ACQ", "PROCESS IMAGE", "CLOSE CLAW"] -> [w1280] mode=indexing
                      n455 = Enqueue Element(queue=w1282, element=w1280) -> (queue out=w1281:refnum<queue>)  [unwired: 2 in, 2 out]
                    }
                  }
                }
                n456 = Select(t=State_Type_Definitions,_for_0.26g_versions_and_later_2."True Stop" ("Enum"), s=w1263, f=State_Type_Definitions,_for_0.26g_versions_and_later_2."Task 6_B" ("Enum")) -> (s? t:f=w1268:T9)
              }
              frame "Exit" {
                # ">> State after true stop >>"
                # ">> Goes to true stop >>"
                n457 = for {
                  shift-right: [w1289] -> w1286
                  shift-left: w1283 -> [w1290]
                  tunnel: string[] ["STOP", "RESET ENCODERS", "RESET YAW", ""] -> [w1288] mode=indexing
                  n458 = Enqueue Element(queue=w1290, element=w1288) -> (queue out=w1289:refnum<queue>)  [unwired: 2 in, 2 out]
                }
              }
            }
          }
          frame 26 {
          }
          frame 27 {
            # ">>> Motor control cluster >>>"
            # ">>> yStepper command>>>"
            # ">> Manual override >>"
            n459 = Dequeue Element(queue=w1305, timeout in ms (-1)=w1304, error in (no error)=w1306) -> (element=w1303:T10)  [unwired: 3 out]
            n460 = Equal?(x=w1302, y=u8 60) -> (x = y?=w1300:bool)
            n461 = case shown="\"None\", Default" w1303 {
              tunnel: [w1316 State_Type_Definitions,_for_0.26g_versions_and_later_2."True Stop" ("Enum")] -> w1307
              tunnel: [w1319 w1336] -> w1308
              tunnel: [State_Type_Definitions,_for_0.26g_versions_and_later_2."Idle" ("Enum") State_Type_Definitions,_for_0.26g_versions_and_later_2."Shutdown" ("Enum")] -> w1309
              tunnel: w1300 -> [w1315 _]
              tunnel: w1299 -> [w1314 _]
              tunnel: w1298 -> [w1310 w1333]
              frame "None", Default {
                # "Stays in Task 5_A until stepper reaches desired \nheight"
                # "T: Go back to idle, F: Continue with task\""
                # ">> Manual override >>"
                n462 = case shown="True" w1315 {
                  tunnel: [w1323 w1329] -> w1319
                  tunnel: w1310 -> [w1321 w1327]
                  frame False {
                    n463 = for {
                      tunnel: string[] ["Z STEPPER CAM HEIGHT", "READ STEPPER VALUES"] ("element") -> [w1324] mode=indexing
                      shift-right: [w1326] -> w1323
                      shift-left: w1321 -> [w1325]
                      n464 = Enqueue Element(queue=w1325, element=w1324) -> (queue out=w1326:refnum<queue>)  [unwired: 2 in, 2 out]
                    }
                  }
                  frame True {
                    n465 = for {
                      shift-right: [w1331] -> w1329
                      shift-left: w1327 -> [w1332]
                      tunnel: string[] ["ARDUINO - ULTRASONIC", "READ ULTRASONIC", ""] -> [w1330] mode=indexing
                      n466 = Enqueue Element(queue=w1332, element=w1330) -> (queue out=w1331:refnum<queue>)  [unwired: 2 in, 2 out]
                    }
                  }
                }
                n467 = Or(x=w1315, y=w1314) -> (x .or. y?=w1317:bool)
                n468 = Select(t=State_Type_Definitions,_for_0.26g_versions_and_later_2."True Stop" ("Enum"), s=w1314, f=State_Type_Definitions,_for_0.26g_versions_and_later_2."Task 8B: MOVE TO BOX" ("Enum")) -> (s? t:f=w1311:T9)
                n469 = Select(t=w1311, s=w1317, f=State_Type_Definitions,_for_0.26g_versions_and_later_2."Task 8A: RAISE ARM" ("Enum")) -> (s? t:f=w1316:T9)
              }
              frame "Exit" {
                n470 = for {
                  shift-right: [w1339] -> w1336
                  shift-left: w1333 -> [w1340]
                  tunnel: string[] ["STOP", "RESET ENCODERS", "RESET YAW", "ARDUINO MODE 0"] -> [w1338] mode=indexing
                  n471 = Enqueue Element(queue=w1340, element=w1338) -> (queue out=w1339:refnum<queue>)  [unwired: 2 in, 2 out]
                }
              }
            }
          }
          frame 28 {
            w1347 = u8 15 ("y")
            # ">>> yStepper command>>>"
            n472 = Less?(x=w1344, y=w1347) -> (x < y?=w1345:bool)
            n473 = Dequeue Element(queue=w1351, timeout in ms (-1)=w1350, error in (no error)=w1352) -> (element=w1349:T10)  [unwired: 3 out]
            n474 = Less?(x=w1343, y=w1347) -> (x < y?=w1346:bool)
            n475 = And(x=w1346, y=w1345) -> (x .and. y?=w1342:bool)
            n476 = case shown="\"None\", Default" w1349 {
              tunnel: [w1364 State_Type_Definitions,_for_0.26g_versions_and_later_2."True Stop" ("Enum")] -> w1354
              tunnel: [w1367 w1384] -> w1353
              tunnel: [State_Type_Definitions,_for_0.26g_versions_and_later_2."Idle" ("Enum") State_Type_Definitions,_for_0.26g_versions_and_later_2."Shutdown" ("Enum")] -> w1355
              tunnel: w1357 -> [w1363 _]
              tunnel: w1356 -> [w1359 w1381]
              tunnel: w1342 -> [w1358 _]
              frame "None", Default {
                # "Stays in Task 5_B to capture image over 5 seconds"
                # "T: Go back to idle, F: Continue with task\""
                # ">> Manual override >>"
                n477 = case shown="False" w1358 {
                  tunnel: [w1371 w1377] -> w1367
                  tunnel: w1359 -> [w1369 w1375]
                  frame False {
                    n478 = for {
                      tunnel: string[] ["FORWARD", "READ ULTRASONIC", "READ NAVX"] ("element") -> [w1372] mode=indexing
                      shift-right: [w1374] -> w1371
                      shift-left: w1369 -> [w1373]
                      n479 = Enqueue Element(queue=w1373, element=w1372) -> (queue out=w1374:refnum<queue>)  [unwired: 2 in, 2 out]
                    }
                  }
                  frame True {
                    n480 = for {
                      shift-right: [w1379] -> w1377
                      shift-left: w1375 -> [w1380]
                      tunnel: string[] ["STOP", "RESET ENCODERS", "OPEN LOG CAM", "SET TIMER 2", "OPEN IMAQ REF"] -> [w1378] mode=indexing
                      n481 = Enqueue Element(queue=w1380, element=w1378) -> (queue out=w1379:refnum<queue>)  [unwired: 2 in, 2 out]
                    }
                  }
                }
                n482 = Or(x=w1358, y=w1363) -> (x .or. y?=w1365:bool)
                n483 = Select(t=State_Type_Definitions,_for_0.26g_versions_and_later_2."True Stop" ("Enum"), s=w1363, f=State_Type_Definitions,_for_0.26g_versions_and_later_2."Task 8C: CAM BURST" ("Enum")) -> (s? t:f=w1360:T9)
                n484 = Select(t=w1360, s=w1365, f=State_Type_Definitions,_for_0.26g_versions_and_later_2."Task 8B: MOVE TO BOX" ("Enum")) -> (s? t:f=w1364:T9)
              }
              frame "Exit" {
                n485 = for {
                  shift-right: [w1387] -> w1384
                  shift-left: w1381 -> [w1388]
                  tunnel: string[] ["STOP", "RESET ENCODERS", "RESET YAW", "ARDUINO MODE 0"] -> [w1386] mode=indexing
                  n486 = Enqueue Element(queue=w1388, element=w1386) -> (queue out=w1387:refnum<queue>)  [unwired: 2 in, 2 out]
                }
              }
            }
          }
          frame 29 {
            # ">>> Motor control cluster >>>"
            # ">>> yStepper command>>>"
            # ">> Manual override >>"
            n487 = Dequeue Element(queue=w1398, timeout in ms (-1)=w1397, error in (no error)=w1396) -> (element=w1395:T10)  [unwired: 3 out]
            n488 = case shown="\"None\", Default" w1395 {
              tunnel: [w1407 State_Type_Definitions,_for_0.26g_versions_and_later_2."True Stop" ("Enum")] -> w1400
              tunnel: [w1410 w1427] -> w1393
              tunnel: [State_Type_Definitions,_for_0.26g_versions_and_later_2."Idle" ("Enum") State_Type_Definitions,_for_0.26g_versions_and_later_2."Shutdown" ("Enum")] -> w1392
              tunnel: w1394 -> [w1401 _]
              tunnel: w1399 -> [w1406 w1424]
              tunnel: w1390 -> [w1405 _]
              frame "None", Default {
                # ">> Is time up? >>"
                # "Determines if object is in range to pick up"
                # ">> Manual override >>"
                n489 = case shown="True" w1405 {
                  tunnel: [w1414 w1420] -> w1410
                  tunnel: w1406 -> [w1412 w1418]
                  frame False {
                    n490 = for {
                      tunnel: string[] ["CAM ACQ", "START TIMER"] ("element") -> [w1415] mode=indexing
                      shift-right: [w1417] -> w1414
                      shift-left: w1412 -> [w1416]
                      n491 = Enqueue Element(queue=w1416, element=w1415) -> (queue out=w1417:refnum<queue>)  [unwired: 2 in, 2 out]
                    }
                  }
                  frame True {
                    n492 = for {
                      shift-right: [w1422] -> w1420
                      shift-left: w1418 -> [w1423]
                      tunnel: string[] ["CAM CLOSE", "PROCESS IMAGE", "SET TIMER 5"] -> [w1421] mode=indexing
                      n493 = Enqueue Element(queue=w1423, element=w1421) -> (queue out=w1422:refnum<queue>)  [unwired: 2 in, 2 out]
                    }
                  }
                }
                n494 = Or(x=w1405, y=w1401) -> (x .or. y?=w1408:bool)
                n495 = Select(t=State_Type_Definitions,_for_0.26g_versions_and_later_2."True Stop" ("Enum"), s=w1401, f=State_Type_Definitions,_for_0.26g_versions_and_later_2."Task 8D: PROCESS IMAGE" ("Enum")) -> (s? t:f=w1403:T9)
                n496 = Select(t=w1403, s=w1408, f=State_Type_Definitions,_for_0.26g_versions_and_later_2."Task 8C: CAM BURST" ("Enum")) -> (s? t:f=w1407:T9)
              }
              frame "Exit" {
                n497 = for {
                  shift-right: [w1430] -> w1427
                  shift-left: w1424 -> [w1431]
                  tunnel: string[] ["STOP", "RESET ENCODERS", "RESET YAW", "ARDUINO MODE 0"] -> [w1429] mode=indexing
                  n498 = Enqueue Element(queue=w1431, element=w1429) -> (queue out=w1430:refnum<queue>)  [unwired: 2 in, 2 out]
                }
              }
            }
          }
          frame 30 {
            # ">>> yStepper command>>>"
            n499 = Dequeue Element(queue=w1438, timeout in ms (-1)=w1437, error in (no error)=w1436) -> (element=w1435:T10)  [unwired: 3 out]
            n500 = case shown="\"None\", Default" w1435 {
              tunnel: [w1450 State_Type_Definitions,_for_0.26g_versions_and_later_2."True Stop" ("Enum")] -> w1442
              tunnel: [w1453 w1470] -> w1441
              tunnel: [State_Type_Definitions,_for_0.26g_versions_and_later_2."Idle" ("Enum") State_Type_Definitions,_for_0.26g_versions_and_later_2."Shutdown" ("Enum")] -> w1443
              tunnel: w1439 -> [w1449 _]
              tunnel: w1440 -> [w1445 w1467]
              tunnel: w1433 -> [w1444 _]
              frame "None", Default {
                # ">> T: Breaks out of state loop; F: Stays in loop>>"
                # ">> Manual override >>"
                # ">> Checks if time is up>>"
                # "Stays in Task 5D until the object is detected"
                # "T: Go back to idle, F: Continue with task\""
                # ">> Manual override >>"
                n501 = case shown="False" w1444 {
                  tunnel: [w1457 w1463] -> w1453
                  tunnel: w1445 -> [w1455 w1461]
                  frame False {
                    n502 = for {
                      tunnel: string[] ["START TIMER", "PROCESS IMAGE", ""] ("element") -> [w1458] mode=indexing
                      shift-right: [w1460] -> w1457
                      shift-left: w1455 -> [w1459]
                      n503 = Enqueue Element(queue=w1459, element=w1458) -> (queue out=w1460:refnum<queue>)  [unwired: 2 in, 2 out]
                    }
                  }
                  frame True {
                    n504 = for {
                      shift-right: [w1465] -> w1463
                      shift-left: w1461 -> [w1466]
                      tunnel: string[] ["RESET ENCODERS", "", ""] -> [w1464] mode=indexing
                      n505 = Enqueue Element(queue=w1466, element=w1464) -> (queue out=w1465:refnum<queue>)  [unwired: 2 in, 2 out]
                    }
                  }
                }
                n506 = Or(x=w1444, y=w1449) -> (x .or. y?=w1451:bool)
                n507 = Select(t=State_Type_Definitions,_for_0.26g_versions_and_later_2."True Stop" ("Enum"), s=w1449, f=State_Type_Definitions,_for_0.26g_versions_and_later_2."Task 8E: ROBOT ADJUST" ("Enum")) -> (s? t:f=w1446:T9)
                n508 = Select(t=w1446, s=w1451, f=State_Type_Definitions,_for_0.26g_versions_and_later_2."Task 8D: PROCESS IMAGE" ("Enum")) -> (s? t:f=w1450:T9)
              }
              frame "Exit" {
                n509 = for {
                  shift-right: [w1473] -> w1470
                  shift-left: w1467 -> [w1474]
                  tunnel: string[] ["STOP", "RESET ENCODERS", "RESET YAW", "ARDUINO MODE 0"] -> [w1472] mode=indexing
                  n510 = Enqueue Element(queue=w1474, element=w1472) -> (queue out=w1473:refnum<queue>)  [unwired: 2 in, 2 out]
                }
              }
            }
          }
          frame 31 {
            # ">>> Motor control cluster >>>"
            # ">>> yStepper command>>>"
            n511 = Dequeue Element(queue=w1490, timeout in ms (-1)=w1489, error in (no error)=w1488) -> (element=w1487:T10)  [unwired: 3 out]
            n512 = Subtract(x=w1485, y=300.0) -> (x-y=w1483:dbl)
            "x-y" <- w1483
            n513 = formula code="if (error <= -61&&error > -300){\ndistance = -15;\nxSpeed = -30;\n}\n\nelse if (error <= -26 && error >= -60){\ndistance = -10;\nxSpeed = -30;\n}\n\nelse if (error >= -25 && error <= 25){\ndistance = 0;\nxSpeed = 0;\n}\n\nelse if (error >= 51 && error <= 80){\ndistance = 10;\nxSpeed = 30;\n}\n\nelse if (error >= 81 && error <= 100){\ndistance = 15;\nxSpeed = 30;\n}\n\nelse if (error >= 101 && error <= 120){\ndistance = 20;\nxSpeed = 30;\n}\n\nelse if (error >= 121 && error < 300){\ndistance = 25;\nxSpeed = 30;\n}\n\nelse{\ndistance = 0;\nxSpeed = 0;\n}"("error"=w1483) -> ("distance"=w1478:dbl, "xSpeed"=w1480:dbl)
            n514 = formula code="if (target > 0){\nif (current  >= target)\noutput = 1;\n}\n\nelse if (target == 0){\nif (current == target)\noutput = 1;\n}\n\nelse if (target < 0){\nif (current <= target)\noutput = 1;\n}\n\nelse\noutput = 0;"("target"=w1478, "current"=w1479) -> ("output"=w1477:dbl)
            n515 = Bundle By Name(cluster=w1482, "xSpeed"=w1480) -> (w1481:T12)
            n516 = Equal?(x=w1477, y=1.0) -> (x = y?=w1475:bool)
            n517 = case shown="\"None\", Default" w1487 {
              tunnel: [w1502 State_Type_Definitions,_for_0.26g_versions_and_later_2."True Stop" ("Enum")] -> w1494
              tunnel: [w1505 w1522] -> w1493
              tunnel: [State_Type_Definitions,_for_0.26g_versions_and_later_2."Idle" ("Enum") State_Type_Definitions,_for_0.26g_versions_and_later_2."Shutdown" ("Enum")] -> w1495
              tunnel: w1491 -> [w1501 _]
              tunnel: w1492 -> [w1497 w1519]
              tunnel: w1475 -> [w1496 _]
              frame "None", Default {
                # ">> T: Breaks out of state loop; F: Stays in loop>>"
                # ">> Manual override >>"
                # ">> Checks if time is up>>"
                # "Stays in Task 5D until the object is detected"
                # "T: Go back to idle, F: Continue with task\""
                # ">> Manual override >>"
                n518 = case shown="False" w1496 {
                  tunnel: [w1509 w1515] -> w1505
                  tunnel: w1497 -> [w1507 w1513]
                  frame False {
                    n519 = for {
                      tunnel: string[] ["X AXIS - SLOW", "READ ENCODERS", "READ NAVX"] ("element") -> [w1510] mode=indexing
                      shift-right: [w1512] -> w1509
                      shift-left: w1507 -> [w1511]
                      n520 = Enqueue Element(queue=w1511, element=w1510) -> (queue out=w1512:refnum<queue>)  [unwired: 2 in, 2 out]
                    }
                  }
                  frame True {
                    n521 = for {
                      shift-right: [w1517] -> w1515
                      shift-left: w1513 -> [w1518]
                      tunnel: string[] ["SET TIMER 2", "STOP", "READ STEPPER VALUES", ""] -> [w1516] mode=indexing
                      n522 = Enqueue Element(queue=w1518, element=w1516) -> (queue out=w1517:refnum<queue>)  [unwired: 2 in, 2 out]
                    }
                  }
                }
                n523 = Or(x=w1496, y=w1501) -> (x .or. y?=w1503:bool)
                n524 = Select(t=State_Type_Definitions,_for_0.26g_versions_and_later_2."True Stop" ("Enum"), s=w1501, f=State_Type_Definitions,_for_0.26g_versions_and_later_2."Task 8H: ARM ADJUST" ("Enum")) -> (s? t:f=w1498:T9)
                n525 = Select(t=w1498, s=w1503, f=State_Type_Definitions,_for_0.26g_versions_and_later_2."Task 8E: ROBOT ADJUST" ("Enum")) -> (s? t:f=w1502:T9)
              }
              frame "Exit" {
                n526 = for {
                  shift-right: [w1525] -> w1522
                  shift-left: w1519 -> [w1526]
                  tunnel: string[] ["STOP", "RESET ENCODERS", "RESET YAW", "ARDUINO MODE 0"] -> [w1524] mode=indexing
                  n527 = Enqueue Element(queue=w1526, element=w1524) -> (queue out=w1525:refnum<queue>)  [unwired: 2 in, 2 out]
                }
              }
            }
          }
          frame 32 {
            # ">>> Motor control cluster >>>"
            # ">>> yStepper command>>>"
            # ">> Manual override >>"
            n528 = Dequeue Element(queue=w1536, timeout in ms (-1)=w1535, error in (no error)=w1534) -> (element=w1533:T10)  [unwired: 3 out]
            n529 = case shown="\"None\", Default" w1533 {
              tunnel: [w1545 State_Type_Definitions,_for_0.26g_versions_and_later_2."True Stop" ("Enum")] -> w1538
              tunnel: [w1548 w1565] -> w1531
              tunnel: [State_Type_Definitions,_for_0.26g_versions_and_later_2."Idle" ("Enum") State_Type_Definitions,_for_0.26g_versions_and_later_2."Shutdown" ("Enum")] -> w1530
              tunnel: w1532 -> [w1539 _]
              tunnel: w1537 -> [w1544 w1562]
              tunnel: w1528 -> [w1543 _]
              frame "None", Default {
                # ">> Is time up? >>"
                # "Determines if object is in range to pick up"
                # ">> Manual override >>"
                n530 = case shown="True" w1543 {
                  tunnel: [w1552 w1558] -> w1548
                  tunnel: w1544 -> [w1550 w1556]
                  frame False {
                    n531 = for {
                      tunnel: string[] ["CAM ACQ", "START TIMER"] ("element") -> [w1553] mode=indexing
                      shift-right: [w1555] -> w1552
                      shift-left: w1550 -> [w1554]
                      n532 = Enqueue Element(queue=w1554, element=w1553) -> (queue out=w1555:refnum<queue>)  [unwired: 2 in, 2 out]
                    }
                  }
                  frame True {
                    n533 = for {
                      shift-right: [w1560] -> w1558
                      shift-left: w1556 -> [w1561]
                      tunnel: string[] ["CAM CLOSE", "PROCESS IMAGE", "SET TIMER 3"] -> [w1559] mode=indexing
                      n534 = Enqueue Element(queue=w1561, element=w1559) -> (queue out=w1560:refnum<queue>)  [unwired: 2 in, 2 out]
                    }
                  }
                }
                n535 = Or(x=w1543, y=w1539) -> (x .or. y?=w1546:bool)
                n536 = Select(t=State_Type_Definitions,_for_0.26g_versions_and_later_2."True Stop" ("Enum"), s=w1539, f=State_Type_Definitions,_for_0.26g_versions_and_later_2."Task 8G: PROCESS IMAGE 2" ("Enum")) -> (s? t:f=w1541:T9)
                n537 = Select(t=w1541, s=w1546, f=State_Type_Definitions,_for_0.26g_versions_and_later_2."Task 8F: CAM BURST 2" ("Enum")) -> (s? t:f=w1545:T9)
              }
              frame "Exit" {
                n538 = for {
                  shift-right: [w1568] -> w1565
                  shift-left: w1562 -> [w1569]
                  tunnel: string[] ["STOP", "RESET ENCODERS", "RESET YAW", "ARDUINO MODE 0"] -> [w1567] mode=indexing
                  n539 = Enqueue Element(queue=w1569, element=w1567) -> (queue out=w1568:refnum<queue>)  [unwired: 2 in, 2 out]
                }
              }
            }
          }
          frame 33 {
            # ">>> yStepper command>>>"
            n540 = Dequeue Element(queue=w1576, timeout in ms (-1)=w1575, error in (no error)=w1574) -> (element=w1573:T10)  [unwired: 3 out]
            n541 = case shown="\"None\", Default" w1573 {
              tunnel: [w1588 State_Type_Definitions,_for_0.26g_versions_and_later_2."True Stop" ("Enum")] -> w1580
              tunnel: [w1591 w1608] -> w1579
              tunnel: [State_Type_Definitions,_for_0.26g_versions_and_later_2."Idle" ("Enum") State_Type_Definitions,_for_0.26g_versions_and_later_2."Shutdown" ("Enum")] -> w1581
              tunnel: w1577 -> [w1587 _]
              tunnel: w1578 -> [w1583 w1605]
              tunnel: w1571 -> [w1582 _]
              frame "None", Default {
                # ">> T: Breaks out of state loop; F: Stays in loop>>"
                # ">> Manual override >>"
                # ">> Checks if time is up>>"
                # "Stays in Task 5D until the object is detected"
                # "T: Go back to idle, F: Continue with task\""
                # ">> Manual override >>"
                n542 = case shown="False" w1582 {
                  tunnel: [w1595 w1601] -> w1591
                  tunnel: w1583 -> [w1593 w1599]
                  frame False {
                    n543 = for {
                      tunnel: string[] ["START TIMER", "PROCESS IMAGE", ""] ("element") -> [w1596] mode=indexing
                      shift-right: [w1598] -> w1595
                      shift-left: w1593 -> [w1597]
                      n544 = Enqueue Element(queue=w1597, element=w1596) -> (queue out=w1598:refnum<queue>)  [unwired: 2 in, 2 out]
                    }
                  }
                  frame True {
                    n545 = for {
                      shift-right: [w1603] -> w1601
                      shift-left: w1599 -> [w1604]
                      tunnel: string[] ["READ STEPPER VALUES", "Y STEPPER CONTROL", ""] -> [w1602] mode=indexing
                      n546 = Enqueue Element(queue=w1604, element=w1602) -> (queue out=w1603:refnum<queue>)  [unwired: 2 in, 2 out]
                    }
                  }
                }
                n547 = Or(x=w1582, y=w1587) -> (x .or. y?=w1589:bool)
                n548 = Select(t=State_Type_Definitions,_for_0.26g_versions_and_later_2."True Stop" ("Enum"), s=w1587, f=State_Type_Definitions,_for_0.26g_versions_and_later_2."Task 8H: ARM ADJUST" ("Enum")) -> (s? t:f=w1584:T9)
                n549 = Select(t=w1584, s=w1589, f=State_Type_Definitions,_for_0.26g_versions_and_later_2."Task 8G: PROCESS IMAGE 2" ("Enum")) -> (s? t:f=w1588:T9)
              }
              frame "Exit" {
                n550 = for {
                  shift-right: [w1611] -> w1608
                  shift-left: w1605 -> [w1612]
                  tunnel: string[] ["STOP", "RESET ENCODERS", "RESET YAW", "ARDUINO MODE 0"] -> [w1610] mode=indexing
                  n551 = Enqueue Element(queue=w1612, element=w1610) -> (queue out=w1611:refnum<queue>)  [unwired: 2 in, 2 out]
                }
              }
            }
          }
          frame 34 {
            # ">>> yStepper command>>>"
            n552 = Dequeue Element(queue=w1625, timeout in ms (-1)=w1626, error in (no error)=w1627) -> (element=w1629:T10)  [unwired: 3 out]
            n553 = formula code="if (pos < 70)\ny = 43;\n\nelse if (pos >= 71 &&pos <= 80)\ny = 40;\n\nelse if (pos >= 81 &&pos <= 120)\ny = 35;\n\nelse if (pos >= 121 && pos <= 140)\ny = 30;\n\nelse if (pos >= 141 && pos <= 170)\ny = 26;\n\nelse if (pos >= 171 &&pos <= 200) \ny = 20;\n\nelse if (pos >= 201&& pos <= 210)\ny = 15;\n\nelse if (pos >= 211 && pos <= 230)\ny = 10;\n\nelse if (pos >= 231)\ny = 0;"("pos"=w1617) -> ("y"=w1620:dbl)
            n554 = To Unsigned Byte Integer(number=w1620) -> (unsigned 8bit integer=w1615:u8)
            "Correcte stepper" <- w1615
            n555 = Equal?(x=w1616, y=w1615) -> (x = y?=w1614:bool)
            n556 = case shown="\"None\", Default" w1629 {
              tunnel: [w1636 State_Type_Definitions,_for_0.26g_versions_and_later_2."True Stop" ("Enum")] -> w1623
              tunnel: [w1639 w1656] -> w1621
              tunnel: [State_Type_Definitions,_for_0.26g_versions_and_later_2."Idle" ("Enum") State_Type_Definitions,_for_0.26g_versions_and_later_2."Shutdown" ("Enum")] -> w1622
              tunnel: w1628 -> [w1635 _]
              tunnel: w1624 -> [w1631 w1653]
              tunnel: w1614 -> [w1630 _]
              frame "None", Default {
                # ">> T: Breaks out of state loop; F: Stays in loop>>"
                # ">> Manual override >>"
                # ">> Checks if time is up>>"
                # "Stays in Task 5D until the object is detected"
                # "T: Go back to idle, F: Continue with task\""
                # ">> Manual override >>"
                n557 = case shown="False" w1630 {
                  tunnel: [w1643 w1649] -> w1639
                  tunnel: w1631 -> [w1641 w1647]
                  frame False {
                    n558 = for {
                      tunnel: string[] ["READ STEPPER VALUES", "Y STEPPER CONTROL", ""] ("element") -> [w1644] mode=indexing
                      shift-right: [w1646] -> w1643
                      shift-left: w1641 -> [w1645]
                      n559 = Enqueue Element(queue=w1645, element=w1644) -> (queue out=w1646:refnum<queue>)  [unwired: 2 in, 2 out]
                    }
                  }
                  frame True {
                    n560 = for {
                      shift-right: [w1651] -> w1649
                      shift-left: w1647 -> [w1652]
                      tunnel: string[] ["DISPOSE BUFFERS", "READ STEPPER VALUES", ""] -> [w1650] mode=indexing
                      n561 = Enqueue Element(queue=w1652, element=w1650) -> (queue out=w1651:refnum<queue>)  [unwired: 2 in, 2 out]
                    }
                  }
                }
                n562 = Or(x=w1630, y=w1635) -> (x .or. y?=w1637:bool)
                n563 = Select(t=State_Type_Definitions,_for_0.26g_versions_and_later_2."True Stop" ("Enum"), s=w1635, f=State_Type_Definitions,_for_0.26g_versions_and_later_2."Task 8I: ARM GRAB HEIGHT" ("Enum")) -> (s? t:f=w1632:T9)
                n564 = Select(t=w1632, s=w1637, f=State_Type_Definitions,_for_0.26g_versions_and_later_2."Task 8H: ARM ADJUST" ("Enum")) -> (s? t:f=w1636:T9)
              }
              frame "Exit" {
                n565 = for {
                  shift-right: [w1659] -> w1656
                  shift-left: w1653 -> [w1660]
                  tunnel: string[] ["STOP", "RESET ENCODERS", "RESET YAW", "ARDUINO MODE 0"] -> [w1658] mode=indexing
                  n566 = Enqueue Element(queue=w1660, element=w1658) -> (queue out=w1659:refnum<queue>)  [unwired: 2 in, 2 out]
                }
              }
            }
            n567 = Bundle By Name(cluster=w1619, "yStepper desired"=w1615) -> (w1618:T14)
          }
          frame 35 {
            # ">>> Motor control cluster >>>"
            # ">>> yStepper command>>>"
            # ">> Manual override >>"
            n568 = Dequeue Element(queue=w1670, timeout in ms (-1)=w1669, error in (no error)=w1671) -> (element=w1668:T10)  [unwired: 3 out]
            n569 = Equal?(x=w1667, y=u8 1) -> (x = y?=w1665:bool)
            n570 = case shown="\"None\", Default" w1668 {
              tunnel: [w1681 State_Type_Definitions,_for_0.26g_versions_and_later_2."True Stop" ("Enum")] -> w1672
              tunnel: [w1684 w1701] -> w1673
              tunnel: [State_Type_Definitions,_for_0.26g_versions_and_later_2."Idle" ("Enum") State_Type_Definitions,_for_0.26g_versions_and_later_2."Shutdown" ("Enum")] -> w1674
              tunnel: w1665 -> [w1680 _]
              tunnel: w1664 -> [w1679 _]
              tunnel: w1663 -> [w1675 w1698]
              frame "None", Default {
                # "Stays in Task 5F until stepper reaches desired \nheight"
                # "T: Go back to idle, F: Continue with task\""
                # ">> Manual override >>"
                n571 = case shown="True" w1680 {
                  tunnel: [w1688 w1694] -> w1684
                  tunnel: w1675 -> [w1686 w1692]
                  frame False {
                    n572 = for {
                      tunnel: string[] ["Z STEPPER GRAB HEIGHT", "READ STEPPER VALUES"] ("element") -> [w1689] mode=indexing
                      shift-right: [w1691] -> w1688
                      shift-left: w1686 -> [w1690]
                      n573 = Enqueue Element(queue=w1690, element=w1689) -> (queue out=w1691:refnum<queue>)  [unwired: 2 in, 2 out]
                    }
                  }
                  frame True {
                    n574 = for {
                      shift-right: [w1696] -> w1694
                      shift-left: w1692 -> [w1697]
                      tunnel: string[] ["SET TIMER 2", "CLOSE CLAW", ""] -> [w1695] mode=indexing
                      n575 = Enqueue Element(queue=w1697, element=w1695) -> (queue out=w1696:refnum<queue>)  [unwired: 2 in, 2 out]
                    }
                  }
                }
                n576 = Or(x=w1680, y=w1679) -> (x .or. y?=w1682:bool)
                n577 = Select(t=State_Type_Definitions,_for_0.26g_versions_and_later_2."True Stop" ("Enum"), s=w1679, f=State_Type_Definitions,_for_0.26g_versions_and_later_2."Task 8J: CLOSE CLAW" ("Enum")) -> (s? t:f=w1676:T9)
                n578 = Select(t=w1676, s=w1682, f=State_Type_Definitions,_for_0.26g_versions_and_later_2."Task 8I: ARM GRAB HEIGHT" ("Enum")) -> (s? t:f=w1681:T9)
              }
              frame "Exit" {
                n579 = for {
                  shift-right: [w1704] -> w1701
                  shift-left: w1698 -> [w1705]
                  tunnel: string[] ["STOP", "RESET ENCODERS", "RESET YAW", "ARDUINO MODE 0"] -> [w1703] mode=indexing
                  n580 = Enqueue Element(queue=w1705, element=w1703) -> (queue out=w1704:refnum<queue>)  [unwired: 2 in, 2 out]
                }
              }
            }
          }
          frame 36 {
            # ">>> yStepper command>>>"
            # ">> Manual override >>"
            n581 = Dequeue Element(queue=w1715, timeout in ms (-1)=w1714, error in (no error)=w1713) -> (element=w1712:T10)  [unwired: 3 out]
            n582 = case shown="\"None\", Default" w1712 {
              tunnel: [w1724 State_Type_Definitions,_for_0.26g_versions_and_later_2."True Stop" ("Enum")] -> w1717
              tunnel: [w1727 w1744] -> w1710
              tunnel: [State_Type_Definitions,_for_0.26g_versions_and_later_2."Idle" ("Enum") State_Type_Definitions,_for_0.26g_versions_and_later_2."Shutdown" ("Enum")] -> w1709
              tunnel: w1711 -> [w1718 _]
              tunnel: w1716 -> [w1723 w1741]
              tunnel: w1707 -> [w1722 _]
              frame "None", Default {
                # ">> Is time up? >>"
                # "Determines if object is in range to pick up"
                # ">> Manual override >>"
                n583 = case shown="True" w1722 {
                  tunnel: [w1731 w1737] -> w1727
                  tunnel: w1723 -> [w1729 w1735]
                  frame False {
                    n584 = for {
                      tunnel: string[] ["CLOSE CLAW", "START TIMER"] ("element") -> [w1732] mode=indexing
                      shift-right: [w1734] -> w1731
                      shift-left: w1729 -> [w1733]
                      n585 = Enqueue Element(queue=w1733, element=w1732) -> (queue out=w1734:refnum<queue>)  [unwired: 2 in, 2 out]
                    }
                  }
                  frame True {
                    n586 = for {
                      shift-right: [w1739] -> w1737
                      shift-left: w1735 -> [w1740]
                      tunnel: string[] ["READ STEPPER VALUES", "", ""] -> [w1738] mode=indexing
                      n587 = Enqueue Element(queue=w1740, element=w1738) -> (queue out=w1739:refnum<queue>)  [unwired: 2 in, 2 out]
                    }
                  }
                }
                n588 = Or(x=w1722, y=w1718) -> (x .or. y?=w1725:bool)
                n589 = Select(t=State_Type_Definitions,_for_0.26g_versions_and_later_2."True Stop" ("Enum"), s=w1718, f=State_Type_Definitions,_for_0.26g_versions_and_later_2."Task 8K: RAISE MY SWORD" ("Enum")) -> (s? t:f=w1720:T9)
                n590 = Select(t=w1720, s=w1725, f=State_Type_Definitions,_for_0.26g_versions_and_later_2."Task 8J: CLOSE CLAW" ("Enum")) -> (s? t:f=w1724:T9)
              }
              frame "Exit" {
                n591 = for {
                  shift-right: [w1747] -> w1744
                  shift-left: w1741 -> [w1748]
                  tunnel: string[] ["STOP", "RESET ENCODERS", "RESET YAW", "ARDUINO MODE 0"] -> [w1746] mode=indexing
                  n592 = Enqueue Element(queue=w1748, element=w1746) -> (queue out=w1747:refnum<queue>)  [unwired: 2 in, 2 out]
                }
              }
            }
          }
          frame 37 {
            # ">>> yStepper command>>>"
            # ">> Manual override >>"
            n593 = Dequeue Element(queue=w1758, timeout in ms (-1)=w1757, error in (no error)=w1759) -> (element=w1756:T10)  [unwired: 3 out]
            n594 = Equal?(x=w1755, y=u8 60) -> (x = y?=w1753:bool)
            n595 = case shown="\"None\", Default" w1756 {
              tunnel: [w1769 State_Type_Definitions,_for_0.26g_versions_and_later_2."True Stop" ("Enum")] -> w1760
              tunnel: [w1772 w1789] -> w1761
              tunnel: [State_Type_Definitions,_for_0.26g_versions_and_later_2."Idle" ("Enum") State_Type_Definitions,_for_0.26g_versions_and_later_2."Shutdown" ("Enum")] -> w1762
              tunnel: w1753 -> [w1768 _]
              tunnel: w1752 -> [w1767 _]
              tunnel: w1751 -> [w1763 w1786]
              frame "None", Default {
                # "Stays in Task 5_A until stepper reaches desired \nheight"
                # "T: Go back to idle, F: Continue with task\""
                # ">> Manual override >>"
                n596 = case shown="True" w1768 {
                  tunnel: [w1776 w1782] -> w1772
                  tunnel: w1763 -> [w1774 w1780]
                  frame False {
                    n597 = for {
                      tunnel: string[] ["Z STEPPER CAM HEIGHT", "READ STEPPER VALUES"] ("element") -> [w1777] mode=indexing
                      shift-right: [w1779] -> w1776
                      shift-left: w1774 -> [w1778]
                      n598 = Enqueue Element(queue=w1778, element=w1777) -> (queue out=w1779:refnum<queue>)  [unwired: 2 in, 2 out]
                    }
                  }
                  frame True {
                    n599 = for {
                      shift-right: [w1784] -> w1782
                      shift-left: w1780 -> [w1785]
                      tunnel: string[] ["CAM CLOSE", "DISPOSE ALL BUFFERS", ""] -> [w1783] mode=indexing
                      n600 = Enqueue Element(queue=w1785, element=w1783) -> (queue out=w1784:refnum<queue>)  [unwired: 2 in, 2 out]
                    }
                  }
                }
                n601 = Or(x=w1768, y=w1767) -> (x .or. y?=w1770:bool)
                n602 = Select(t=State_Type_Definitions,_for_0.26g_versions_and_later_2."True Stop" ("Enum"), s=w1767, f=State_Type_Definitions,_for_0.26g_versions_and_later_2."True Stop" ("Enum")) -> (s? t:f=w1764:T9)
                n603 = Select(t=w1764, s=w1770, f=State_Type_Definitions,_for_0.26g_versions_and_later_2."Task 8K: RAISE MY SWORD" ("Enum")) -> (s? t:f=w1769:T9)
              }
              frame "Exit" {
                n604 = for {
                  shift-right: [w1792] -> w1789
                  shift-left: w1786 -> [w1793]
                  tunnel: string[] ["STOP", "RESET ENCODERS", "RESET YAW", "ARDUINO MODE 0"] -> [w1791] mode=indexing
                  n605 = Enqueue Element(queue=w1793, element=w1791) -> (queue out=w1792:refnum<queue>)  [unwired: 2 in, 2 out]
                }
              }
            }
          }
          frame 38 {
            # ">> Stepper height reeached >>"
            # ">>> yStepper command>>>"
            # ">> Manual override >>"
            n606 = Dequeue Element(queue=w1804, timeout in ms (-1)=w1799, error in (no error)=w1803) -> (element=w1807:T10)  [unwired: 3 out]
            n607 = Equal?(x=w1801, y=u8 40) -> (x = y?=w1805:bool)
            n608 = case shown="\"None\", Default" w1807 {
              tunnel: [w1818 State_Type_Definitions,_for_0.26g_versions_and_later_2."True Stop" ("Enum")] -> w1797
              tunnel: [w1816 w1833] -> w1796
              tunnel: w1800 -> [w1815 _]
              tunnel: w1802 -> [w1809 _]
              tunnel: [State_Type_Definitions,_for_0.26g_versions_and_later_2."Idle" ("Enum") State_Type_Definitions,_for_0.26g_versions_and_later_2."Shutdown" ("Enum")] -> w1798
              tunnel: w1805 -> [w1808 _]
              frame "None", Default {
                # ">> WIill proceed to part ii if not manual override >>"
                # ">>If ENABLE or Trigger is set to true>>"
                n609 = Or(x=w1808, y=w1809) -> (x .or. y?=w1810:bool)
                n610 = case shown="False" w1808 {
                  tunnel: [w1821 w1827] -> w1816
                  tunnel: w1815 -> [w1820 w1826]
                  frame False {
                    n611 = for {
                      shift-right: [w1823] -> w1821
                      shift-left: w1820 -> [w1824]
                      tunnel: string[] ["Z STEPPER BOX HEIGHT", "READ STEPPER VALUES"] ("element") -> [w1822] mode=indexing
                      n612 = Enqueue Element(queue=w1824, element=w1822) -> (queue out=w1823:refnum<queue>)  [unwired: 2 in, 2 out]
                    }
                  }
                  frame True {
                    n613 = for {
                      shift-right: [w1829] -> w1827
                      shift-left: w1826 -> [w1830]
                      tunnel: string[] ["ARDUINO - ULTRASONIC", "READ ULTRASONIC", "", "", "", ""] -> [w1828] mode=indexing
                      n614 = Enqueue Element(queue=w1830, element=w1828) -> (queue out=w1829:refnum<queue>)  [unwired: 2 in, 2 out]
                    }
                  }
                }
                n615 = Select(t=State_Type_Definitions,_for_0.26g_versions_and_later_2."True Stop" ("Enum"), s=w1809, f=State_Type_Definitions,_for_0.26g_versions_and_later_2."Task 9B: Rotate to Angle" ("Enum")) -> (s? t:f=w1812:T9)
                n616 = Select(t=w1812, s=w1810, f=State_Type_Definitions,_for_0.26g_versions_and_later_2."Task 9A: Raise Arm" ("Enum")) -> (s? t:f=w1818:T9)
              }
              frame "Exit" {
                n617 = for {
                  shift-right: [w1836] -> w1833
                  shift-left: _ -> [w1837]
                  tunnel: string[] ["STOP", "RESET ENCODERS", "RESET YAW", ""] -> [w1835] mode=indexing
                  n618 = Enqueue Element(queue=w1837, element=w1835) -> (queue out=w1836:refnum<queue>)  [unwired: 2 in, 2 out]
                }
              }
            }
          }
          frame 39 {
            # ">>> yStepper command>>>"
            n619 = Dequeue Element(queue=w1850, timeout in ms (-1)=w1849, error in (no error)=w1848) -> (element=w1852:T10)  [unwired: 3 out]
            n620 = In Range and Coerce(upper limit=65.0, x=w1842, lower limit=55.0) -> (In Range?=w1839:bool)  [unwired: 1 out]
            n621 = case shown="\"None\", Default" w1852 {
              tunnel: w1843 -> [w1855 _]
              tunnel: [w1863 State_Type_Definitions,_for_0.26g_versions_and_later_2."True Stop" ("Enum")] -> w1845
              tunnel: w1851 -> [w1861 w1879]
              tunnel: [w1860 w1878] -> w1844
              tunnel: [State_Type_Definitions,_for_0.26g_versions_and_later_2."Idle" ("Enum") State_Type_Definitions,_for_0.26g_versions_and_later_2."Shutdown" ("Enum")] -> w1846
              tunnel: w1839 -> [w1853 _]
              frame "None", Default {
                n622 = Or(x=w1853, y=w1855) -> (x .or. y?=w1854:bool)
                n623 = case shown="True" w1853 {
                  tunnel: w1861 -> [w1866 w1872]
                  tunnel: [w1865 w1870] -> w1860
                  frame False {
                    n624 = for {
                      shift-right: [w1868] -> w1865
                      shift-left: w1866 -> [w1869]
                      tunnel: string[] ["READ NAVX", "R-ACW"] ("element") -> [w1867] mode=indexing
                      n625 = Enqueue Element(queue=w1869, element=w1867) -> (queue out=w1868:refnum<queue>)  [unwired: 2 in, 2 out]
                    }
                  }
                  frame True {
                    n626 = for {
                      shift-right: [w1874] -> w1870
                      shift-left: w1872 -> [w1875]
                      tunnel: string[] ["STOP", "RESET ENCODERS", "RESET YAW", ""] -> [w1873] mode=indexing
                      n627 = Enqueue Element(queue=w1875, element=w1873) -> (queue out=w1874:refnum<queue>)  [unwired: 2 in, 2 out]
                    }
                  }
                }
                n628 = Select(t=State_Type_Definitions,_for_0.26g_versions_and_later_2."True Stop" ("Enum"), s=w1855, f=State_Type_Definitions."Task 9C: Rotation alignmnet") -> (s? t:f=w1857:u16)
                n629 = Select(t=w1857, s=w1854, f=State_Type_Definitions,_for_0.26g_versions_and_later_2."Task 9B: Rotate to Angle" ("Enum")) -> (s? t:f=w1863:u16)
              }
              frame "Exit" {
                n630 = for {
                  shift-right: [w1882] -> w1878
                  shift-left: w1879 -> [w1883]
                  tunnel: string[] ["STOP", "RESET ENCODERS", "RESET YAW", ""] -> [w1881] mode=indexing
                  n631 = Enqueue Element(queue=w1883, element=w1881) -> (queue out=w1882:refnum<queue>)  [unwired: 2 in, 2 out]
                }
              }
            }
          }
          frame 39 {
            # ">>> Motor control cluster >>>"
            # ">>Line Detected>>"
            # ">>Action Queue>>"
            # ">>> yStepper command>>>"
            n632 = Dequeue Element(queue=w1894, timeout in ms (-1)=w1893, error in (no error)=w1892) -> (element=w1895:T10)  [unwired: 3 out]
            n633 = case shown="\"None\", Default" w1895 {
              tunnel: w1890 -> [w1896 _]
              tunnel: [w1906 State_Type_Definitions,_for_0.26g_versions_and_later_2."True Stop" ("Enum")] -> w1887
              tunnel: w1891 -> [w1904 w1922]
              tunnel: [w1903 w1921] -> w1886
              tunnel: [State_Type_Definitions,_for_0.26g_versions_and_later_2."Idle" ("Enum") State_Type_Definitions,_for_0.26g_versions_and_later_2."Shutdown" ("Enum")] -> w1889
              tunnel: w1884 -> [w1897 _]
              frame "None", Default {
                n634 = Or(x=w1896, y=w1897) -> (x .or. y?=w1898:bool)
                n635 = case shown="True" w1897 {
                  tunnel: w1904 -> [w1909 w1915]
                  tunnel: [w1908 w1913] -> w1903
                  frame False {
                    n636 = for {
                      shift-right: [w1911] -> w1908
                      shift-left: w1909 -> [w1912]
                      tunnel: string[] ["READ IR", "READ LINE SENSOR", "FORWARD - IR ASSIST"] ("element") -> [w1910] mode=indexing
                      n637 = Enqueue Element(queue=w1912, element=w1910) -> (queue out=w1911:refnum<queue>)  [unwired: 2 in, 2 out]
                    }
                  }
                  frame True {
                    n638 = for {
                      shift-right: [w1917] -> w1913
                      shift-left: w1915 -> [w1918]
                      tunnel: string[] ["STOP", "RESET ENCODERS", "RESET YAW", ""] -> [w1916] mode=indexing
                      n639 = Enqueue Element(queue=w1918, element=w1916) -> (queue out=w1917:refnum<queue>)  [unwired: 2 in, 2 out]
                    }
                  }
                }
                n640 = Select(t=State_Type_Definitions,_for_0.26g_versions_and_later_2."True Stop" ("Enum"), s=w1896, f=State_Type_Definitions."Task 9D: Move Forward") -> (s? t:f=w1900:u16)
                n641 = Select(t=w1900, s=w1898, f=State_Type_Definitions."Task 9C: Rotation alignmnet" ("Enum")) -> (s? t:f=w1906:u16)
              }
              frame "Exit" {
                n642 = for {
                  shift-right: [w1925] -> w1921
                  shift-left: w1922 -> [w1926]
                  tunnel: string[] ["STOP", "RESET ENCODERS", "RESET YAW", ""] -> [w1924] mode=indexing
                  n643 = Enqueue Element(queue=w1926, element=w1924) -> (queue out=w1925:refnum<queue>)  [unwired: 2 in, 2 out]
                }
              }
            }
          }
          frame 40 {
            # ">> Manual override >>"
            # ">>Table Detected>>"
            # ">>> Motor control cluster >>>"
            # ">>Line Detected>>"
            # ">>Action Queue>>"
            # ">>> yStepper command>>>"
            n644 = Less Or Equal?(x=w1928, y=15.0) -> (x <= y?=w1927:bool)
            n645 = Dequeue Element(queue=w1939, timeout in ms (-1)=w1938, error in (no error)=w1937) -> (element=w1940:T10)  [unwired: 3 out]
            n646 = case shown="\"None\", Default" w1940 {
              tunnel: w1935 -> [w1941 _]
              tunnel: [w1951 State_Type_Definitions,_for_0.26g_versions_and_later_2."True Stop" ("Enum")] -> w1932
              tunnel: w1936 -> [w1949 w1967]
              tunnel: [w1948 w1966] -> w1931
              tunnel: [State_Type_Definitions,_for_0.26g_versions_and_later_2."Idle" ("Enum") State_Type_Definitions,_for_0.26g_versions_and_later_2."Shutdown" ("Enum")] -> w1934
              tunnel: w1927 -> [w1942 _]
              frame "None", Default {
                n647 = Or(x=w1941, y=w1942) -> (x .or. y?=w1943:bool)
                n648 = case shown="True" w1942 {
                  tunnel: w1949 -> [w1954 w1960]
                  tunnel: [w1953 w1958] -> w1948
                  frame False {
                    n649 = for {
                      shift-right: [w1956] -> w1953
                      shift-left: w1954 -> [w1957]
                      tunnel: string[] ["READ IR", "FORWARD - IR ASSIST", ""] ("element") -> [w1955] mode=indexing
                      n650 = Enqueue Element(queue=w1957, element=w1955) -> (queue out=w1956:refnum<queue>)  [unwired: 2 in, 2 out]
                    }
                  }
                  frame True {
                    n651 = for {
                      shift-right: [w1962] -> w1958
                      shift-left: w1960 -> [w1963]
                      tunnel: string[] ["STOP", "RESET ENCODERS", "RESET YAW", ""] -> [w1961] mode=indexing
                      n652 = Enqueue Element(queue=w1963, element=w1961) -> (queue out=w1962:refnum<queue>)  [unwired: 2 in, 2 out]
                    }
                  }
                }
                n653 = Select(t=State_Type_Definitions,_for_0.26g_versions_and_later_2."True Stop" ("Enum"), s=w1941, f=State_Type_Definitions,_for_0.26g_versions_and_later_2."Task 9E: MOVE LEFT") -> (s? t:f=w1945:T9)
                n654 = Select(t=w1945, s=w1943, f=State_Type_Definitions."Task 9D: Move Forward" ("Enum")) -> (s? t:f=w1951:u16)
              }
              frame "Exit" {
                n655 = for {
                  shift-right: [w1970] -> w1966
                  shift-left: w1967 -> [w1971]
                  tunnel: string[] ["STOP", "RESET ENCODERS", "RESET YAW", ""] -> [w1969] mode=indexing
                  n656 = Enqueue Element(queue=w1971, element=w1969) -> (queue out=w1970:refnum<queue>)  [unwired: 2 in, 2 out]
                }
              }
            }
          }
          frame 42 {
            # ">> Reached distance?>>"
            # ">> Manual override >>"
            # ">>> Motor control cluster >>>"
            # ">>Action Queue>>"
            # ">>> yStepper command>>>"
            n657 = Dequeue Element(queue=w1984, timeout in ms (-1)=w1983, error in (no error)=w1982) -> (element=w1985:T10)  [unwired: 3 out]
            n658 = Less Or Equal?(x=w1974, y=-30.0) -> (x <= y?=w1972:bool)
            "Distance reached?" <- w1972
            n659 = case shown="\"None\", Default" w1985 {
              tunnel: w1980 -> [w1986 _]
              tunnel: [w1996 State_Type_Definitions,_for_0.26g_versions_and_later_2."True Stop" ("Enum")] -> w1977
              tunnel: w1981 -> [w1994 w2012]
              tunnel: [w1993 w2011] -> w1976
              tunnel: [State_Type_Definitions,_for_0.26g_versions_and_later_2."Idle" ("Enum") State_Type_Definitions,_for_0.26g_versions_and_later_2."Shutdown" ("Enum")] -> w1979
              tunnel: w1972 -> [w1987 _]
              frame "None", Default {
                n660 = Or(x=w1986, y=w1987) -> (x .or. y?=w1988:bool)
                n661 = case shown="False" w1987 {
                  tunnel: w1994 -> [w1999 w2005]
                  tunnel: [w1998 w2003] -> w1993
                  frame False {
                    n662 = for {
                      shift-right: [w2001] -> w1998
                      shift-left: w1999 -> [w2002]
                      tunnel: string[] ["LEFT", "READ NAVX", "READ ENCODERS"] ("element") -> [w2000] mode=indexing
                      n663 = Enqueue Element(queue=w2002, element=w2000) -> (queue out=w2001:refnum<queue>)  [unwired: 2 in, 2 out]
                    }
                  }
                  frame True {
                    n664 = for {
                      shift-right: [w2007] -> w2003
                      shift-left: w2005 -> [w2008]
                      tunnel: string[] ["STOP", "RESET ENCODERS", "RESET YAW", ""] -> [w2006] mode=indexing
                      n665 = Enqueue Element(queue=w2008, element=w2006) -> (queue out=w2007:refnum<queue>)  [unwired: 2 in, 2 out]
                    }
                  }
                }
                n666 = Select(t=State_Type_Definitions,_for_0.26g_versions_and_later_2."True Stop" ("Enum"), s=w1986, f=State_Type_Definitions,_for_0.26g_versions_and_later_2."True Stop") -> (s? t:f=w1990:T9)
                n667 = Select(t=w1990, s=w1988, f=State_Type_Definitions,_for_0.26g_versions_and_later_2."Task 9E: MOVE LEFT" ("Enum")) -> (s? t:f=w1996:T9)
              }
              frame "Exit" {
                n668 = for {
                  shift-right: [w2015] -> w2011
                  shift-left: w2012 -> [w2016]
                  tunnel: string[] ["STOP", "RESET ENCODERS", "RESET YAW", ""] -> [w2014] mode=indexing
                  n669 = Enqueue Element(queue=w2016, element=w2014) -> (queue out=w2015:refnum<queue>)  [unwired: 2 in, 2 out]
                }
              }
            }
          }
          frame 42 {
            # ">> Stepper height reeached >>"
            # ">>> yStepper command>>>"
            # ">> Manual override >>"
            n670 = Dequeue Element(queue=w2027, timeout in ms (-1)=w2022, error in (no error)=w2026) -> (element=w2030:T10)  [unwired: 3 out]
            n671 = Equal?(x=w2024, y=u8 40) -> (x = y?=w2028:bool)
            n672 = case shown="\"None\", Default" w2030 {
              tunnel: [w2041 State_Type_Definitions,_for_0.26g_versions_and_later_2."True Stop" ("Enum")] -> w2020
              tunnel: [w2039 w2057] -> w2019
              tunnel: w2023 -> [w2038 w2054]
              tunnel: w2025 -> [w2032 _]
              tunnel: [State_Type_Definitions,_for_0.26g_versions_and_later_2."Idle" ("Enum") State_Type_Definitions,_for_0.26g_versions_and_later_2."Shutdown" ("Enum")] -> w2021
              tunnel: w2028 -> [w2031 _]
              frame "None", Default {
                # ">> WIill proceed to part ii if not manual override >>"
                # ">>If ENABLE or Trigger is set to true>>"
                n673 = Or(x=w2031, y=w2032) -> (x .or. y?=w2033:bool)
                n674 = case shown="False" w2031 {
                  tunnel: [w2044 w2050] -> w2039
                  tunnel: w2038 -> [w2043 w2049]
                  frame False {
                    n675 = for {
                      shift-right: [w2046] -> w2044
                      shift-left: w2043 -> [w2047]
                      tunnel: string[] ["Z STEPPER BOX HEIGHT", "READ STEPPER VALUES"] ("element") -> [w2045] mode=indexing
                      n676 = Enqueue Element(queue=w2047, element=w2045) -> (queue out=w2046:refnum<queue>)  [unwired: 2 in, 2 out]
                    }
                  }
                  frame True {
                    n677 = for {
                      shift-right: [w2052] -> w2050
                      shift-left: w2049 -> [w2053]
                      tunnel: string[] ["READ IR", "", "", "", "", ""] -> [w2051] mode=indexing
                      n678 = Enqueue Element(queue=w2053, element=w2051) -> (queue out=w2052:refnum<queue>)  [unwired: 2 in, 2 out]
                    }
                  }
                }
                n679 = Select(t=State_Type_Definitions,_for_0.26g_versions_and_later_2."True Stop" ("Enum"), s=w2032, f=State_Type_Definitions."Task A: MOVE FORWARD" ("Enum")) -> (s? t:f=w2035:u16)
                n680 = Select(t=w2035, s=w2033, f=State_Type_Definitions."Task A: RAISE ARM TO HEIGHT" ("Enum")) -> (s? t:f=w2041:u16)
              }
              frame "Exit" {
                n681 = for {
                  shift-right: [w2060] -> w2057
                  shift-left: w2054 -> [w2061]
                  tunnel: string[] ["STOP", "RESET ENCODERS", "RESET YAW", ""] -> [w2059] mode=indexing
                  n682 = Enqueue Element(queue=w2061, element=w2059) -> (queue out=w2060:refnum<queue>)  [unwired: 2 in, 2 out]
                }
              }
            }
          }
          frame 43 {
            # ">>> Motor control cluster >>>"
            # ">>> yStepper command>>>"
            # ">>Object detected>>"
            n683 = Dequeue Element(queue=w2070, timeout in ms (-1)=w2069, error in (no error)=w2068) -> (element=w2075:T10)  [unwired: 3 out]
            n684 = Less Or Equal?(x=w2064, y=30.0) -> (x <= y?=w2062:bool)
            "Table obstruct" <- w2062
            n685 = case shown="\"None\", Default" w2075 {
              tunnel: w2062 -> [w2078 _]
              tunnel: [w2085 State_Type_Definitions,_for_0.26g_versions_and_later_2."True Stop" ("Enum")] -> w2074
              tunnel: w2067 -> [w2077 _]
              tunnel: w2071 -> [w2084 w2101]
              tunnel: [w2083 w2102] -> w2073
              tunnel: [State_Type_Definitions,_for_0.26g_versions_and_later_2."Idle" ("Enum") State_Type_Definitions,_for_0.26g_versions_and_later_2."Shutdown" ("Enum")] -> w2072
              frame "None", Default {
                n686 = case shown="False" w2078 {
                  tunnel: w2084 -> [w2088 w2095]
                  tunnel: [w2089 w2094] -> w2083
                  frame False {
                    n687 = for {
                      tunnel: string[] ["READ IR", "FORWARD", "READ NAVX"] ("element") -> [w2090] mode=indexing
                      shift-right: [w2092] -> w2089
                      shift-left: w2088 -> [w2091]
                      n688 = Enqueue Element(queue=w2091, element=w2090) -> (queue out=w2092:refnum<queue>)  [unwired: 2 in, 2 out]
                    }
                  }
                  frame True {
                    n689 = for {
                      shift-right: [w2097] -> w2094
                      shift-left: w2095 -> [w2098]
                      tunnel: string[] ["RESET ENCODERS", "READ NAVX", "READ ENCODERS"] -> [w2096] mode=indexing
                      n690 = Enqueue Element(queue=w2098, element=w2096) -> (queue out=w2097:refnum<queue>)  [unwired: 2 in, 2 out]
                    }
                  }
                }
                n691 = Or(x=w2078, y=w2077) -> (x .or. y?=w2076:bool)
                n692 = Select(t=State_Type_Definitions,_for_0.26g_versions_and_later_2."True Stop" ("Enum"), s=w2077, f=State_Type_Definitions,_for_0.26g_versions_and_later_2."True Stop" ("Enum")) -> (s? t:f=w2079:T9)
                n693 = Select(t=w2079, s=w2076, f=State_Type_Definitions."Task A: MOVE FORWARD" ("Enum")) -> (s? t:f=w2085:u16)
              }
              frame "Exit" {
                n694 = for {
                  shift-right: [w2105] -> w2102
                  shift-left: w2101 -> [w2106]
                  tunnel: string[] ["STOP", "RESET ENCODERS", "RESET YAW", "ARDUINO MODE 0"] -> [w2104] mode=indexing
                  n695 = Enqueue Element(queue=w2106, element=w2104) -> (queue out=w2105:refnum<queue>)  [unwired: 2 in, 2 out]
                }
              }
            }
          }
        }
        "Object Detection" <- w282
      }
    }
    n696 = local write "Green LED"(w207) -> ()
  }
  n697 = while {
    stop <- w2764 stop-if-true
    n698 = call "MOTOR CONTROL WITH PID AE.vi"("AE Mode"=MOTOR_CONTROL_WITH_PID_AE_DATA_MODE_TYPE_DEF."Read from AE") -> ("Speed & distance"=→"Speed & distance":T5)  [unwired: 3 in]
    n699 = call "FGV Bool.vi"("Init/Read/Write State"=States_for_Action_Engine."Read") -> ("Output node"=w2764:bool)  [unwired: 2 in, 1 out]
    n700 = Wait (ms)(milliseconds to wait=u32 5) -> ()  [unwired: 1 out]
  }
  n701 = while {
    stop <- w2769 stop-if-true
    n702 = call <vilib>:"RT Get CPU Loads.vi"() -> ("CPU loads"=→"CPU loads":T8[])  [unwired: 10 in, 1 out]
    n703 = Wait (ms)(milliseconds to wait=u32 100) -> ()  [unwired: 1 out]
    n704 = call "FGV Bool.vi"("Init/Read/Write State"=States_for_Action_Engine."Read") -> ("Output node"=w2769:bool)  [unwired: 2 in, 1 out]
  }
  n705 = call <vilib>:"DIO Close.vi"("error in (no error)"=w22, "DIO Info In"=w25) -> ()  [unwired: 9 in, 1 out]
  n706 = call <vilib>:"DIO Close.vi"("error in (no error)"=w32, "DIO Info In"=w34) -> ()  [unwired: 9 in, 1 out]
  n707 = call <vilib>:"NavX Close.vi"("error in (no error)"=w9, "NavX Info In"=w8) -> ()  [unwired: 9 in, 1 out]
  n708 = call <vilib>:"DIO Close.vi"("error in (no error)"=w27, "DIO Info In"=w29) -> ()  [unwired: 9 in, 1 out]
  n709 = call <vilib>:"DIO Close.vi"("error in (no error)"=w16, "DIO Info In"=w17) -> ()  [unwired: 9 in, 1 out]
  n710 = call <vilib>:"DIO Close.vi"("error in (no error)"=w11, "DIO Info In"=w12) -> ()  [unwired: 9 in, 1 out]
  n711 = Merge Errors "Merge Errors"(w62, w61) -> (w44:errorcluster)
  n712 = Merge Errors(w48, w44) -> (w43:errorcluster)
  n713 = Destroy User Event(user event=w65, error in=w43) -> ()  [unwired: 1 out]
  n714 = Destroy User Event(user event=w66, error in=w43) -> ()  [unwired: 1 out]
  n715 = Unregister For Events(event registration refnum=w57, error in=w43) -> ()  [unwired: 1 out]
  n716 = Release Queue(queue=w39, error in (no error)=w43) -> (error out=→"Queue Errors":errorcluster)  [unwired: 1 in, 2 out]
  n717 = Release Queue(queue=w56, error in (no error)=w43) -> ()  [unwired: 1 in, 3 out]
